vi "Periodic Tasks.vi"(8 "error in":errorcluster) -> ()   [LabVIEW 2016]
doc: "This VI runs in parallel to other tasks. It can contain as many user-defined periodic loops as you need. These can carry out PID or other sorts of timed response."
uses:
  <userlib>/836-libraries/Drive/Drive_Code/Drive_Code_Support/Drive_Code_PID_Bundle.ctl
  <vilib>/Platform/TimedLoop/XDataNode/timing_clust.ctl
  <vilib>/Platform/TimedLoop/XDataNode/nitl_modes.ctl
  <vilib>/Platform/TimedLoop/XDataNode/wakeup.ctl
  Drive Commands.ctl
  Shooting States.ctl
  <vilib>/Rock Robotics/SystemInterfaces/DIO/FPGA_DIOChannel.ctl
  Gear Command.ctl
  TurretStates.ctl
  Control 1.ctl
  TurretImu.ctl
  <vilib>/Rock Robotics/WPI/ThirdParty/CanMotor/TalonSRX/WPI_CANTalonSRX_APIFeedbackSelect.ctl
  FMS Commands.ctl
  <userlib>/836-libraries/Drive/Drive_Code/Drive_Code_Support/Sensor_Cluster.ctl
  <userlib>/836-libraries/Drive/Drive_Code/Drive_Code_Support/Camera_Cluster.ctl
  <userlib>/836-libraries/Drive/Drive_Code/Drive_Code_Support/Drive_Code_Notifier.ctl
  <userlib>/836-libraries/Drive/Drive_Code/Drive_Code_Support/Drive_Code_Command.ctl
  <userlib>/836-libraries/Drive/Drive_Code/Logging_Data.ctl
  <userlib>/836-libraries/Pneumatics/Support_Code/Pneumatics_Command.ctl
  <userlib>/836-libraries/Pneumatics/Support_Code/Pneumatics_Status.ctl
  <userlib>/836-libraries/Pneumatics/Support_Code/Pneumatics_Position.ctl
  <vilib>/Rock Robotics/WPI/Solenoid/WPI_SolenoidDevRef.ctl
  <vilib>/Rock Robotics/WPI/Solenoid/WPI_SolenoidChannel.ctl
  <vilib>/Rock Robotics/WPI/Solenoid/WPI_SolenoidValue.ctl
  <vilib>/Rock Robotics/SystemInterfaces/AI/FPGA_AIChannel.ctl
  <vilib>/Rock Robotics/WPI/DriverStation/WPI_DriverStationRobotMode2.ctl
  MatchTimeNotifications.ctl
  <vilib>/Rock Robotics/WPI/DriverStation/WPI_DriverStationAllianceInfo.ctl
  <vilib>/Analysis/coordinate.llb/Angle Units.ctl
  <vilib>/Analysis/coordinate.llb/Angle Range (Degree).ctl
  <vilib>/Rock Robotics/WPI/ThirdParty/CanMotor/TalonSRX/WPI_CANTalonSRX_APIControlMode.ctl
  <vilib>/Analysis/coordinate.llb/Wrap Angle (scalar).vi
  <vilib>/Rock Robotics/WPI/Utilities/WPI_GetSetVariantRefNum.vi
  <vilib>/addons/control/pid/pid.llb/PID Output Rate Limiter (DBL).vi
  <userlib>/836-libraries/Drive/Drive_Code/Drive_Code_Support/Drive_Loop_Turn_to_Camera.vi
  <userlib>/836-libraries/Drive/Drive_Code/Drive_Code_Support/Drive_Loop_Cheesey_Drive.vi
  <userlib>/836-libraries/Drive/Drive_Code/Drive_Code_Support/Drive_Loop_Turn.vi
  <userlib>/836-libraries/Drive/Drive_Code/Drive_Code_Support/Drive_Loop_Drive_Distance.vi
  <vilib>/addons/control/pid/pid.llb/PID (DBL).vi
  <userlib>/836-libraries/Drive/Drive_Code/Drive_Code_Support/Drive_Loop_Do_Nothing.vi
  <userlib>/836-libraries/Drive/Drive_Code/Drive_Code_Support/Drive_Loop_Follow_Camera.vi
  <userlib>/836-libraries/Drive/Drive_Code/Drive_Code_Support/Drive_Loop_Tank_Drive.vi
  <userlib>/836-libraries/Pneumatics/Support_Code/Pneumatics_Command_Set_Periodic.vi
  <vilib>/Rock Robotics/Network Tables/NT Write Number.vi
  <vilib>/platform/TimedLoop/XDataNode/XDataNode.xnode
  <vilib>/Platform/TimedLoop/XDataNode/XDNodeRunTimeDep.lvlib
  <vilib>/Analysis/NI_AAL_Angle.lvlib
  <vilib>/addons/control/pid/NI_PID_pid.lvlib
  <userlib>/836-libraries/Drive/Drive_Code/Drive_Code_Support/Drive_Loop_Approach_Camera.vi
panel:
  in  "Modulate?":bool
  out "Sensor Loop Duration? 2":i64=6
  out "Sensor Loop Late? 2":bool
  in  "Sensor Loop Period 2":i64=20
  in  "Tab Control":T1(tab)=enum."Sensors"
  in  "Reset S and H":bool
  in  "PID Reset Tolerance":dbl=1.0
  out "PID Response":cluster{dbl, "Double":dbl}(graph)={1.3854228500280215, "Double"=1.3854228500280215}
  in  "Switch Case":i32
  in  "Power 3":dbl=0.4
  in  "Angle 3":dbl=4.0
  in  "Distance":dbl=20.0
  in  "Power in":dbl=0.7
  in  "Angle in":dbl=20.0
  in  "Update PIDS":bool
  in  "Send Command":bool
  in  "PID Gains":T2={"Yaw, Driving Straight"={"proportional gain (Kc)"=0.01, "integral time (Ti, min)"=0.0, "derivative time (Td, min)"=0.0}, "Yaw, Holding Still"={"proportional gain (Kc)"=0.037, "integral time (Ti, min)"=0.01, "derivative time (Td, min)"=0.0}, "Distance, Driving Straight"={"proportional gain (Kc)"=0.035, "integral time (Ti, min)"=0.0, "derivative time (Td, min)"=0.001}, "Distance, Holding Still"={"proportional gain (Kc)"=0.0, "integral time (Ti, min)"=0.0, "derivative time (Td, min)"=0.0}}
  out "Done?":bool=TRUE
  out "Diff":dbl
  out "Motor Out":dbl(graph)
  in  "FMS Reverse Speed":dbl(knob)=-0.44952415089947806
  in  "Offset?":bool
  in  "Feeder Period":dbl
  in  "Feeder Duty Cycle":dbl
  in  "FMS Period":dbl=400.0
  in  "FMS Duty Cycle":dbl=65.0
  in  "FMS Speed":dbl(knob)=0.48612791751281736 scale=0.0..1.0
  in  "Feeder Speed":dbl(knob)=0.8400379461171551 scale=0.0..1.0
  in  "rate":dbl(knob)=501.8694638525026 scale=0.0..1000.0
  in  "TR Period":dbl=400.0
  in  "Transition Roller Duty Cycle":dbl=60.0
  in  "Trans Roller":dbl(knob)=0.6328698265378321 scale=0.0..1.0
  in  "Trans Roller Reverse Speed":dbl(knob)=-0.2732336168714805
  out "Gear Mech Duration":i64=31
  in  "Climb Blocking?":bool
  out "Shooter SM Late?":bool
  out "Shooter SM Duration":i64
  in  "Shooter SM Period":i64=40
  out "Climb Loop Late?":bool
  out "Climb Loop Duration":i64=2
  in  "Climb  Loop Period":i64=40
  out "Gear Manual Late?":bool
  out "Gear Manual Duration":i64
  in  "Gear  Manual Period":i64=40
  out "Homing Sensor Late":bool
  out "Homing Sensor Duration":i64
  in  "Drive Command Period":i64=20
  in  "Intake Period":i64=60
  in  "Intake Blocking?":bool
  in  "Gear Shift Period":i64=100
  in  "NeoPixel Period":i64=100
  in  "NeoPixel Blocking?":bool
  in  "FMS Blocking?":bool
  out "FMS Control Late?":bool
  out "FMS Control Duration":i64
  out "Intake Control Late?":bool
  out "Intake Control Duration":i64=1
  out "Drive Comand Loop Late?":bool
  out "Drive Command Loop Duration":i64=1
  out "Gear Shift Loop Late?":bool
  out "Gear Shift Loop Duration":i64
  out "NeoPixel Loop Late?":bool
  out "NeoPixel Loop Duration":i64
  out "Match Time Loop Late?":bool
  out "Match Time Loop Duration":i64=12
  in  "FMS Period":i64=10
  in  "Match Time Period":i64=100
  in  "Boiler Dist Period":i64=50
  in  "Homing Sensor Period":i64=4
  out "Boiler Dist Late?":bool
  out "Boiler Dist Duration":i64
  out "Top Late?":bool
  in  "Top Period":i64=60
  out "Top Duration":i64=13
  out "Bottom Wheel Late?":bool
  out "Bottom Wheel Duration":i64=12
  in  "Bot Period":i64=60
  out "TurretLate?":bool
  in  "Turret Period":i64=20
  out "Turret Duration":i64=2
  out "Gear Mech Late?":bool
  in  "Gear Mech Period":i64=40
  in  "Home Turret Sensor":bool
  out "Auto Target Lock":bool
  in  "Test LEDS":bool
  out "Turret State":dbl(graph)=2.0
  in  "Feed CW":dbl
  in  "FeedCCW":dbl
  out "Motor Output":dbl=-0.25
  out "Turret":cluster{"Double":dbl, "desired Angle":dbl}(graph)={"Double"=-77.76264505639548, "desired Angle"=-118.0}
  in  "Range for I":dbl=10.0
  in  "Reinitalize?":bool
  in  "Turret Max Speed":dbl(knob)=0.34982498966729664 scale=0.0..1.0
  in  "CW Bound":dbl=110.0
  in  "CCW Bound":dbl=-120.0 format="%#_13g"
  in  "Tab Control 3":T3(tab)
  in  "Min Rate":dbl=0.2
  in  "Lost Target Time?":dbl(knob)=0.5301133241962713 scale=0.0..1.0
  in  "Wait Time in Search":dbl(knob)=0.3769951386039123 scale=0.0..1.0
  in  "Period (ms)":dbl=100.0
  in  "Duty Cycle (%)":dbl=10.0
  in  "Target Range Gains":T4={"proportional gain (Kc)"=0.01, "integral time (Ti, min)"=0.006, "derivative time (Td, min)"=0.0} {"derivative time (Td, min)" format="%.4f"; "integral time (Ti, min)" format="%.8f"; "proportional gain (Kc)" format="%.8f"}
  in  "Target range":cluster{"output high":dbl, "output low":dbl}={"output high"=0.9, "output low"=-0.9}
  in  "Setpoint Tol":dbl=1.5
  in  "Search Gains":T4={"proportional gain (Kc)"=0.018, "integral time (Ti, min)"=0.003, "derivative time (Td, min)"=0.005}
  in  "Search Range":cluster{"output high":dbl, "output low":dbl}={"output high"=0.25, "output low"=-0.25}
  in  "Search Tol":dbl=7.0
  in  "Softstop":dbl=2.0
  in  "Jump to Desired Angle":T4={"proportional gain (Kc)"=0.015, "integral time (Ti, min)"=0.005, "derivative time (Td, min)"=0.6}
  in  "Jump Output":cluster{"output high":dbl, "output low":dbl}={"output high"=0.5, "output low"=-0.5}
  in  "Valid Target Time Guess":dbl(knob)=0.19161068264500253 scale=0.0..1.0
  in  "Switch outer bound delta":dbl=20.0
  in  "Stable Movemt":dbl(knob)=0.11807450406305693 scale=0.0..1.0
  in  "Guess State Time?":u32
  in  "Target Track":bool
  in  "Manual Entry":bool
  in  "Turret Desired":dbl=56.0
  in  "d":dbl=0.41666666666667 format="%#_13g"
  in  "Top Multiplier BLUE":dbl=0.977
  in  "Tab Control 2":enum32{"TBH", "PID(F)"}(tab)=enum."PID(F)"
  in  "P 2":dbl=0.04 format="%#_8g"
  in  "I 2":dbl=0.0003
  in  "D 2":dbl=2.0
  in  "F 2":dbl=0.0132
  in  "I Zone 2":dbl
  in  "Ramp Rate 2":dbl
  in  "Enc Counts 2":dbl=4096.0
  in  "Rev FB Sensor 2":bool=TRUE
  in  "Reverse Closed-Loop Output":bool
  out "State1":i32
  out "Top Response":cluster{"Top Cntrl":dbl, dbl}(graph)={"Top Cntrl"=0.0, -2616.406}
  in  "Reset1":bool
  in  "Len":i16=90
  in  "Trig":dbl=30.0
  in  "Arm":bool
  out "Tgrd":bool
  out "cnt":i16=90
  in  "Top Open":bool
  out "Top Dist":dbl
  in  "Output":dbl(knob) scale=0.0..1.0
  out "Min Top":dbl
  out "Max top":dbl
  in  "reset top":bool
  out "Top Cntrl .":dbl=-2616.406
  in  "Top Tol":dbl=25.0 format="%#_13g"
  out "RPM High":bool=TRUE
  out "RPM Low":bool
  out "1 RPM":bool
  out "5 RPM":bool
  out "2 RPM":bool
  out "8 RPM":bool
  out "7 RPM":bool
  out "6 RPM":bool
  out "4 RPM":bool
  out "3 RPM":bool
  in  "Disable Top":bool
  in  "TopFrontPanelMode?":bool
  in  "Top Cntrl":dbl(knob)=-4212.742512853087 scale=-10000.0..7000.0
  in  "Top Multiplier RED":dbl(knob)=0.9791850874811381 scale=0.0..1.0
  in  "TuneTopPID":bool
  in  "Bottom Multiplier Blue":dbl=0.977
  out "State2":i32
  out "Bot Response":cluster{"Bot Cntrl":dbl, dbl}(graph)
  in  "Reset2":bool
  in  "Len2":i16=90
  in  "Trig2":dbl=40.0
  in  "Arm2":bool
  out "Tgrd 2":bool
  out "cnt 2":i16=90
  out "Bot Dist":dbl
  in  "Ramp Rate 3":dbl
  in  "I Zone 3":dbl
  in  "F 3":dbl=0.0288
  in  "D 3":dbl=7.0
  in  "I 3":dbl=0.001
  in  "P 3":dbl=0.16
  in  "Enc Counts":dbl=4096.0
  in  "Rev FB Sensor":bool=TRUE
  out "Min Bot":dbl
  out "Max Bot":dbl
  in  "reset bot":bool
  out "Bot Cntrl .":dbl
  in  "Open?":bool
  in  "Open Loop Cntrl":dbl(knob)=0.0014346101200435335 scale=-1.0..1.0
  in  "Bot Tol":dbl=25.0 format="%#_13g"
  out "RPM High .":bool
  out "RPM Low .":bool
  out "1 RPM .":bool=TRUE
  out "5 RPM .":bool=TRUE
  out "2 RPM .":bool=TRUE
  out "8 RPM .":bool=TRUE
  out "7 RPM .":bool=TRUE
  out "6 RPM .":bool=TRUE
  out "4 RPM .":bool=TRUE
  out "3 RPM .":bool=TRUE
  in  "Disable Bottom":bool
  in  "BotFrontPanel":bool
  in  "Bot Cntrl":dbl(knob)=1732.3253418662134 scale=0.0..5700.0
  in  "Bottom Multiplier Red":dbl(knob)=0.9795602911750467 scale=0.0..1.0
  in  "TuneBotPID":bool
  in  "Max Buff Size":i32=50
  in  "Eval Period (s)":dbl=0.5
  out "Climb Speed":dbl(knob) scale=0.0..1.0
  in  "Slow Speed":dbl(knob)=0.5025106150572204 scale=0.0..1.0
  in  "Fast Thresh":dbl=90.0
  in  "Slow Thresh":dbl=20.0
  in  "Pitch Roll Switch":bool
  in  "Manual Speed":dbl(knob)=1.0 scale=0.0..1.0
  in  "Intake speed":dbl(knob)=0.7559666744644368 scale=0.0..1.0
  in  "Camera Align Stable":dbl=0.5
  out "Camera Align Done":bool=TRUE
  out "Turn To Camera":cluster{dbl, dbl}(graph)
  in  "Start Score Gear":bool
  in  "Turn To Peg Tol. (deg)":dbl=1.0
  in  "PID Segments (1-500)":dbl=60.0
  in  "Amount of Time (s)":dbl=5.0
  in  "Limit of Orientation Change":dbl=3.0
  out "PlaceGearSpline":cluster{"X":dbl, "Y":dbl}[](graph)=[{"X"=-1.3322676295501878e-15, "Y"=0.0}, {"X"=-0.005175551287835818, "Y"=0.029230486948032965}, {"X"=-0.010309669370175054, "Y"=0.05770879451037929}, {"X"=-0.015402478881982571, "Y"=0.08543795321519669}, {"X"=-0.020454104458221895, "Y"=0.1124209935906429}, {"X"=-0.025464670733856554, "Y"=0.13866094616487562}, {"X"=-0.030434302343850077, "Y"=0.16416084146605264}, {"X"=-0.03536312392316599, "Y"=0.18892371002233163}, {"X"=-0.04025126010676783, "Y"=0.21295258236187029}, {"X"=-0.045098835529619095, "Y"=0.2362504890128264}, {"X"=-0.04990597482668335, "Y"=0.25882046050335766}, {"X"=-0.0546728026329241, "Y"=0.28066552736162176}, {"X"=-0.05939944358330489, "Y"=0.3017887201157765}, {"X"=-0.06408602231278922, "Y"=0.32219306929397956}, {"X"=-0.06873266345634065, "Y"=0.3418816054243887}, {"X"=-0.07333949164892267, "Y"=0.3608573590351616}, {"X"=-0.07790663152549886, "Y"=0.379123360654456}, {"X"=-0.0824342077210327, "Y"=0.3966826408104296}, {"X"=-0.08692234487048774, "Y"=0.41353823003124013}, {"X"=-0.0913711676088275, "Y"=0.4296931588450454}, {"X"=-0.09578080057101551, "Y"=0.44515045778000295}, {"X"=-0.10015136839201531, "Y"=0.45991315736427074}, {"X"=-0.10448299570679041, "Y"=0.4739842881260064}, {"X"=-0.10877580715030434, "Y"=0.4873668805933676}, {"X"=-0.11302992735752064, "Y"=0.500063965294512}, {"X"=-0.11724548096340282, "Y"=0.5120785727575975}, {"X"=-0.12142259260291441, "Y"=0.5234137335107818}, {"X"=-0.12556138691101898, "Y"=0.5340724780822225}, {"X"=-0.12966198852268, "Y"=0.5440578370000774}, {"X"=-0.13372452207286104, "Y"=0.5533728407925042}, {"X"=-0.13774911219652555, "Y"=0.5620205199876606}, {"X"=-0.14173588352863717, "Y"=0.5700039051137045}, {"X"=-0.14568496070415934, "Y"=0.5773260266987934}, {"X"=-0.14959646835805565, "Y"=0.5839899152710851}, {"X"=-0.1534705311252896, "Y"=0.5899986013587375}, {"X"=-0.1573072736408247, "Y"=0.595355115489908}, {"X"=-0.1611068205396245, "Y"=0.6000624881927545}, {"X"=-0.16486929645665252, "Y"=0.6041237499954348}, {"X"=-0.1685948260268723, "Y"=0.6075419314261065}, {"X"=-0.17228353388524736, "Y"=0.6103200630129273}, {"X"=-0.1759355446667412, "Y"=0.6124611752840551}, {"X"=-0.1795509830063174, "Y"=0.6139682987676475}, {"X"=-0.18312997353893945, "Y"=0.6148444639918622}, {"X"=-0.1866726408995709, "Y"=0.615092701484857}, {"X"=-0.19017910972317525, "Y"=0.6147160417747896}, {"X"=-0.19364950464471603, "Y"=0.6137175153898176}, {"X"=-0.1970839502991568, "Y"=0.6121001528580988}, {"X"=-0.20048257132146108, "Y"=0.6098669847077911}, {"X"=-0.20384549234659238, "Y"=0.6070210414670519}, {"X"=-0.20717283800951425, "Y"=0.6035653536640394}, {"X"=-0.21046473294519016, "Y"=0.5995029518269108}, {"X"=-0.21372130178858373, "Y"=0.5948368664838243}, {"X"=-0.2169426691746584, "Y"=0.5895701281629372}, {"X"=-0.22012895973837776, "Y"=0.5837057673924075}, {"X"=-0.2232802981147053, "Y"=0.5772468147003926}, {"X"=-0.22639680893860456, "Y"=0.5701963006150508}, {"X"=-0.22947861684503912, "Y"=0.5625572556645392}, {"X"=-0.2325258464689724, "Y"=0.5543327103770159}, {"X"=-0.235538622445368, "Y"=0.5455256952806385}, {"X"=-0.2385170694091894, "Y"=0.5361392409035648}, {"X"=-0.2414613119954002, "Y"=0.5261763777739528}, {"X"=-0.2443714748389639, "Y"=0.5156401364199595}, {"X"=-0.24724768257484397, "Y"=0.504533547369743}, {"X"=-0.25009005983800403, "Y"=0.4928596411514612}, {"X"=-0.2528987312634075, "Y"=0.4806214482932716}, {"X"=-0.255673821486018, "Y"=0.4678219993233321}, {"X"=-0.25841545514079906, "Y"=0.45446432476980037}, {"X"=-0.26112375686271416, "Y"=0.4405514551608339}, {"X"=-0.26379885128672687, "Y"=0.42608642102459054}, {"X"=-0.2664408630478006, "Y"=0.41107225288922855}, {"X"=-0.269049916780899, "Y"=0.3955119812829047}, {"X"=-0.2716261371209856, "Y"=0.3794086367337775}, {"X"=-0.27416964870302385, "Y"=0.3627652497700043}, {"X"=-0.27668057616197733, "Y"=0.3455848509197428}, {"X"=-0.2791590441328096, "Y"=0.32787047071115094}, {"X"=-0.2816051772504842, "Y"=0.3096251396723863}, {"X"=-0.28401910014996445, "Y"=0.29085188833160647}, {"X"=-0.28640093746621414, "Y"=0.27155374721696923}, {"X"=-0.28875081383419665, "Y"=0.251733746856633}, {"X"=-0.29106885388887554, "Y"=0.23139491777875446}, {"X"=-0.29335518226521434, "Y"=0.2105402905114923}, {"X"=-0.2956099235981766, "Y"=0.18917289558300335}, {"X"=-0.2978332025227258, "Y"=0.16729576352144557}, {"X"=-0.3000251436738256, "Y"=0.1449119248549767}, {"X"=-0.30218587168643934, "Y"=0.12202441011175486}, {"X"=-0.30431551119553063, "Y"=0.09863624981993736}, {"X"=-0.306414186836063, "Y"=0.07475047450768234}, {"X"=-0.30848202324300006, "Y"=0.05037011470314714}, {"X"=-0.3105191450513051, "Y"=0.025498200934489852}, {"X"=-0.3125256768959419, "Y"=0.00013776372986783157}, {"X"=-0.3145017434118739, "Y"=-0.025708166382561206}, {"X"=-0.3164474692340646, "Y"=-0.052036558874639136}, {"X"=-0.31836297899747756, "Y"=-0.07884438321820904}, {"X"=-0.3202483973370763, "Y"=-0.10612860888511239}, {"X"=-0.3221038488878243, "Y"=-0.13388620534719187}, {"X"=-0.3239294582846852, "Y"=-0.16211414207628932}, {"X"=-0.3257253501626224, "Y"=-0.19080938854424706}, {"X"=-0.3274916491565995, "Y"=-0.21996891422290815}, {"X"=-0.32922847990158005, "Y"=-0.24958968858411407}, {"X"=-0.33093596703252753, "Y"=-0.2796686810997075}, {"X"=-0.3326142351844054, "Y"=-0.3102028612415302}, {"X"=-0.3342634089921774, "Y"=-0.3411891984814255}, {"X"=-0.33588361309080683, "Y"=-0.3726246622912342}, {"X"=-0.33747497211525734, "Y"=-0.40450622214280046}, {"X"=-0.3390376107004925, "Y"=-0.4368308475079642}, {"X"=-0.3405716534814756, "Y"=-0.4695955078585701}, {"X"=-0.34207722509317046, "Y"=-0.5027971726664584}, {"X"=-0.34355445017054037, "Y"=-0.5364328114034724}, {"X"=-0.3450034533485491, "Y"=-0.5704993935414542}, {"X"=-0.34642435926216003, "Y"=-0.604993888552246}, {"X"=-0.34781729254633664, "Y"=-0.639913265907691}, {"X"=-0.3491823778360426, "Y"=-0.6752544950796302}, {"X"=-0.35051973976624134, "Y"=-0.7110145455399067}, {"X"=-0.3518295029718964, "Y"=-0.747190386760362}, {"X"=-0.35311179208797133, "Y"=-0.7837789882128385}, {"X"=-0.35436673174942956, "Y"=-0.8207773193691789}, {"X"=-0.3555944465912348, "Y"=-0.8581823497012261}, {"X"=-0.3567950612483505, "Y"=-0.8959910486808206}, {"X"=-0.35796870035574, "Y"=-0.9342003857798058}, {"X"=-0.35911548854836717, "Y"=-0.9728073304700249}, {"X"=-0.3602355504611953, "Y"=-1.011808852223318}, {"X"=-0.361329010729188, "Y"=-1.05120192051153}, {"X"=-0.36239599398730876, "Y"=-1.0909835048065}, {"X"=-0.3634366248705212, "Y"=-1.1311505745800736}, {"X"=-0.36445102801378865, "Y"=-1.1717000993040902}, {"X"=-0.36543932805207485, "Y"=-1.2126290484503932}, {"X"=-0.3664016496203432, "Y"=-1.2539343914908254}, {"X"=-0.36733811735355737, "Y"=-1.2956130978972293}, {"X"=-0.36824885588668066, "Y"=-1.3376621371414452}, {"X"=-0.3691339898546767, "Y"=-1.380078478695317}, {"X"=-0.3699936438925091, "Y"=-1.4228590920306878}, {"X"=-0.37082794263514135, "Y"=-1.4660009466193986}, {"X"=-0.3716370107175369, "Y"=-1.5095010119332912}, {"X"=-0.3724209727746594, "Y"=-1.5533562574442086}, {"X"=-0.3731799534414723, "Y"=-1.5975636526239934}, {"X"=-0.37391407735293913, "Y"=-1.6421201669444871}, {"X"=-0.37462346914402334, "Y"=-1.6870227698775333}, {"X"=-0.3753082534496887, "Y"=-1.7322684308949718}, {"X"=-0.3759685549048985, "Y"=-1.7778541194686481}, {"X"=-0.37660449814461633, "Y"=-1.8237768050704015}, {"X"=-0.3772162078038058, "Y"=-1.8700334571720758}, {"X"=-0.37780380851743034, "Y"=-1.9166210452455135}, {"X"=-0.37836742492045355, "Y"=-1.9635365387625552}, {"X"=-0.3789071816478389, "Y"=-2.010776907195046}, {"X"=-0.37942320333454993, "Y"=-2.0583391200148253}, {"X"=-0.3799156146155501, "Y"=-2.106220146693737}, {"X"=-0.3803845401258031, "Y"=-2.154416956703623}, {"X"=-0.3808301045002724, "Y"=-2.202926519516326}, {"X"=-0.3812524323739214, "Y"=-2.251745804603687}, {"X"=-0.3816516483817139, "Y"=-2.30087178143755}, {"X"=-0.3820278771586131, "Y"=-2.350301419489756}, {"X"=-0.3823812433395826, "Y"=-2.4000316882321475}, {"X"=-0.38271187155958625, "Y"=-2.4500595571365675}, {"X"=-0.38301988645358725, "Y"=-2.5003819956748576}, {"X"=-0.38330541265654916, "Y"=-2.5509959733188605}, {"X"=-0.3835685748034356, "Y"=-2.601898459540417}, {"X"=-0.38380949752921, "Y"=-2.6530864238113727}, {"X"=-0.38402830546883615, "Y"=-2.7045568356035647}, {"X"=-0.38422512325727726, "Y"=-2.7563066643888416}, {"X"=-0.38440007552949684, "Y"=-2.80833287963904}, {"X"=-0.3845532869204587, "Y"=-2.8606324508260057}, {"X"=-0.3846848820651262, "Y"=-2.9132023474215805}, {"X"=-0.38479498559846287, "Y"=-2.966039538897604}, {"X"=-0.3848837221554322, "Y"=-3.0191409947259205}, {"X"=-0.3849512163709979, "Y"=-3.0725036843783733}, {"X"=-0.38499759288012336, "Y"=-3.126124577326804}, {"X"=-0.38502297631777205, "Y"=-3.180000643043055}, {"X"=-0.3850274913189075, "Y"=-3.2341288509989683}, {"X"=-0.3850112625184935, "Y"=-3.2885061706663827}, {"X"=-0.38497441455149317, "Y"=-3.343129571517146}, {"X"=-0.3849170720528703, "Y"=-3.397996023023098}, {"X"=-0.3848393596575885, "Y"=-3.45310249465608}, {"X"=-0.384741402000611, "Y"=-3.508445955887938}, {"X"=-0.3846233237169017, "Y"=-3.5640233761905113}, {"X"=-0.38448524944142376, "Y"=-3.6198317250356418}, {"X"=-0.38432730380914093, "Y"=-3.6758679718951726}, {"X"=-0.38414961145501664, "Y"=-3.7321290862409464}, {"X"=-0.38395229701401445, "Y"=-3.7886120375448047}, {"X"=-0.3837354851210979, "Y"=-3.8453137952785914}, {"X"=-0.38349930041123054, "Y"=-3.9022313289141453}, {"X"=-0.38324386751937584, "Y"=-3.9593616079233116}, {"X"=-0.3829693110804973, "Y"=-4.016701601777932}, {"X"=-0.3826757557295587, "Y"=-4.074248279949847}, {"X"=-0.3823633261015231, "Y"=-4.1319986119109045}, {"X"=-0.3820321468313545, "Y"=-4.189949567132939}, {"X"=-0.3816823425540162, "Y"=-4.248098115087799}, {"X"=-0.38131403790447166, "Y"=-4.306441225247323}, {"X"=-0.38092735751768453, "Y"=-4.364975867083354}, {"X"=-0.38052242602861835, "Y"=-4.423699010067736}, {"X"=-0.38009936807223665, "Y"=-4.482607623672311}, {"X"=-0.3796583082835028, "Y"=-4.5416986773689185}, {"X"=-0.3791993712973804, "Y"=-4.600969140629405}, {"X"=-0.3787226817488333, "Y"=-4.660415982925608}, {"X"=-0.37822836427282447, "Y"=-4.7200361737293735}, {"X"=-0.3777165435043178, "Y"=-4.779826682512543}, {"X"=-0.3771873440782768, "Y"=-4.8397844787469575}, {"X"=-0.3766408906296649, "Y"=-4.8999065319044615}, {"X"=-0.3760773077934456, "Y"=-4.960189811456894}, {"X"=-0.37549672020458247, "Y"=-5.0206312868761}, {"X"=-0.3748992524980391, "Y"=-5.08122792763392}, {"X"=-0.37428502930877905, "Y"=-5.141976703202198}, {"X"=-0.37365417527176553, "Y"=-5.2028745830527745}, {"X"=-0.37300681502196265, "Y"=-5.263918536657495}, {"X"=-0.3723430731943333, "Y"=-5.325105533488195}, {"X"=-0.3716630744238415, "Y"=-5.386432543016726}, {"X"=-0.3709669433454505, "Y"=-5.447896534714923}, {"X"=-0.3702548045941239, "Y"=-5.509494478054634}, {"X"=-0.3695267828048253, "Y"=-5.571223342507692}, {"X"=-0.368783002612518, "Y"=-5.6330800975459505}, {"X"=-0.3680235886521659, "Y"=-5.695061712641247}, {"X"=-0.36724866555873226, "Y"=-5.757165157265423}, {"X"=-0.36645835796718046, "Y"=-5.819387400890318}, {"X"=-0.36565279051247446, "Y"=-5.88172541298778}, {"X"=-0.36483208782957754, "Y"=-5.94417616302965}, {"X"=-0.36399637455345324, "Y"=-6.006736620487765}, {"X"=-0.363145775319065, "Y"=-6.069403754833974}, {"X"=-0.3622804147613765, "Y"=-6.132174535540118}, {"X"=-0.36140041751535124, "Y"=-6.195045932078035}, {"X"=-0.3605059082159527, "Y"=-6.25801491391957}, {"X"=-0.35959701149814455, "Y"=-6.321078450536566}, {"X"=-0.35867385199689006, "Y"=-6.3842335114008675}, {"X"=-0.35773655434715285, "Y"=-6.4474770659843115}, {"X"=-0.3567852431838966, "Y"=-6.510806083758742}, {"X"=-0.35582004314208476, "Y"=-6.574217534196006}, {"X"=-0.3548410788566807, "Y"=-6.637708386767938}, {"X"=-0.35384847496264815, "Y"=-6.701275610946384}, {"X"=-0.3528423560949506, "Y"=-6.764916176203185}, {"X"=-0.35182284688855153, "Y"=-6.828627052010189}, {"X"=-0.3507900719784143, "Y"=-6.892405207839234}, {"X"=-0.34974415599950287, "Y"=-6.956247613162157}, {"X"=-0.3486852235867804, "Y"=-7.0201512374508095}, {"X"=-0.3476133993752105, "Y"=-7.08411305017703}, {"X"=-0.3465288079997568, "Y"=-7.148130020812661}, {"X"=-0.34543157409538267, "Y"=-7.212199118829539}, {"X"=-0.3443218222970517, "Y"=-7.276317313699517}, {"X"=-0.34319967723972755, "Y"=-7.34048157489443}, {"X"=-0.3420652635583737, "Y"=-7.40468887188612}, {"X"=-0.34091870588795353, "Y"=-7.468936174146434}, {"X"=-0.33976012886343054, "Y"=-7.533220451147211}, {"X"=-0.33858965711976835, "Y"=-7.5975386723602965}, {"X"=-0.3374074152919309, "Y"=-7.661887807257524}, {"X"=-0.33621352801488097, "Y"=-7.726264825310746}, {"X"=-0.33500811992358265, "Y"=-7.790666695991799}, {"X"=-0.333791315652999, "Y"=-7.85509038877253}, {"X"=-0.3325632398380941, "Y"=-7.9195328731247745}, {"X"=-0.331324017113831, "Y"=-7.983991118520381}, {"X"=-0.33007377211517336, "Y"=-8.048462094431192}, {"X"=-0.3288126294770851, "Y"=-8.112942770329042}, {"X"=-0.32754071383452915, "Y"=-8.17743011568578}, {"X"=-0.32625814982246937, "Y"=-8.241921099973249}, {"X"=-0.32496506207586906, "Y"=-8.30641269266329}, {"X"=-0.323661575229692, "Y"=-8.370901863227738}, {"X"=-0.3223478139189018, "Y"=-8.435385581138448}, {"X"=-0.32102390277846155, "Y"=-8.499860815867253}, {"X"=-0.3196899664433352, "Y"=-8.564324536885996}, {"X"=-0.3183461295484862, "Y"=-8.628773713666524}, {"X"=-0.3169925167288777, "Y"=-8.693205315680675}, {"X"=-0.3156292526194739, "Y"=-8.757616312400293}, {"X"=-0.31425646185523765, "Y"=-8.822003673297218}, {"X"=-0.31287426907113297, "Y"=-8.886364367843301}, {"X"=-0.311482798902123, "Y"=-8.95069536551037}, {"X"=-0.31008217598317167, "Y"=-9.01499363577028}, {"X"=-0.30867252494924224, "Y"=-9.079256148094865}, {"X"=-0.3072539704352981, "Y"=-9.143479871955975}, {"X"=-0.30582663707630325, "Y"=-9.207661776825447}, {"X"=-0.3043906495072209, "Y"=-9.271798832175124}, {"X"=-0.3029461323630145, "Y"=-9.335888007476845}, {"X"=-0.30149321027864767, "Y"=-9.399926272202459}, {"X"=-0.30003200788908413, "Y"=-9.463910595823805}, {"X"=-0.2985626498292871, "Y"=-9.52783794781272}, {"X"=-0.29708526073422026, "Y"=-9.591705297641058}, {"X"=-0.2955999652388472, "Y"=-9.655509614780653}, {"X"=-0.2941068879781315, "Y"=-9.719247868703347}, {"X"=-0.2926061535870363, "Y"=-9.782917028880986}, {"X"=-0.29109788670052555, "Y"=-9.846514064785406}, {"X"=-0.2895822119535627, "Y"=-9.910035945888461}, {"X"=-0.28805925398111104, "Y"=-9.973479641661982}, {"X"=-0.28652913741813424, "Y"=-10.036842121577815}, {"X"=-0.28499198689959604, "Y"=-10.100120355107805}, {"X"=-0.28344792706045957, "Y"=-10.16331131172379}, {"X"=-0.28189708253568857, "Y"=-10.226411960897615}, {"X"=-0.2803395779602467, "Y"=-10.289419272101119}, {"X"=-0.2787755379690973, "Y"=-10.35233021480615}, {"X"=-0.27720508719720394, "Y"=-10.41514175848455}, {"X"=-0.27562835027953, "Y"=-10.477850872608153}, {"X"=-0.27404545185103946, "Y"=-10.540454526648807}, {"X"=-0.27245651654669517, "Y"=-10.602949690078358}, {"X"=-0.2708616690014613, "Y"=-10.665333332368643}, {"X"=-0.2692610338503012, "Y"=-10.7276024229915}, {"X"=-0.2676547357281783, "Y"=-10.789753931418783}, {"X"=-0.2660428992700557, "Y"=-10.851784827122327}, {"X"=-0.2644256491108978, "Y"=-10.913692079573972}, {"X"=-0.26280310988566763, "Y"=-10.975472658245566}, {"X"=-0.26117540622932855, "Y"=-11.037123532608947}, {"X"=-0.2595426627768445, "Y"=-11.09864167213596}, {"X"=-0.25790500416317885, "Y"=-11.160024046298442}, {"X"=-0.2562625550232951, "Y"=-11.221267624568247}, {"X"=-0.2546154399921567, "Y"=-11.282369376417204}, {"X"=-0.252963783704727, "Y"=-11.343326271317165}, {"X"=-0.2513077107959704, "Y"=-11.404135278739968}, {"X"=-0.24964734590084944, "Y"=-11.464793368157455}, {"X"=-0.2479828136543278, "Y"=-11.52529750904147}, {"X"=-0.2463142386913698, "Y"=-11.585644670863852}, {"X"=-0.24464174564693825, "Y"=-11.645831823096449}, {"X"=-0.24296545915599654, "Y"=-11.705855935211098}, {"X"=-0.24128550385350844, "Y"=-11.765713976679645}, {"X"=-0.23960200437443793, "Y"=-11.825402916973927}, {"X"=-0.23791508535374778, "Y"=-11.88491972556579}, {"X"=-0.23622487142640178, "Y"=-11.94426137192708}, {"X"=-0.23453148722736403, "Y"=-12.003424825529631}, {"X"=-0.23283505739159727, "Y"=-12.062407055845293}, {"X"=-0.23113570655406515, "Y"=-12.1212050323459}, {"X"=-0.22943355934973164, "Y"=-12.179815724503301}, {"X"=-0.22772874041356025, "Y"=-12.238236101789335}, {"X"=-0.22602137438051392, "Y"=-12.296463133675848}, {"X"=-0.22431158588555627, "Y"=-12.354493789634677}, {"X"=-0.22259949956365152, "Y"=-12.412325039137672}, {"X"=-0.2208852400497627, "Y"=-12.469953851656664}, {"X"=-0.21916893197885315, "Y"=-12.527377196663506}, {"X"=-0.21745069998588676, "Y"=-12.58459204363004}, {"X"=-0.21573066870582738, "Y"=-12.641595362028095}, {"X"=-0.21400896277363754, "Y"=-12.698384121329529}, {"X"=-0.21228570682428127, "Y"=-12.75495529100618}, {"X"=-0.21056102549272243, "Y"=-12.811305840529883}, {"X"=-0.20883504341392417, "Y"=-12.867432739372484}, {"X"=-0.2071078852228501, "Y"=-12.923332957005833}, {"X"=-0.20537967555446385, "Y"=-12.97900346290176}, {"X"=-0.203650539043729, "Y"=-13.034441226532115}, {"X"=-0.20192060032560866, "Y"=-13.08964321736874}, {"X"=-0.2001899840350666, "Y"=-13.144606404883472}, {"X"=-0.1984588148070667, "Y"=-13.199327758548161}, {"X"=-0.19672721727657208, "Y"=-13.25380424783464}, {"X"=-0.19499531607854595, "Y"=-13.308032842214763}, {"X"=-0.1932632358479527, "Y"=-13.362010511160365}, {"X"=-0.19153110121975558, "Y"=-13.41573422414328}, {"X"=-0.18979903682891727, "Y"=-13.469200950635372}, {"X"=-0.1880671673104025, "Y"=-13.52240766010846}, {"X"=-0.1863356172991742, "Y"=-13.575351322034404}, {"X"=-0.1846045114301957, "Y"=-13.628028905885039}, {"X"=-0.18287397433843108, "Y"=-13.680437381132203}, {"X"=-0.18114413065884355, "Y"=-13.732573717247746}, {"X"=-0.1794151050263968, "Y"=-13.78443488370351}, {"X"=-0.17768702207605375, "Y"=-13.836017849971327}, {"X"=-0.17596000644277893, "Y"=-13.887319585523052}, {"X"=-0.1742341827615353, "Y"=-13.938337059830522}, {"X"=-0.17250967566728595, "Y"=-13.98906724236558}, {"X"=-0.1707866097949952, "Y"=-14.03950710260006}, {"X"=-0.16906510977962638, "Y"=-14.089653610005817}, {"X"=-0.16734530025614305, "Y"=-14.139503734054685}, {"X"=-0.16562730585950813, "Y"=-14.189054444218513}, {"X"=-0.16391125122468575, "Y"=-14.238302709969137}, {"X"=-0.16219726098663942, "Y"=-14.287245500778404}, {"X"=-0.16048545978033246, "Y"=-14.33587978611815}, {"X"=-0.1587759722407284, "Y"=-14.384202535460224}, {"X"=-0.1570689230027912, "Y"=-14.432210718276467}, {"X"=-0.1553644367014836, "Y"=-14.479901304038721}, {"X"=-0.15366263797176946, "Y"=-14.527271262218823}, {"X"=-0.15196365144861312, "Y"=-14.57431756228862}, {"X"=-0.15026760176697715, "Y"=-14.621037173719955}, {"X"=-0.14857461356182508, "Y"=-14.66742706598467}, {"X"=-0.1468848114681206, "Y"=-14.713484208554602}, {"X"=-0.14519832012082784, "Y"=-14.759205570901601}, {"X"=-0.14351526415490917, "Y"=-14.804588122497506}, {"X"=-0.14183576820532887, "Y"=-14.849628832814162}, {"X"=-0.1401599569070511, "Y"=-14.894324671323403}, {"X"=-0.13848795489503815, "Y"=-14.938672607497079}, {"X"=-0.1368198868042538, "Y"=-14.982669610807028}, {"X"=-0.13515587726966194, "Y"=-15.026312650725098}, {"X"=-0.13349605092622652, "Y"=-15.069598696723121}, {"X"=-0.13184053240890983, "Y"=-15.112524718272955}, {"X"=-0.13018944635267604, "Y"=-15.155087684846423}, {"X"=-0.12854291739248927, "Y"=-15.197284565915384}, {"X"=-0.12690107016331262, "Y"=-15.239112330951672}, {"X"=-0.12526402930010905, "Y"=-15.280567949427132}, {"X"=-0.12363191943784245, "Y"=-15.3216483908136}, {"X"=-0.12200486521147699, "Y"=-15.362350624582929}, {"X"=-0.12038299125597518, "Y"=-15.402671620206954}, {"X"=-0.11876642220630095, "Y"=-15.442608347157519}, {"X"=-0.11715528269741823, "Y"=-15.482157774906463}, {"X"=-0.11554969736429012, "Y"=-15.521316872925636}, {"X"=-0.11394979084187998, "Y"=-15.560082610686873}, {"X"=-0.11235568776515194, "Y"=-15.59845195766202}, {"X"=-0.11076751276906933, "Y"=-15.63642188332292}, {"X"=-0.10918539048859523, "Y"=-15.67398935714141}, {"X"=-0.10760944555869341, "Y"=-15.711151348589336}, {"X"=-0.10603980261432781, "Y"=-15.747904827138544}, {"X"=-0.10447658629046132, "Y"=-15.784246762260869}, {"X"=-0.10291992122205768, "Y"=-15.820174123428162}, {"X"=-0.10136993204408083, "Y"=-15.855683880112256}, {"X"=-0.09982674339149392, "Y"=-15.890773001784996}, {"X"=-0.0982904798992604, "Y"=-15.92543845791823}, {"X"=-0.09676126620234365, "Y"=-15.959677217983792}, {"X"=-0.09523922693570781, "Y"=-15.993486251453527}, {"X"=-0.09372448673431621, "Y"=-16.02686252779928}, {"X"=-0.0922171702331315, "Y"=-16.059803016492893}, {"X"=-0.09071740206711873, "Y"=-16.092304687006205}, {"X"=-0.08922530687124056, "Y"=-16.124364508811063}, {"X"=-0.08774100928046007, "Y"=-16.155979451379302}, {"X"=-0.08626463392974146, "Y"=-16.18714648418277}, {"X"=-0.08479630545404825, "Y"=-16.217862576693314}, {"X"=-0.08333614848834417, "Y"=-16.248124698382764}, {"X"=-0.0818842876675919, "Y"=-16.27792981872297}, {"X"=-0.08044084762675562, "Y"=-16.307274907185768}, {"X"=-0.07900595300079885, "Y"=-16.33615693324301}, {"X"=-0.0775797284246849, "Y"=-16.364572866366533}, {"X"=-0.07616229853337729, "Y"=-16.392519676028186}, {"X"=-0.07475378796183998, "Y"=-16.41999433169979}, {"X"=-0.07335432134503587, "Y"=-16.446993802853214}, {"X"=-0.07196402331792846, "Y"=-16.473515058960288}, {"X"=-0.07058301851548174, "Y"=-16.499555069492853}, {"X"=-0.06921143157265922, "Y"=-16.525110803922747}, {"X"=-0.06784938712442444, "Y"=-16.550179231721824}, {"X"=-0.06649700980574047, "Y"=-16.574757322361922}, {"X"=-0.0651544242515713, "Y"=-16.598842045314882}, {"X"=-0.06382175509688041, "Y"=-16.622430370052538}, {"X"=-0.06249912697663142, "Y"=-16.64551926604675}, {"X"=-0.06118666452578733, "Y"=-16.668105702769346}, {"X"=-0.05988449237931215, "Y"=-16.69018664969218}, {"X"=-0.05859273517216894, "Y"=-16.711759076287073}, {"X"=-0.0573115175393217, "Y"=-16.732819952025892}, {"X"=-0.05604096411573394, "Y"=-16.75336624638047}, {"X"=-0.05478119953636872, "Y"=-16.773394928822643}, {"X"=-0.053532348436190064, "Y"=-16.792902968824254}, {"X"=-0.05229453545016148, "Y"=-16.811887335857158}, {"X"=-0.051067885213246504, "Y"=-16.83034499939319}, {"X"=-0.049852522360408186, "Y"=-16.84827292890419}, {"X"=-0.04864857152661052, "Y"=-16.865668093861995}, {"X"=-0.047456157346816574, "Y"=-16.88252746373846}, {"X"=-0.04627540445599081, "Y"=-16.89884800800542}, {"X"=-0.04510643748909582, "Y"=-16.914626696134714}, {"X"=-0.043949381081095605, "Y"=-16.929860497598185}, {"X"=-0.04280435986695321, "Y"=-16.94454638186769}, {"X"=-0.041671498481632645, "Y"=-16.958681318415056}, {"X"=-0.04055092156009695, "Y"=-16.972262276712133}, {"X"=-0.039442753737310626, "Y"=-16.985286226230752}, {"X"=-0.03834711964823623, "Y"=-16.997750136442765}, {"X"=-0.037264143927837765, "Y"=-17.009650976820016}, {"X"=-0.036193951211078296, "Y"=-17.020985716834343}, {"X"=-0.035136666132921816, "Y"=-17.03175132595758}, {"X"=-0.034092413328331864, "Y"=-17.041944773661587}, {"X"=-0.033061317432271475, "Y"=-17.051563029418197}, {"X"=-0.03204350307970467, "Y"=-17.060603062699254}, {"X"=-0.031039094905594967, "Y"=-17.069061842976588}, {"X"=-0.0300482175449059, "Y"=-17.076936339722064}, {"X"=-0.02907099563260051, "Y"=-17.084223522407505}, {"X"=-0.028107553803642812, "Y"=-17.090920360504768}, {"X"=-0.02715801669299584, "Y"=-17.09702382348569}, {"X"=-0.026222508935623622, "Y"=-17.102530880822094}, {"X"=-0.025301155166489675, "Y"=-17.107438501985854}, {"X"=-0.024394080020557537, "Y"=-17.111743656448795}, {"X"=-0.023501408132790225, "Y"=-17.115443313682764}, {"X"=-0.022623264138151782, "Y"=-17.11853444315959}, {"X"=-0.02175977267160573, "Y"=-17.12101401435114}, {"X"=-0.02091105836811509, "Y"=-17.122878996729238}, {"X"=-0.020077245862643898, "Y"=-17.124126359765736}, {"X"=-0.019258459790155676, "Y"=-17.124753072932457}, {"X"=-0.018454824785613454, "Y"=-17.12475610570127}, {"X"=-0.01766646548398126, "Y"=-17.124132427544005}, {"X"=-0.01689350652022211, "Y"=-17.122879007932504}, {"X"=-0.016136072529300563, "Y"=-17.120992816338603}, {"X"=-0.015394288146179118, "Y"=-17.118470822234155}, {"X"=-0.014668278005821815, "Y"=-17.115309995091}, {"X"=-0.01395816674319167, "Y"=-17.11150730438098}, {"X"=-0.013264078993252723, "Y"=-17.107059719575922}, {"X"=-0.012586139390968502, "Y"=-17.101964210147695}, {"X"=-0.011924472571302018, "Y"=-17.096217745568126}, {"X"=-0.011279203169217317, "Y"=-17.08981729530906}, {"X"=-0.01065045581967793, "Y"=-17.08275982884233}, {"X"=-0.010038355157647378, "Y"=-17.0750423156398}, {"X"=-0.009443025818088676, "Y"=-17.066661725173294}, {"X"=-0.008864592435965346, "Y"=-17.05761502691466}, {"X"=-0.00830317964624196, "Y"=-17.047899190335734}, {"X"=-0.007758912083881002, "Y"=-17.03751118490837}, {"X"=-0.007231914383846523, "Y"=-17.026447980104404}, {"X"=-0.006722311181102053, "Y"=-17.014706545395683}, {"X"=-0.0062302271106105915, "Y"=-17.00228385025403}, {"X"=-0.005755786807336192, "Y"=-16.989176864151318}, {"X"=-0.005299114906242386, "Y"=-16.975382556559367}, {"X"=-0.004860336042292169, "Y"=-16.96089789695003}, {"X"=-0.0044395748504496, "Y"=-16.945719854795133}, {"X"=-0.004036955965678205, "Y"=-16.929845399566542}, {"X"=-0.003652604022940982, "Y"=-16.913271500736084}, {"X"=-0.00328664365720199, "Y"=-16.89599512777561}, {"X"=-0.002939199503424759, "Y"=-16.878013250156947}, {"X"=-0.002610396196572278, "Y"=-16.859322837351954}, {"X"=-0.002300358371608614, "Y"=-16.839920858832468}, {"X"=-0.0020092106634972936, "Y"=-16.81980428407033}, {"X"=-0.001737077707201305, "Y"=-16.79897008253737}, {"X"=-0.0014840841376847168, "Y"=-16.777415223705454}, {"X"=-0.0012503545899110572, "Y"=-16.755136677046416}, {"X"=-0.0010360136988438553, "Y"=-16.732131412032093}, {"X"=-0.0008411860994460935, "Y"=-16.708396398134315}, {"X"=-0.0006659964266818446, "Y"=-16.683928604824953}, {"X"=-0.0005105693155140889, "Y"=-16.658725001575835}, {"X"=-0.0003750294009069016, "Y"=-16.632782557858803}, {"X"=-0.0002595013178238114, "Y"=-16.606098243145688}, {"X"=-0.00016410970122834715, "Y"=-16.578669026908354}, {"X"=-8.897918608348467e-05, "Y"=-16.550491878618633}, {"X"=-3.4234407353303444e-05, "Y"=-16.52156376774837}, {"X"=-1.3322676295501878e-15, "Y"=-16.491881663769405}]
  in  "Done?":bool
  out "Arc Length Chart":cluster{dbl, "setpoint":dbl}(graph)={41.98750750000001, "setpoint"=43.85178169819717}
  in  "Steer Range":cluster{"output high":dbl, "output low":dbl}={"output high"=1.0, "output low"=-1.0} {"output low" format="%.2f"; "output high" format="%.2f"}
  in  "PID Steer gains":T4={"proportional gain (Kc)"=7.0, "integral time (Ti, min)"=0.0, "derivative time (Td, min)"=1e-06} {"derivative time (Td, min)" format="%.3f"; "integral time (Ti, min)" format="%.4f"; "proportional gain (Kc)" format="%.3f"}
  out "steer":dbl=-1.0 format="%.2f"
  out "throttle":dbl=-0.14914193585577323 format="%.2f"
  in  "Speed Range":cluster{"output high":dbl, "output low":dbl}={"output high"=0.8, "output low"=-0.8} {"output low" format="%.2f"; "output high" format="%.2f"}
  in  "PID Speed gains":T4={"proportional gain (Kc)"=0.08, "integral time (Ti, min)"=0.0, "derivative time (Td, min)"=0.0} {"derivative time (Td, min)" format="%.3f"; "integral time (Ti, min)" format="%.3f"; "proportional gain (Kc)" format="%.3f"}
  out "Angle Chart (rad)":cluster{"Yaw Wind":dbl, "setpoint":dbl}(graph)={"Yaw Wind"=1.3285812927941276, "setpoint"=1.4723179878791584}
  in  "Power Place Gear  2":dbl=0.4
  in  "Offset APpr 2":dbl=-4.0
  in  "Invert Angle":bool
  in  "Initial dAngle":dbl=10.0
  out "Gear Delivery Graphs":cluster{"Double":dbl, "Double":dbl}(graph)={"Double"=137.66732472410789, "Double"=126.6012025}
  in  "Gear Place gains":T4={"proportional gain (Kc)"=0.01, "integral time (Ti, min)"=0.0, "derivative time (Td, min)"=0.005} {"derivative time (Td, min)" format="%.3f"; "integral time (Ti, min)" format="%.3f"; "proportional gain (Kc)" format="%.3f"}
  in  "output range":cluster{"output high":dbl, "output low":dbl}={"output high"=0.5, "output low"=-0.5} {"output low" format="%.2f"; "output high" format="%.2f"}
  in  "Offset":dbl=6.0
  out "Save Drive 2":bool
  in  "Burst":i32=75
  out "Save Drive":bool
  in  "loop period (ms) 2":u32=200
  in  "Log to USB?":bool=TRUE
  in  "TDMS Name":string
  in  "Numeric":dbl
  out "Hit Peg":bool
  out "Accel Z":dbl(graph)
  out "Accel Y":dbl(graph)
  out "Bot Dist .":dbl
  out "Top Dist .":dbl
  out "Bottom Wheel Graph":cluster{"Bot Cntrl":dbl, dbl}(graph)
  out "Top Response 2":cluster{"Top Cntrl":dbl, dbl}(graph)={"Top Cntrl"=0.0, -2972.7832571721456}
  out "Good Pri.":bool=TRUE
  out "Pitch Body 2":dbl=-0.056920261793436566
  out "Roll Body 2":dbl=0.6690482686994529
  out "Yaw Body 2":dbl=1.3854228500280215
  out "S 5":T5={"Boolean"=FALSE, "Boolean 2"=FALSE, "Boolean 3"=FALSE, "Boolean 4"=TRUE}
  out "G 5":T5={"Boolean"=TRUE, "Boolean 2"=FALSE, "Boolean 3"=FALSE, "Boolean 4"=FALSE}
  out "A 5":T5={"Boolean"=TRUE, "Boolean 2"=FALSE, "Boolean 3"=FALSE, "Boolean 4"=FALSE}
  out "M 5":T5={"Boolean"=FALSE, "Boolean 2"=FALSE, "Boolean 3"=FALSE, "Boolean 4"=TRUE}
  out "Good Pri 2":bool=TRUE
  out "Good BU 3":bool=TRUE
  out "Pitch Turret 2":dbl=-0.028041453986879628
  out "Roll Turret 2":dbl=-0.028238181631991988
  in  "ReOpen IMUs 2":bool
  out "Occupant Pri 2":u8[](array[numeric])=[160] format="%02x"
  out "Odd Pri 2":bool
  out "Odd Alt 2":bool
  out "Occupant Alt 2":u8[](array[numeric])=[160] format="%02x"
  out "S 6":T5={"Boolean"=FALSE, "Boolean 2"=FALSE, "Boolean 3"=FALSE, "Boolean 4"=TRUE}
  out "G 6":T5={"Boolean"=TRUE, "Boolean 2"=FALSE, "Boolean 3"=FALSE, "Boolean 4"=FALSE}
  out "A 6":T5={"Boolean"=TRUE, "Boolean 2"=FALSE, "Boolean 3"=FALSE, "Boolean 4"=FALSE}
  out "M 6":T5={"Boolean"=FALSE, "Boolean 2"=FALSE, "Boolean 3"=FALSE, "Boolean 4"=TRUE}
  out "S 7":T5={"Boolean"=FALSE, "Boolean 2"=FALSE, "Boolean 3"=FALSE, "Boolean 4"=TRUE}
  out "G 7":T5={"Boolean"=TRUE, "Boolean 2"=FALSE, "Boolean 3"=FALSE, "Boolean 4"=FALSE}
  out "A 7":T5={"Boolean"=TRUE, "Boolean 2"=FALSE, "Boolean 3"=FALSE, "Boolean 4"=FALSE}
  out "M 7":T5={"Boolean"=FALSE, "Boolean 2"=FALSE, "Boolean 3"=FALSE, "Boolean 4"=TRUE}
  out "Sonar 2":dbl(graph)=2.4353024850000002
  out "Right Drv Encoder 2":dbl=1456.4470125
  out "Left Drv Encoder 2":dbl=1461.0888475
  out "S 8":T5={"Boolean"=FALSE, "Boolean 2"=FALSE, "Boolean 3"=FALSE, "Boolean 4"=TRUE}
  out "G 8":T5={"Boolean"=TRUE, "Boolean 2"=FALSE, "Boolean 3"=FALSE, "Boolean 4"=FALSE}
  out "A 8":T5={"Boolean"=TRUE, "Boolean 2"=FALSE, "Boolean 3"=FALSE, "Boolean 4"=FALSE}
  out "M 8":T5={"Boolean"=FALSE, "Boolean 2"=FALSE, "Boolean 3"=FALSE, "Boolean 4"=TRUE}
  out "Yaw Turret 2":dbl=51.83726484818141
  out "Sonar Dist 2":dbl=2.4353024850000002
  in  "Sonar Gain 2":dbl=105.0
  in  "IMU Read Enable":T6={"Cal Status"=TRUE, "Orientation"=TRUE, "Gyro"=FALSE, "Accelerometer"=FALSE, "Quanterion"=FALSE, "Accel Mode"=enum."Linear", "Magnetometer"=FALSE, "Register Mode"=enum."Quaternion"}
  in  "Orient Ref (Wind)":T7 {"Pitch Ref" format="%#_13g"; "Roll Ref" format="%#_13g"; "Yaw Ref" format="%#_13g"}
  out "Good BU 2":bool=TRUE
  out "Home?":bool=TRUE
  out "Accel X":dbl(graph)
  in  "Width (sec)":dbl=0.01
  in  "y":dbl
  out "x .and. y?":bool
  in  "Tuning Mode?":bool
  in  "Load QCP":bool
  out "Out":bool
  in  "Gear Zero Down Power":dbl=-0.4
  in  "Gear Zero Down Time":dbl=1.0
  out "Encoder Pos":cluster{"setpoint":dbl, dbl}(graph)={"setpoint"=100.0, 88.32779009740001}
  in  "Intake Rev Spd":dbl(knob)=-1.0 scale=-1.0..1.0
  in  "Intake Fwd Spd":dbl(knob)=0.7095043451632626 scale=-1.0..1.0
  in  "PDP Addr":u8=1
  in  "PDP Channel":i32=9
  out "Tgrd 3":bool
  out "cnt 3":i16=40
  in  "Arm 2":bool
  in  "Trig 2":dbl=5.0
  in  "Len 2":i16=40
  in  "Reset1 2":bool
  out "Intake Motor Current":dbl(graph)
  out "State1 2":i32
  in  "reverse":bool
  in  "Thresh 1":dbl=20.0
  in  "Eval Period (sec)":dbl(knob)=0.19253649783681326 scale=0.0..1.0
  out "Stable":bool
  in  "output rate (EGU/min)":dbl(knob)=195.7494926389327 scale=0.0..500.0
  in  "reinitialize? (F)":bool
  out "Sensor Position":dbl=88.32779009740001
  in  "ZERO SENSOR":bool
  in  "Factor":dbl=310.0
  in  "Open":dbl(knob)=0.014738895236751093 scale=-1.0..1.0
  in  "Closed":bool=TRUE
  in  "Invert":bool
  in  "output range 2":cluster{"output high":dbl, "output low":dbl}={"output high"=0.45, "output low"=-0.25} {"output low" format="%.2f"; "output high" format="%.2f"}
  in  "PID gains":T4={"proportional gain (Kc)"=0.014, "integral time (Ti, min)"=0.0, "derivative time (Td, min)"=0.001} {"derivative time (Td, min)" format="%.6f"; "integral time (Ti, min)" format="%.3f"; "proportional gain (Kc)" format="%.6f"}
  in  "Catch":dbl(knob)=84.98128996789143 scale=0.0..100.0
  in  "Gear Overdone Thresh":dbl=99.0
  in  "Eval Period (sec) 2":dbl=0.1 format="%#_13g"
  in  "Absolute Encoder Factor":dbl=71.78
  in  "Absolute Encoder Shift":dbl=1.9555
  out "all currents (A)":dbl[](array[numeric])
  out "current (A)":dbl(graph)
  in  "PDP Channel 2":i32=2
  # ".01"
  # "0"
  # "i"
  # "p"
  # ".008\n.009"
  # "PID TUNING"
  # "Drive PID"
  # "Turn PID"
  # "0 Manual\n1 Turn\n2 Distance"
  # "P-Bot:\nP: 0.075?\nI: 0.001\nD: 5\nF: 0.0132"
  # "C-Bot:\nP: 0.04\nI: 0.0003\nD: 2\nF: 0.0132"
  # "P-Bot:\nP: 0.18\nI: 0.001\nD: 3\nF: 0.0288"
  # "C-Bot:\nP: 0.16\nI: 0.001\nD: 7\nF: 0.0288"
  # "NEEDS ACTUAL CONDITION"
  # "IMUs"
  # "Drive Encoders"
  # "Turret Encoders"
  # "Softstop BreakBeams"
  # "P-Bot"
  # "C-Bot (not finished)"
  # "Drive"
  # "Drive"
  # "0"
  # "Drive"
  # "Drive"
  # "2"
  # "Drive"
  # "Drive"
  # "Drive"
  # "Drive"
  # "---"
  # "4"
  # "---"
  # "---"
  # "---"
  # "6"
  # "Shooter (Bot)"
  # "---"
  # "---"
  # "Feeder"
  # "Gear Roller"
  # "8"
  # "---"
  # "Gear Roller"
  # "---"
  # "---"
  # "10"
  # "Climb"
  # "---"
  # "Turret"
  # "Shooter (Bot)"
  # "---"
  # "12"
  # "FMS"
  # "---"
  # "Shooter (Bot)"
  # "14"
  # "Shooter (Top)"
  # "Shooter (Bot)"
  # "Shooter (Top)"
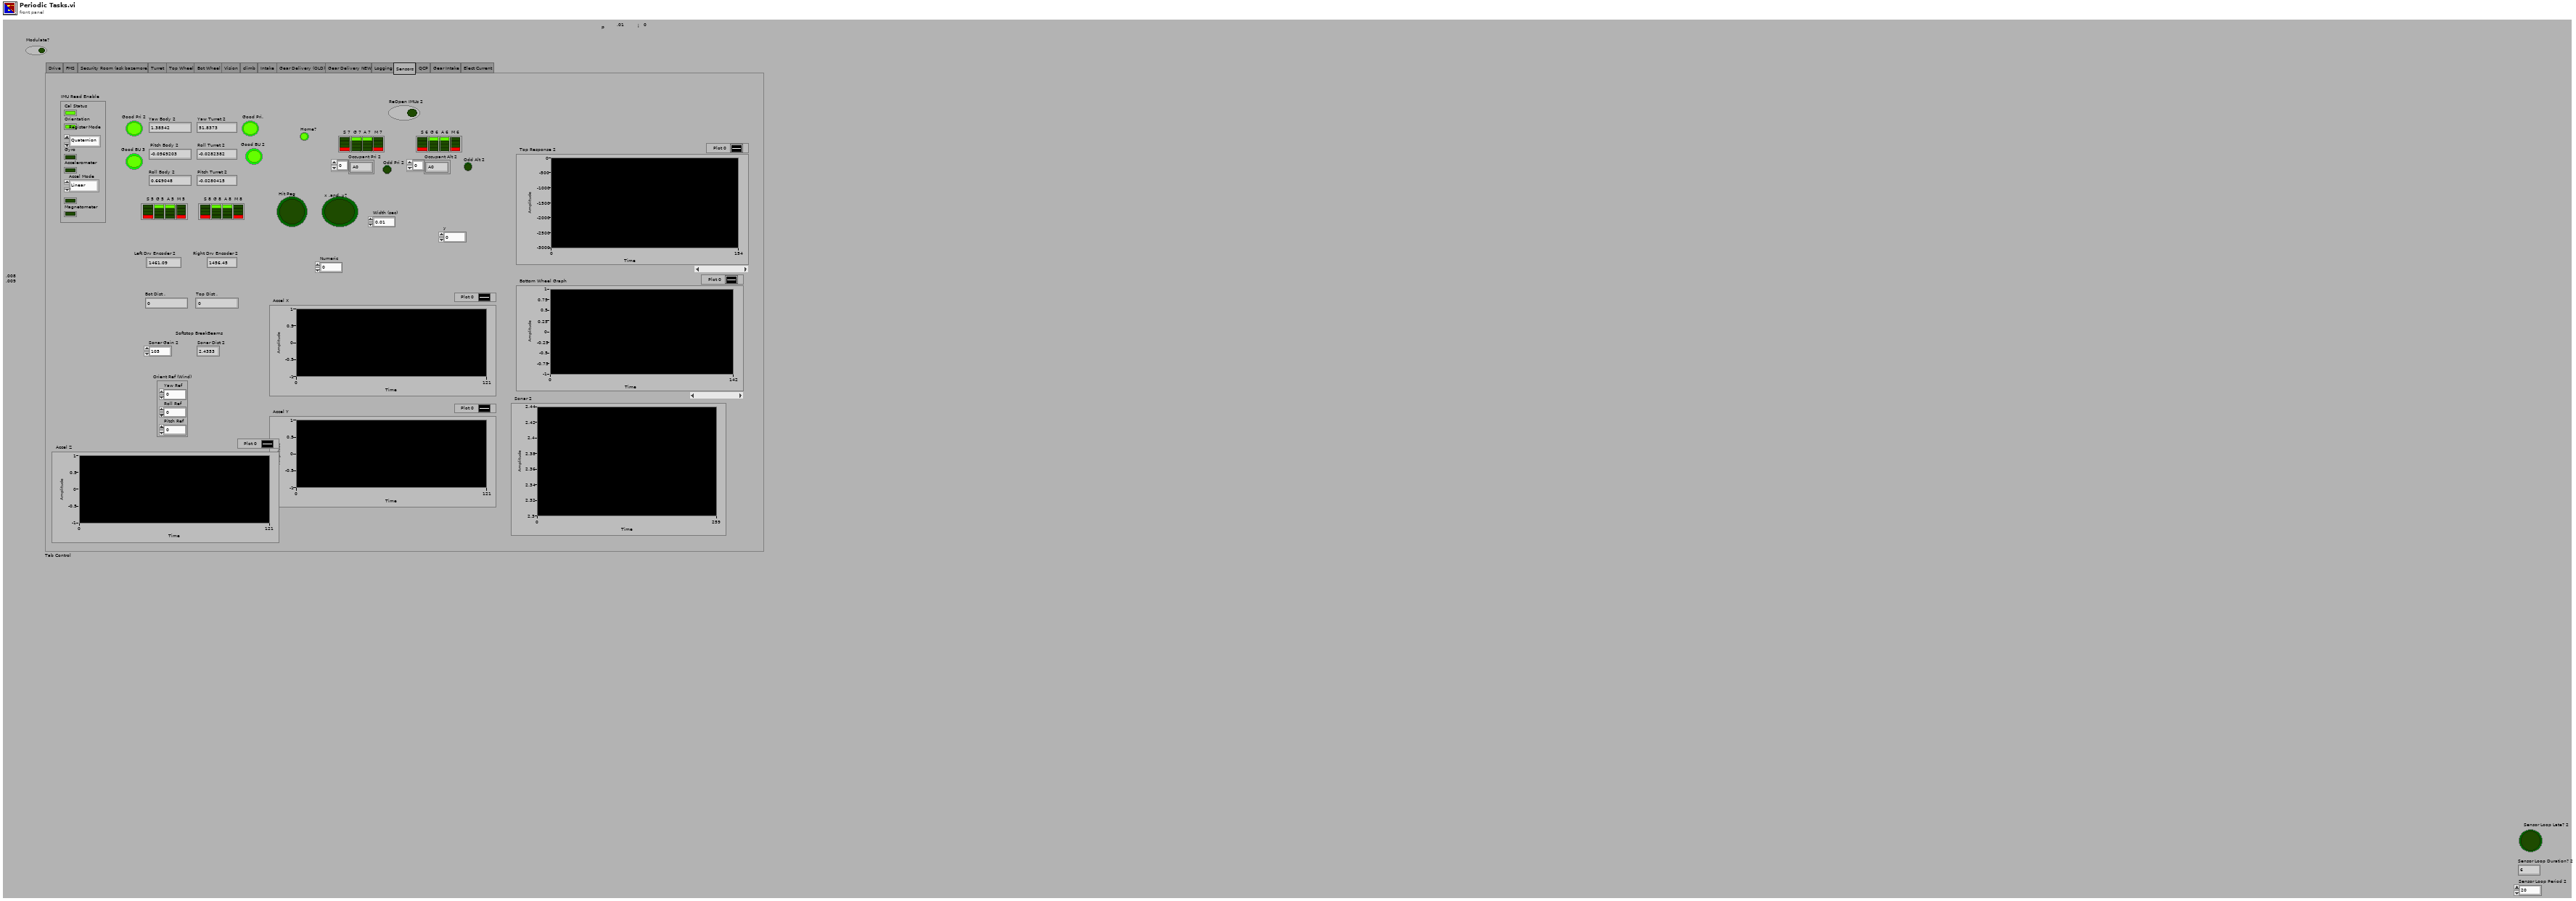
[diagram p1: front panel]
types:
  T1 = enum32{"Drive", "FMS", "Security Room (ask bazemore)", "Turret", "Top Wheel", "Bot Wheel", "Vision", "climb", "Intake", "Gear Delivery (OLD)", "Gear Delivery NEW", "Logging", "Sensors", "QCP", "Gear Intake", "Elect Current"}
  T2 = typedef "Drive_Code_PID_Bundle.ctl" = cluster{"Yaw, Driving Straight":cluster{"proportional gain (Kc)":dbl, "integral time (Ti, min)":dbl, "derivative time (Td, min)":dbl}, "Yaw, Holding Still":cluster{"proportional gain (Kc)":dbl, "integral time (Ti, min)":dbl, "derivative time (Td, min)":dbl}, "Distance, Driving Straight":cluster{"proportional gain (Kc)":dbl, "integral time (Ti, min)":dbl, "derivative time (Td, min)":dbl}, "Distance, Holding Still":cluster{"proportional gain (Kc)":dbl, "integral time (Ti, min)":dbl, "derivative time (Td, min)":dbl}}
  T3 = enum32{"Target Valid", "Search", "Guess/Desired Angle"}
  T4 = cluster{"proportional gain (Kc)":dbl, "integral time (Ti, min)":dbl, "derivative time (Td, min)":dbl}
  T5 = cluster{"Boolean":bool, "Boolean 2":bool, "Boolean 3":bool, "Boolean 4":bool}
  T6 = cluster{"Cal Status":bool, "Orientation":bool, "Gyro":bool, "Accelerometer":bool, "Quanterion":bool, "Accel Mode":enum8{"Raw Data", "Linear", "Gravity"}, "Magnetometer":bool, "Register Mode":enum8{"Euler", "Quaternion"}}
  T7 = cluster{"Yaw Ref":dbl, "Roll Ref":dbl, "Pitch Ref":dbl}
  T8 = typedef "WPI_CANTalonSRX_APIFeedbackSelect.ctl" = enum16{"Digital Quadrature Encoder", "Analog Potentiometer", "Analog Encoder", "Count on Quad-A (Rising-Edge)", "Count on Quad-A (Falling-Edge)", "CTR Magnetic Enc (Absolute)", "CTR Magnetic Enc (Relative)", "Pulse Width"}
  T9 = typedef "TurretImu.ctl" = enum16{"Pri Turret IMU", "Bu Turret IMU"}
  T10 = typedef "Control 1.ctl" = enum16{"Pri Body IMU", "Bu Body IMU"}
  T11 = typedef "TurretStates.ctl" = enum16{"Target Valid in Range", "Guess", "Search", "Desired Angle Shot", "Manual"}
  T12 = typedef "Gear Command.ctl" = enum16{"Home", "Floor Intake", "Catch", "Score"}
  T13 = typedef "FPGA_DIOChannel.ctl" = enum8{"DIO 0", "DIO 1", "DIO 2", "DIO 3", "DIO 4", "DIO 5", "DIO 6", "DIO 7", "DIO 8", "DIO 9", "DIO MXP 0", "DIO MXP 1", "DIO MXP 2", "DIO MXP 3", "DIO MXP 4", "DIO MXP 5", "DIO MXP 6", "DIO MXP 7", "DIO MXP 8", "DIO MXP 9", "DIO MXP 10", "DIO MXP 11", "DIO MXP 12", "DIO MXP 13", "DIO MXP 14", "DIO MXP 15", "SPI Port CS1", "SPI Port CS2", "SPI Port CS3", "SPI Port MISO", "SPI Port MOSI", "Invalid"}
  T14 = enum16{"open", "open or create", "create or replace", "create", "open (read-only)"}
  T15 = typedef "Shooting States.ctl" = enum16{"Wait", "Prepare for Shot", "Shoot", "Release"}
  T16 = typedef "Drive Commands.ctl" = enum16{"Manual", "Get Gear", "Score Gear", "Align Rope", "Turn To Angle", "Start Gear Score", "Place Gear", "Tank Drive", "Drive Distance"}
  T17 = typedef "Sensor_Cluster.ctl" = cluster{"Gyro Data":cluster{"Gyro RT FIFO":refnum<k33>, "Gyro Current":dbl, "Gyro Hold":dbl}, "Encoder Data":cluster{"Encoder RT FIFO":refnum<k33>, "Encoder Current":dbl, "Encoder Hold":dbl}, "Camera Data":cluster{"Camera RT FIFO":refnum<k33>, "Camera Current":T18}}
  T18 = typedef "Camera_Cluster.ctl" = cluster{" Angle":dbl, "Valid":bool}
  T19 = cluster{"Cluster":T17, "Drive Command rt fifo":refnum<k33>, "Logging Data":refnum<k33>, "PID Update":refnum<notifier>}
  T20 = typedef "WPI_RobotDriveDevRef.ctl" = cluster{"DevStatus":errorcluster, "Motors[]":T21[], "Square Inputs":bool, "Max Output":dbl}
  T21 = typedef "WPI_MotorControlDeviceRef.ctl" = cluster{"DeviceStatus":errorcluster, "Type":T22, "PWM":cluster{"PWM Channel":T23, "DeadBand":T24}, "CAN":cluster{"Device Number":u8, "SetOutput VI Ref":variant, "GetOutput VI Ref":variant, "Enable VI Ref":variant, "Disable VI Ref":variant, "Data":variant}, "Invert":bool}
  T22 = typedef "WPI_MotorControlType.ctl" = enum16{"PWM", "CAN"}
  T23 = typedef "FPGA_DIOPWMChannel.ctl" = enum8{"PWM 0", "PWM 1", "PWM 2", "PWM 3", "PWM 4", "PWM 5", "PWM 6", "PWM 7", "PWM 8", "PWM 9", "PWM MXP 0", "PWM MXP 1", "PWM MXP 2", "PWM MXP 3", "PWM MXP 4", "PWM MXP 5", "PWM MXP 6", "PWM MXP 7", "PWM MXP 8", "PWM MXP 9", "Invalid"}
  T24 = typedef "WPI_PWMDeadband.ctl" = cluster{"Name":string, "maxPositivePwm":i32, "minPositivePwm":i32, "centerPwm":i32, "maxNegativePwm":i32, "minNegativePwm":i32, "angularRange":u16}
  T25 = cluster{"Command":refnum<notifier>, "Status":refnum<queue>}
  T26 = typedef "Pneumatics_Position.ctl" = enum16{"Forward", "Reverse"}
  T27 = typedef "WPI_SolenoidDevRef.ctl" = cluster{"DevStatus":errorcluster, "Pneumatics Control Module":u8, "Forward Solenoid Channel":T28, "Reverse Solenoid Channel":T28}
  T28 = typedef "WPI_SolenoidChannel.ctl" = enum8{"Solenoid 0", "Solenoid 1", "Solenoid 2", "Solenoid 3", "Solenoid 4", "Solenoid 5", "Solenoid 6", "Solenoid 7", "Invalid"}
  T29 = cluster{"Control Notifier":refnum<notifier>, "Enum":T26, "SolenoidDevRef":T27, "Status Loop":refnum<k33>}
  T30 = typedef "XDNodeRunTimeDep.lvlib/timing_clust.ctl" = cluster{"Expected End [f-1]":u64, "Actual End [f-1]":u64, "Finished Late? [f-1]":bool, "Expected End [i-1]":u64, "Actual End [i-1]":u64, "Finished Late? [i-1]":bool, "Expected Start [i]":u64, "Actual Start [i]":u64, "Expected Start [f]":u64, "Actual Start [f]":u64, "Source Name":string, "Structure Name":string, "Period":i64, "Deadline":i64, "Offset":i64, "Start":i64, "Priority":i32, "Timeout":i32, "Mode":T31, "Wakeup Reason":T32, "Error":errorcluster, "Source Type":string, "Secondary Source Type":string, "Global End Time":u64, "Global Start Time":u64, "Frame Duration":u64, "Iteration Duration":u64, "Assigned CPU":i32, "I/O Scan Engine Mode":u32}
  T31 = typedef "XDNodeRunTimeDep.lvlib/nitl_modes.ctl" = enum32{"No Change", "Process missed periods, maintain original phase", "Discard missed periods, maintain original phase", "Process missed periods, ignore original phase", "Discard missed periods, ignore original phase"}
  T32 = typedef "XDNodeRunTimeDep.lvlib/wakeup.ctl" = enum32{"Normal", "Aborted", "Asynchronous wakeup", "Timing source error", "Timed loop error", "Timeout"}
  T33 = typedef "WPI_I2CDevRef.ctl" = cluster{"DevStatus":errorcluster, "Device Address":u8, "Handle":i32, "I2C Bus":T34}
  T34 = typedef "i2c_bus.ctl" = enum16{"I2C On-Board", "I2C MXP", "Invalid"}
  T35 = typedef "Pneumatics_Command.ctl" = enum16{"Nothing", "Forward", "Reverse", "Toggle"}
  T36 = typedef "FMS Commands.ctl" = enum16{"Shoot", "Un-Jam", "Stop"}
  T37 = typedef "WPI_DriverStationAllianceInfo.ctl" = enum16{"Red", "Blue", "Invalid"}
  T38 = typedef "MatchTimeNotifications.ctl" = enum16{"oneMinuteLeft", "thirtySecondsLeft", "tenSecondsLeft", "matchOver"}
  T39 = typedef "WPI_DriverStationRobotMode2.ctl" = enum16{"Autonomous Disabled", "Autonomous Enabled", "Teleop Disabled", "Teleop Enabled", "Disconnected", "Finish", "Test Disabled", "Test Enabled", "Emergency Stopped"}
  T40 = enum8{"setop", "setcolor", "default", "pilot", "ball", "gear", "both", "gearDeliver", "timeWarn", "targeting", "rave", "debug", "Set Power"}
  T41 = typedef "WPI_CANTalonSRX_APIControlMode.ctl" = enum8{"Percent VBus", "Speed", "Position", "Slave", "Unchanged / Invalid", "Voltage Compensation", "Current", "Motion Profile", "Motion Magic"}
  T42 = typedef "WPI_CANTalonSRX_GlobalStatus.ctl" = cluster{"Applied Throttle":dbl, "Module Enabled":bool, "CAN Error":errorcluster, "Closed Loop Error":dbl, "Forward Limit Switch Closed":bool, "Reverse Limit Switch Closed":bool, "Sensor Position":dbl, "Sensor Velocity":dbl, "Current":dbl, "Sticky Fault - Over Temp":bool, "Sticky Fault - Under Voltage":bool, "Sticky Fault - Forward Limit":bool, "Sticky Fault - Reverse Limit":bool, "Sticky Fault - Forward Soft Limit":bool, "Sticky Fault - Reverse Soft Limit":bool, "Brake is Enabled":bool, "Encoder Position":dbl, "Encoder Velocity":dbl, "Encoder Index Count":dbl, "Encoder A Pin State":bool, "Encoder B Pin State":bool, "Encoder Index Pin State":bool, "Analog In":dbl, "Analog In Velocity":dbl, "Temperature (C)":dbl, "Battery Voltage":dbl, "Control 5 Is Supported":bool, "Current Profile Slot Select":dbl, "Pos Div 8":bool, "Vel Div 4":bool, "Pulse Width Position":i32, "Pulse Width Velocity":i32, "Pulse Width Rise To Rise (us)":i32, "Pulse Width Rise To Fall (us)":i32, "Mot Prof Active Is Under Run":bool, "Mot Prof Active Has Under Run":bool, "Mot Prof Active Is Last":bool, "Mot Prof Active Velocity Only":bool, "Mot Prof Active Is Valid":bool, "Mot Prof Buffer Is Full":bool, "Mot Prof Active Profile Slot Select":i32, "Mot Prof NextID":i32, "Mot Prof Count":i32, "Mot Prof Active Velocity":dbl, "Mot Prof Active Position":dbl, "Mot Prof Output Enable":i32}
  T43 = typedef "FPGA_AIChannel.ctl" = enum8{"AI 0", "AI 1", "AI 2", "AI 3", "AI MXP 0", "AI MXP 1", "AI MXP 2", "AI MXP 3", "Invalid"}
  T44 = typedef "WPI_AnalogChannelDevRef.ctl" = cluster{"DevStatus":errorcluster, "Analog Channel":T43}
  T45 = typedef "WPI_DigitalInputDevRef.ctl" = cluster{"DevStatus":errorcluster, "DIO Channel":T13}
  T46 = typedef "Control 1" = enum16{"Home", "Floor Intake", "Catch", "Score"}
  T47 = cluster{"Search Gains":cluster{"proportional gain (Kc)":dbl, "integral time (Ti, min)":dbl, "derivative time (Td, min)":dbl}, "Search Range":cluster{"output high":dbl, "output low":dbl}}
  T48 = cluster{"Jump to Desired Angle":cluster{"proportional gain (Kc)":dbl, "integral time (Ti, min)":dbl, "derivative time (Td, min)":dbl}, "Jump Output":cluster{"output high":dbl, "output low":dbl}}
  T49 = cluster{"Target Range Gains":cluster{"proportional gain (Kc)":dbl, "integral time (Ti, min)":dbl, "derivative time (Td, min)":dbl}, "Target range":cluster{"output high":dbl, "output low":dbl}}
  T50 = cluster{"Target Range Gains":cluster{"proportional gain (Kc)":dbl, "integral time (Ti, min)":dbl, "derivative time (Td, min)":dbl}, "Target range":cluster{"output high":dbl, "output low":dbl}}[]
  T51 = typedef "NI_AAL_Angle.lvlib/Angle Range (Degree).ctl" = u16
  T52 = typedef "NI_AAL_Angle.lvlib/Angle Units.ctl" = i32
  T53 = typedef "WPI_EncoderDevRef.ctl" = cluster{"DevStatus":errorcluster, "EncoderIndex":T54, "CounterIndex":T55, "DistancePerCount":dbl, "Decoding Type":T56}
  T54 = typedef "FPGA_EncoderIdx.ctl" = enum8{"Enc 0", "Enc 1", "Enc 2", "Enc 3", "Enc 4", "Enc 5", "Enc 6", "Enc 7", "Invalid"}
  T55 = typedef "FPGA_CounterCtrSystemIndex.ctl" = enum8{"Ctr 0", "Ctr 1", "Ctr 2", "Ctr 3", "Ctr 4", "Ctr 5", "Ctr 6", "Ctr 7", "Invalid"}
  T56 = typedef "WPI_EncoderType.ctl" = enum16{"1x", "2x", "4x"}
  T57 = enum8{"ConfigMode", "AccOnly", "MagOnly", "GyroOnly", "AccMag", "AccGyro", "MagGyro", "AMG", "IMU", "Compass", "M4G", "NDOF_FMC_OFF", "NDOF"}
  T58 = cluster{"Mag":cluster{"[0]":bool, "[1]":bool, "[2]":bool, "[3]":bool}, "Acc":cluster{"[0]":bool, "[1]":bool, "[2]":bool, "[3]":bool}, "Gyro":cluster{"[0]":bool, "[1]":bool, "[2]":bool, "[3]":bool}, "Sys":cluster{"[0]":bool, "[1]":bool, "[2]":bool, "[3]":bool}, "Status":bool}
  T59 = cluster{"Yaw":dbl, "Roll":dbl, "Pitch":dbl, "Yaw Wind":dbl, "Roll Wind":dbl, "Pitch Wind":dbl}
  T60 = cluster{"[0]":bool, "[1]":bool, "[2]":bool, "[3]":bool}
  T61 = cluster{"Cluster":cluster{"[0]":bool, "[1]":bool, "[2]":bool, "[3]":bool}, "Cluster":cluster{"[0]":bool, "[1]":bool, "[2]":bool, "[3]":bool}, "Cluster":cluster{"[0]":bool, "[1]":bool, "[2]":bool, "[3]":bool}, "Cluster":cluster{"[0]":bool, "[1]":bool, "[2]":bool, "[3]":bool}}
  T62 = enum16{"Autonomous Disabled", "Autonomous Enabled", "Teleop Disabled", "Teleop Enabled", "Disconnected", "Finish", "Test Disabled", "Test Enabled", "Emergency Stopped"}
  T63 = enum16{"Calculate Path", "Drive Path", "Gear Cam Placement"}
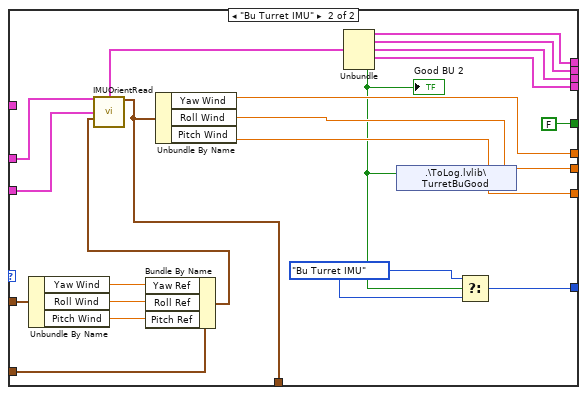
[diagram p5: hidden frame]
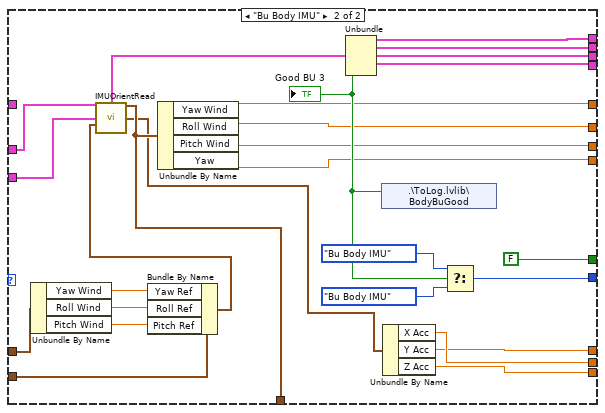
[diagram p6: hidden frame]
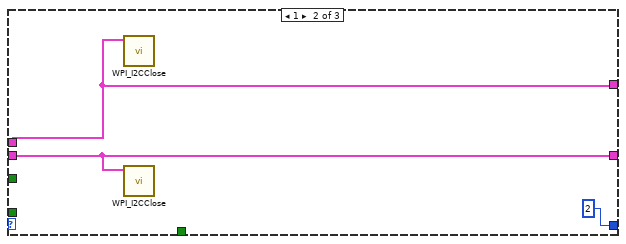
[diagram p7: hidden frame]
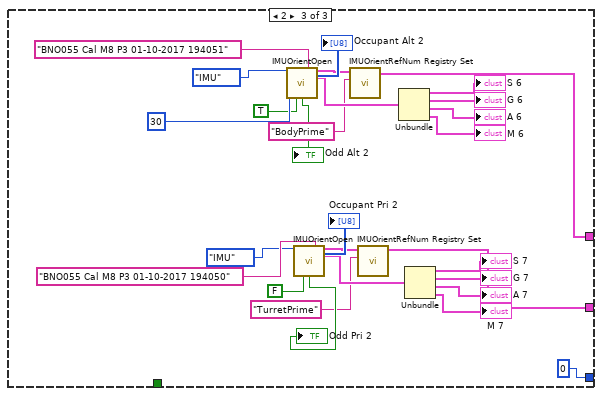
[diagram p8: hidden frame]
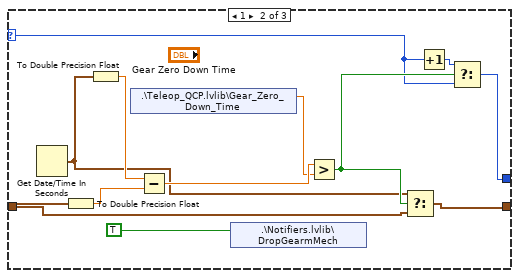
[diagram p13: hidden frame]
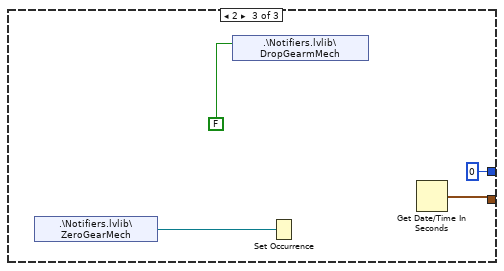
[diagram p14: hidden frame]
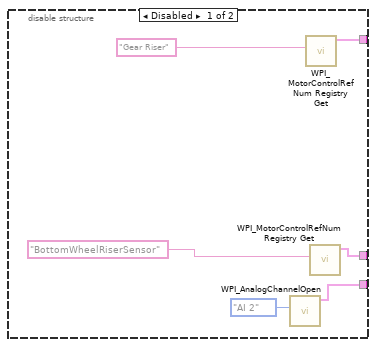
[diagram p15: hidden frame]
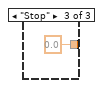
[diagram p17: hidden frame]
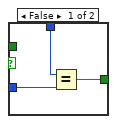
[diagram p20: hidden frame]
diagram:
  w80 = 29 ("dimension size")
  (unwired) TRUE ("Invert Throttle")
  (unwired) FALSE ("Invert Steer")
  # "RelTime\nRobotMode\nRIO Voltage\nBodyPriGood\nBodyBuGood\nTurretPriGood\nTurretBuGood\nFireButton\nShooterBotBumps\nShooterTopBumps\nTurret Bumps\nBoilerCamDist\nBoilerBearing\nBoilerValid\nGearCamDist\nGearBearing\nGearValid\nAutoState\nbody imu yaw\nturret imu yaw\nleft encoder\nright encoder\ntop shooter ctrl\ntop shooter repsonse\nbot shooter ctrl\nbot shooter response\nburst"
  # "arch length points\ntheta points\nleft encoder\nright encoder\nBody IMU Yaw Ref\nTurn Gear Setpoint"
  # "Drive FIFO Setup"
  # "Size of Drive Log"
  n1 = shared-variable ".\\ControlMode.lvlib\\Manual Mode?"() -> ()  [unwired: 1 in, 2 out]
  n2 = call <vilib>:"WPI_DriverStationStart Communication.vi"() -> ()  [unwired: 12 in]
  n3 = shared-variable ".\\Notifiers.lvlib\\Drive Command Notifier"() -> (w98:refnum<notifier>)  [unwired: 1 in, 1 out]
  n4 = shared-variable ".\\Notifiers.lvlib\\Drive Loop Cluster"() -> (w99:T19)  [unwired: 1 in, 1 out]
  n5 = call <vilib>:"WPI_RobotDriveRefNum Registry Get.vi"("refnum name"="Drive Motors") -> ("RobotDriveDevRef"=w113:T20)  [unwired: 9 in, 1 out]
  n6 = shared-variable ".\\Notifiers.lvlib\\GearShift Command DevRef"() -> (w94:T25)  [unwired: 1 in, 1 out]
  n7 = shared-variable ".\\Notifiers.lvlib\\Gear Shift Control Loop"() -> (w93:T29)  [unwired: 1 in, 1 out]
  n8 = call <userlib>:"Drive_Loop_Control_Loop.vi"("Period \n- Amount of time between iterations of the timed control loop"=i64 20 ("Period \n- Amount of time between iterations of the timed control loop"), "RobotDriveDevRef"=w113, "Control Cluster"=w99) -> ()  [unwired: 9 in]
  n9 = shared-variable ".\\Notifiers.lvlib\\FMS Command Notifier"() -> (w86:refnum<notifier>)  [unwired: 1 in, 1 out]
  n10 = shared-variable ".\\Notifiers.lvlib\\Intake Notifier"() -> (w87:refnum<notifier>)  [unwired: 1 in, 1 out]
  n11 = call <userlib>:"Pneumatic_Control_Loop.vi"("Cluster in"=w93) -> ()  [unwired: 11 in]
  n12 = disable-structure shown="Disabled" {
    frame Disabled {
      n13 = shared-variable ".\\Notifiers.lvlib\\NeoPixel Controls"() -> (w122:refnum<notifier>)  [unwired: 1 in, 1 out]
      n14 = call <vilib>:"WPI_I2CRefNum Registry Get.vi"("refnum name"="i2c") -> ("I2CDevRef"=w123:T33)  [unwired: 9 in, 1 out]
      n15 = node-c288() -> (w126:T30)  [unwired: 4 in]
      n16 = timed-loop {
        tunnel: w122 -> [w145]
        timing: w126 -> [_]
        timing-out: [_] -> w125
        tunnel: w123 -> [w143]
        shift-right: [w139] -> _
        shift-left: _ -> [w142]
        stop <- FALSE stop-if-true
        # "COMMAND TIMEMODE"
        # "NeoPixel Control Loop"
        n17 = node-c288() -> (→"NeoPixel Loop Late?":bool, →"NeoPixel Loop Duration":i64)  [unwired: 1 in]
        n18 = Select(t=-1, s="NeoPixel Blocking?", f=0 ("index")) -> (s? t:f=w129:i32)
        n19 = Wait on Notification(notifier=w145, timeout in ms (-1)=w129) -> (notification=w139:u8[], timed out?=w144:bool)  [unwired: 2 in, 2 out]
        n20 = Index Array(array=w139, index=0) -> (element=w137:u8)
        n21 = Equal?(x=w137, y=u8 0) -> (x = y?=w135:bool)
        n22 = feedback #1() -> (w140:u8[])  [unwired: 1 in]
        n23 = Select(t=w140, s=w135, f=w142) -> (s? t:f=w141:u8[])
        n24 = feedback-in #1(w141) -> ()
        n25 = case shown="False" w144 {
          tunnel: w139 -> [w149 _]
          tunnel: w143 -> [w151 _]
          frame False {
            n26 = call <vilib>:"WPI_I2CWrite.vi"("I2CDataToSend"=w149, "I2CRegister"=u8 8, "I2CDevRef"=w151) -> ()  [unwired: 7 in, 2 out]
          }
          frame True {
          }
        }
        n27 = node-c288("NeoPixel Period") -> ()  [unwired: 1 out]
      }
      n28 = node-c288(w125) -> ()  [unwired: 1 out]
    }
    frame Enabled {
    }
  }
  n29 = call <vilib>:"WPI_MotorControlRefNum Registry Get.vi"("refnum name"="BottomWheel") -> ("MotorControlDevRef"=w121:T21)  [unwired: 9 in, 1 out]
  n30 = shared-variable ".\\Notifiers.lvlib\\FMS Command Notifier"() -> (w96:refnum<notifier>)  [unwired: 1 in, 1 out]
  n31 = shared-variable ".\\Notifiers.lvlib\\NeoPixel Controls"() -> (w49:refnum<notifier>)  [unwired: 1 in, 1 out]
  n32 = node-c288() -> (w115:T30)  [unwired: 4 in]
  n33 = shared-variable ".\\OperatorController.lvlib\\Clear Bumps"() -> (w41:refnum<k4>)  [unwired: 1 in, 1 out]
  n34 = call <vilib>:"WPI_MotorControlRefNum Registry Get.vi"("refnum name"="TopWheel") -> ("MotorControlDevRef"=w44:T21)  [unwired: 9 in, 1 out]
  n35 = node-c288() -> (w90:T30)  [unwired: 4 in]
  n36 = call <vilib>:"WPI_MotorControlRefNum Registry Get.vi"("refnum name"="FMS") -> ("MotorControlDevRef"=w111:T21)  [unwired: 9 in, 1 out]
  n37 = call <vilib>:"WPI_MotorControlRefNum Registry Get.vi"("refnum name"="Feeder") -> ("MotorControlDevRef"=w110:T21)  [unwired: 9 in, 1 out]
  n38 = call <vilib>:"WPI_MotorControlRefNum Registry Get.vi"("refnum name"="Roller") -> ("MotorControlDevRef"=w5:T21)  [unwired: 9 in, 1 out]
  n39 = shared-variable ".\\Vision Variables.lvlib\\TargetTracking"(TRUE ("TargetTracking")) -> ()  [unwired: 1 in, 1 out]
  n40 = timed-loop {
    timing: w115 -> [_]
    timing-out: [_] -> w114
    tunnel: w94 -> [w163]
    stop <- FALSE stop-if-true
    # "GearShift Loop"
    n41 = node-c288() -> (→"Gear Shift Loop Late?":bool, →"Gear Shift Loop Duration":i64)  [unwired: 1 in]
    n42 = shared-variable ".\\Sensors.lvlib\\High Gear?"() -> (w160:bool)  [unwired: 1 in, 1 out]
    n43 = feedback-in #2(w160) -> ()
    n44 = feedback #2() -> (w159:bool)  [unwired: 1 in]
    n45 = Not Equal?(x=w160, y=w159) -> (x != y?=w162:bool)
    n46 = case shown="True" w162 {
      tunnel: w163 -> [_ w172]
      tunnel: w160 -> [_ w171]
      frame False {
      }
      frame True {
        n47 = Select(t=Pneumatics_Command."Forward" ("Solenoid Command"), s=w171, f=Pneumatics_Command."Reverse" ("Solenoid Command")) -> (s? t:f=w168:T35)
        n48 = call-poly <userlib>:"Pneumatics_Command_Set.vi"("Solenoid Command"=w168, "Cluster"=w172) -> ()  [unwired: 9 in, 1 out]
      }
    }
    n49 = node-c288("Gear Shift Period") -> ()  [unwired: 1 out]
  }
  n50 = node-c288() -> (w117:T30)  [unwired: 4 in]
  n51 = timed-loop {
    timing: w90 -> [_]
    timing-out: [_] -> w89
    shift-right: [w181] -> _
    shift-left: Shooting_States."Wait" -> [w188]
    tunnel: w87 -> [w187]
    tunnel: w86 -> [w186]
    stop <- _ stop-if-true
    # "Shooter State Machine"
    n52 = node-c288() -> (→"Shooter SM Duration":i64, →"Shooter SM Late?":bool)  [unwired: 1 in]
    n53 = case shown="\"Prepare for Shot\"" w188 {
      selector: w188 -> [w191 w196 w201 _]
      tunnel: [w190 w200 w201 Shooting_States."Wait"] -> w182
      tunnel: w187 -> [_ _ w205 w208]
      tunnel: w186 -> [_ _ w204 w207]
      frame "Wait", Default {
        n54 = shared-variable ".\\ControlMode.lvlib\\ShootingMode"() -> (w192:bool)  [unwired: 1 in, 1 out]
        n55 = Select(t=Shooting_States."Prepare for Shot", s=w192, f=w191) -> (s? t:f=w190:T15)
      }
      frame "Prepare for Shot" {
        n56 = shared-variable ".\\Auto Variables.lvlib\\OverrideSpinUpTime"() -> (w193:bool)  [unwired: 1 in, 1 out]
        n57 = shared-variable ".\\Sensors.lvlib\\Bottom Wheel Steady"() -> (w197:bool)  [unwired: 1 in, 1 out]
        n58 = shared-variable ".\\Sensors.lvlib\\Top Wheel Steady"() -> (w198:bool)  [unwired: 1 in, 1 out]
        n59 = Compound Arithmetic op=AND(w198, w197) -> (w195:bool)
        n60 = Or(x=w195, y=w193) -> (x .or. y?=w194:bool)
        n61 = Select(t=Shooting_States."Shoot", s=w194, f=w196) -> (s? t:f=w200:T15)
      }
      frame "Shoot" {
        n62 = Send Notification(notification=FMS_Commands."Shoot", notifier=w204) -> ()  [unwired: 1 in, 2 out]
        n63 = Send Notification(notification=FMS_Commands."Shoot", notifier=w205) -> ()  [unwired: 1 in, 2 out]
      }
      frame "Release" {
        n64 = Send Notification(notification=FMS_Commands."Stop", notifier=w208) -> ()  [unwired: 1 in, 2 out]
        n65 = Send Notification(notification=FMS_Commands."Stop", notifier=w207) -> ()  [unwired: 1 in, 2 out]
      }
    }
    n66 = shared-variable ".\\ControlMode.lvlib\\ShootingMode"() -> (w185:bool)  [unwired: 1 in, 1 out]
    n67 = feedback-in #3(w185) -> ()
    n68 = feedback #3(FALSE ("Boolean")) -> (w184:bool)
    n69 = Less?(x=w185, y=w184) -> (x < y?=w183:bool)
    n70 = Select(t=Shooting_States."Release", s=w183, f=w182) -> (s? t:f=w181:T15)
    n71 = node-c288("Shooter SM Period") -> ()  [unwired: 1 out]
  }
  n72 = shared-variable ".\\OperatorController.lvlib\\Clear Bumps"() -> (w42:refnum<k4>)  [unwired: 1 in, 1 out]
  n73 = node-c288() -> (w119:T30)  [unwired: 4 in]
  n74 = shared-variable ".\\Notifiers.lvlib\\Home!"() -> (w34:refnum<k4>)  [unwired: 1 in, 1 out]
  n75 = disable-structure shown="Disabled" {
    frame Disabled {
      n76 = shared-variable ".\\Notifiers.lvlib\\Intake Notifier"() -> (w218:refnum<notifier>)  [unwired: 1 in, 1 out]
      n77 = call <vilib>:"WPI_MotorControlRefNum Registry Get.vi"("refnum name"="Intake") -> ("MotorControlDevRef"=w219:T21)  [unwired: 9 in, 1 out]
      n78 = node-c288() -> (w221:T30)  [unwired: 4 in]
      n79 = timed-loop {
        timing: w221 -> [_]
        timing-out: [_] -> w220
        tunnel: w218 -> [w229]
        tunnel: w219 -> [w222]
        stop <- _ stop-if-true
        # "Intake Control Loop"
        n80 = node-c288() -> (→"Intake Control Late?":bool, →"Intake Control Duration":i64)  [unwired: 1 in]
        n81 = Select(t=-1, s="Intake Blocking?", f=0) -> (s? t:f=w225:i32)
        n82 = Wait on Notification(notifier=w229, timeout in ms (-1)=w225) -> (notification=w223:T36, timed out?=w224:bool)  [unwired: 2 in, 2 out]
        n83 = case shown="False" w224 {
          tunnel: w223 -> [w236 _]
          tunnel: w222 -> [w235 _]
          frame False {
            n84 = case shown="\"Un-Jam\"" w236 {
              tunnel: "Intake speed" -> [w237 w238 _]
              tunnel: [w237 w239 0.0 ("Intake speed")] -> w233
              frame "Shoot", Default {
              }
              frame "Un-Jam" {
                n85 = Negate(x=w238) -> (-x=w239:dbl)
              }
              frame "Stop" {
              }
            }
            n86 = call <vilib>:"WPI_MotorControlSetOutput.vi"("Output"=w233, "MotorControlDevRef"=w235) -> ()  [unwired: 7 in, 3 out]
          }
          frame True {
          }
        }
        n87 = node-c288("Intake Period") -> ()  [unwired: 1 out]
      }
      n88 = node-c288(w220) -> ()  [unwired: 1 out]
    }
    frame Enabled {
    }
  }
  n89 = timed-loop {
    timing: w117 -> [_]
    timing-out: [_] -> w116
    tunnel: w96 -> [w266]
    tunnel: w111 -> [w257]
    tunnel: w110 -> [w256]
    shift-right: [w254] -> _
    shift-left: _ -> [w255]
    tunnel: w5 -> [w250]
    stop <- FALSE stop-if-true
    # "FMS Control Loop"
    n90 = node-c288() -> (→"FMS Control Late?":bool, →"FMS Control Duration":i64)  [unwired: 1 in]
    n91 = shared-variable ".\\ControlMode.lvlib\\Tuning Mode?"() -> (w249:bool)  [unwired: 1 in, 1 out]
    n92 = Select(t=-1, s="FMS Blocking?", f=0) -> (s? t:f=w263:i32)
    n93 = Wait on Notification(notifier=w266, timeout in ms (-1)=w263) -> (notification=w260:T36, timed out?=w261:bool)  [unwired: 2 in, 2 out]
    n94 = feedback #4(FMS_Commands."Stop" ("Enum")) -> (w252:T36)
    n95 = case shown="True" w261 {
      tunnel: w260 -> [w272 _]
      tunnel: w257 -> [_ w298]
      tunnel: w256 -> [_ w299]
      tunnel: [w273 w291] -> w254
      tunnel: w255 -> [w273 _]
      tunnel: [w272 w296] -> w253
      tunnel: w252 -> [_ w296]
      tunnel: w250 -> [_ w293]
      tunnel: w249 -> [_ w276]
      frame False {
      }
      frame True {
        n96 = shared-variable ".\\Teleop_QCP.lvlib\\Feeder_Speed"() -> (w285:dbl)  [unwired: 1 in, 1 out]
        n97 = shared-variable ".\\Teleop_QCP.lvlib\\FMS_Transition_Fwd_Speed"() -> (w277:dbl)  [unwired: 1 in, 1 out]
        n98 = shared-variable ".\\Teleop_QCP.lvlib\\FMS_Forward_Speed"() -> (w279:dbl)  [unwired: 1 in, 1 out]
        n99 = feedback-in #5(w296) -> ()
        n100 = feedback #5() -> (w297:T36)  [unwired: 1 in]
        n101 = shared-variable ".\\Teleop_QCP.lvlib\\FMS_Duty_Cycle"() -> (w282:dbl)  [unwired: 1 in, 1 out]
        n102 = shared-variable ".\\Teleop_QCP.lvlib\\FMS_Period"() -> (w278:dbl)  [unwired: 1 in, 1 out]
        n103 = Select(t="Feeder Speed", s=w276, f=w285) -> (s? t:f=w283:dbl)
        n104 = Select(t="FMS Speed", s=w276, f=w279) -> (s? t:f=w281:dbl)
        n105 = Select(t="Trans Roller", s=w276, f=w277) -> (s? t:f=w274:dbl)
        n106 = case shown="\"Shoot\", Default" w296 {
          selector: w296 -> [w339 _ _]
          tunnel: [w323 w343 w345] -> w295
          tunnel: [w330 w342 w345] -> w294
          tunnel: w297 -> [w328 _ _]
          tunnel: w283 -> [w327 _ _]
          tunnel: w281 -> [w324 w344 _]
          tunnel: w274 -> [w319 _ _]
          tunnel: [w320 w342 w345] -> w290
          tunnel: w276 -> [w300 _ _]
          tunnel: w282 -> [w316 _ _]
          tunnel: w278 -> [w313 _ _]
          frame "Shoot", Default {
            n107 = Not Equal?(x=w339, y=w328) -> (x != y?=w340:bool)
            n108 = shared-variable ".\\Teleop_QCP.lvlib\\FMS_Transition_Duty_Cycle"() -> (w309:dbl)  [unwired: 1 in, 1 out]
            n109 = call <userlib>:"Signal_Pulse.vi"("Input"=w340) -> ("Output"=w341:bool)
            n110 = shared-variable ".\\Teleop_QCP.lvlib\\FMS_Transition_Period"() -> (w306:dbl)  [unwired: 1 in, 1 out]
            n111 = shared-variable ".\\Teleop_QCP.lvlib\\FMS_Transition_Rev_Speed"() -> (w303:dbl)  [unwired: 1 in, 1 out]
            n112 = Not(x=w341) -> (.not. x?=w338:bool)
            n113 = Select(t="FMS Duty Cycle", s=w300, f=w316) -> (s? t:f=w318:dbl)
            n114 = Select(t="FMS Period", s=w300, f=w313) -> (s? t:f=w315:dbl)
            n115 = shared-variable ".\\Teleop_QCP.lvlib\\FMS_Reverse_Speed"() -> (w310:dbl)  [unwired: 1 in, 1 out]
            n116 = call "Square Waves Generator.vi"("Duty Cycle (%)"=w318, "Period (ms)"=w315, "Enable"=TRUE) -> ("Signal"=w333:bool)
            n117 = call "Square Waves Generator.vi"("Duty Cycle (%)"="Feeder Duty Cycle", "Period (ms)"="Feeder Period", "Enable"=w338) -> ("Signal"=w335:bool)
            n118 = Select(t="Transition Roller Duty Cycle", s=w300, f=w309) -> (s? t:f=w307:dbl)
            n119 = Not(x=w335) -> (.not. x?=w336:bool)
            n120 = Select(t="TR Period", s=w300, f=w306) -> (s? t:f=w304:dbl)
            n121 = Select(t="Trans Roller Reverse Speed", s=w300, f=w303) -> (s? t:f=w301:dbl)
            n122 = Select(t=w336, s="Offset?", f=w335) -> (s? t:f=w334:bool)
            n123 = call "Square Waves Generator.vi"("Duty Cycle (%)"=w307, "Period (ms)"=w304, "Enable"=TRUE) -> ("Signal"=w321:bool)
            n124 = Select(t="FMS Reverse Speed", s=w300, f=w310) -> (s? t:f=w312:dbl)
            n125 = Select(t=w324, s=w333, f=w312) -> (s? t:f=w325:dbl)
            n126 = Select(t=w327, s=w334, f=w327) -> (s? t:f=w330:dbl)
            n127 = Select(t=w325, s="Modulate?", f=w324) -> (s? t:f=w323:dbl)
            n128 = Select(t=w319, s=w321, f=w301) -> (s? t:f=w320:dbl)
          }
          frame "Un-Jam" {
            w342 = 0.0 ("f")
            n129 = Negate(x=w344) -> (-x=w343:dbl)
          }
          frame "Stop" {
            w345 = 0.0
          }
        }
        n130 = shared-variable ".\\ControlMode.lvlib\\Tuning Mode?"() -> (w287:bool)  [unwired: 1 in, 1 out]
        n131 = shared-variable ".\\Teleop_QCP.lvlib\\FMS_Rate_Limit"() -> (w286:dbl)  [unwired: 1 in, 1 out]
        n132 = Select(t="rate", s=w287, f=w286) -> (s? t:f=w289:dbl)
        n133 = call-poly <vilib>:"PID Output Rate Limiter.vi"("output rate (EGU/min)"=w289, "initial output"=w295, "input (controller output)"=w295) -> ("output"=w291:dbl)  [unwired: 5 in, 1 out]
        n134 = Negate(x=w290) -> (-x=w292:dbl)
        n135 = call <vilib>:"WPI_MotorControlSetOutput.vi"("Output"=w291, "MotorControlDevRef"=w298) -> ()  [unwired: 7 in, 3 out]
        n136 = call <vilib>:"WPI_MotorControlSetOutput.vi"("Output"=w294, "MotorControlDevRef"=w299) -> ()  [unwired: 7 in, 3 out]
        n137 = call <vilib>:"WPI_MotorControlSetOutput.vi"("Output"=w292, "MotorControlDevRef"=w293) -> ()  [unwired: 7 in, 3 out]
      }
    }
    "Motor Out" <- w254
    n138 = feedback-in #4(w253) -> ()
    n139 = node-c288("FMS Period") -> ()  [unwired: 1 out]
  }
  n140 = timed-loop {
    timing: w119 -> [_]
    timing-out: [_] -> w118
    tunnel: w99 -> [w367]
    tunnel: w98 -> [w349]
    border: Drive_Commands."Manual" ("notification") -> [_]
    shift-right: [w359] -> _
    shift-left: _ -> [w357]
    shift-right: [w360] -> _
    shift-left: _ -> [w358]
    shift-right: [w356] -> _
    shift-left: _ -> [w354]
    shift-right: [w355] -> _
    shift-left: _ -> [w353]
    shift-right: [w352] -> _
    shift-left: _ -> [w351]
    stop <- FALSE stop-if-true
    # "4811922"
    # "Drive Command Loop"
    n141 = node-c288() -> (→"Drive Comand Loop Late?":bool, →"Drive Command Loop Duration":i64)  [unwired: 1 in]
    n142 = Wait on Notification(notifier=w349, timeout in ms (-1)=0) -> (notification=w365:T16, timed out?=w366:bool)  [unwired: 2 in, 2 out]
    n143 = feedback #6(Drive_Commands."Manual" ("notification")) -> (w362:T16)
    n144 = case shown="True" w366 {
      tunnel: w365 -> [w383 _]
      tunnel: w367 -> [w378 w458]
      tunnel: w362 -> [_ w457]
      tunnel: [w383 w457] -> w361
      tunnel: [w382 w451] -> w360
      tunnel: [w381 w450] -> w359
      tunnel: w358 -> [w374 w453]
      tunnel: w357 -> [w375 w452]
      tunnel: [w380 w445] -> w356
      tunnel: [w379 w444] -> w355
      tunnel: w354 -> [_ w449]
      tunnel: w353 -> [_ w448]
      tunnel: w349 -> [_ w446]
      tunnel: [w377 w443] -> w352
      tunnel: w351 -> [w376 w443]
      frame False {
        n145 = case shown="\"Turn To Angle\"" w383 {
          tunnel: [_ _ w386 _ w395 _] -> w382
          tunnel: [_ _ w387 _ w394 _] -> w381
          tunnel: [_ _ w389 _ w393 _] -> w380
          tunnel: [_ _ w388 _ w392 _] -> w379
          tunnel: w378 -> [_ _ _ _ _ w440]
          tunnel: [_ _ w385 _ w391 w439] -> w377
          tunnel: w376 -> [_ _ w390 _ _ _]
          tunnel: w375 -> [_ _ w387 _ _ _]
          tunnel: w374 -> [_ _ w386 _ _ _]
          frame "Manual", Default {
          }
          frame "Get Gear" {
          }
          frame "Score Gear" {
            n146 = local read "Initial dAngle"() -> (w384:dbl)
            n147 = Add(x=w384, y=w390) -> (x+y=w385:dbl)
            n148 = shared-variable ".\\Sensors.lvlib\\Right Encoder Distance"() -> (w388:dbl)  [unwired: 1 in, 1 out]
            n149 = shared-variable ".\\Sensors.lvlib\\Left Encoder"() -> (w389:dbl)  [unwired: 1 in, 1 out]
          }
          frame "Align Rope" {
          }
          frame "Turn To Angle" {
            n150 = disable-structure shown="Disabled" {
              disable-tunnel: [w425 _] -> w395
              disable-tunnel: [w424 _] -> w394
              disable-tunnel: [w423 _] -> w393
              disable-tunnel: [w422 _] -> w392
              disable-tunnel: [w408 _] -> w391
              frame Disabled {
                w399 = 1.57 ("Body IMU Yaw")
                # "posative\nnegative"
                n151 = shared-variable ".\\Vision Variables.lvlib\\GearYPoints"() -> (w401:dbl[])  [unwired: 1 in, 1 out]
                n152 = shared-variable ".\\Vision Variables.lvlib\\GearXPoints"() -> (w402:dbl[])  [unwired: 1 in, 1 out]
                n153 = shared-variable ".\\Sensors.lvlib\\Body IMU Yaw"() -> (w407:dbl)  [unwired: 1 in, 1 out]
                n154 = shared-variable ".\\Vision Variables.lvlib\\DeltaGear"() -> (w410:dbl)  [unwired: 1 in, 1 out]
                n155 = local read "Initial dAngle"() -> (w397:dbl)
                n156 = Not(x="Invert Angle") -> (.not. x?=w405:bool)
                n157 = Negate(x=w410) -> (-x=w411:dbl)
                n158 = Select(t=w411, s=w405, f=w410) -> (s? t:f=w409:dbl)
                n159 = expression code="(x/180.0)*pi" "degrees to radians"(w397) -> (w396:dbl)
                n160 = expression code="(x/180.0)*pi" "degrees to radians"(w409) -> (w403:dbl)
                n161 = Add(x=w399, y=w396) -> (x+y=w398:dbl)
                n162 = Add(x=w403, y=w398) -> (x+y=w400:dbl)
                n163 = expression code="(x/pi)*180.0" "radians to degrees"(w400) -> (w406:dbl)
                n164 = call "ArcAndTheta.vi"("Limit of Orientation Change"="Limit of Orientation Change", "Amount of Time (s)"="Amount of Time (s)", "Absolute Theta Final"=w399, "Absolute Theta initial"=w400, "Y"=w401, "X"=w402) -> ("Theta(arc length)"=w413:dbl[], "Arc Length"=w416:dbl[], "TimeStamp"=w414:dbl[], "Verify Graph"=→"PlaceGearSpline":cluster{"X":dbl, "Y":dbl}[])  [unwired: 2 in]
                n165 = Subtract(x=w407, y=w406) -> (x-y=w408:dbl)
                n166 = shared-variable ".\\Sensors.lvlib\\Right Encoder Distance"() -> (w422:dbl)  [unwired: 1 in, 1 out]
                n167 = shared-variable ".\\Sensors.lvlib\\Left Encoder"() -> (w423:dbl)  [unwired: 1 in, 1 out]
                n168 = Build Cluster Array(w414, w416) -> (w415:cluster{dbl, dbl}[])
                n169 = Build Cluster Array(w414, w413) -> (w412:cluster{dbl, dbl}[])
                n170 = Array Size(array=w414) -> (size(s)=w418:i32)
                n171 = for {
                  N: "PID Segments (1-500)" -> [w438]
                  tunnel: w418 -> [w436]
                  tunnel: w415 -> [w430]
                  tunnel: [w428] -> w425 mode=indexing
                  tunnel: [w427] -> w424 mode=indexing
                  tunnel: w412 -> [w426]
                  i -> [w434]
                  n172 = Reciprocal(x=w438) -> (1/x=w437:dbl)
                  n173 = Increment(x=w434) -> (x+1=w433:i32)
                  n174 = Multiply(x=w437, y=w436) -> (x*y=w435:dbl)
                  n175 = Round Toward -Infinity(1:w435) -> (0:w432:dbl)
                  n176 = Multiply(x=w432, y=w433) -> (x*y=w431:dbl)
                  n177 = Decrement(x=w431) -> (x-1=w429:dbl)
                  n178 = Index Array(array=w430, index=w429) -> (element=w428:cluster{dbl, dbl})
                  n179 = Index Array(array=w426, index=w429) -> (element=w427:cluster{dbl, dbl})
                }
              }
              frame Enabled {
              }
            }
          }
          frame "Start Gear Score" {
            (unwired) FALSE ("Absolute Angle? in")
            n180 = call-poly <userlib>:"Drive_Loop_Command.vi"("Power/Rate Limit"=0.7 ("Power in"), "Drive Loop Cluster"=w440) -> ()  [unwired: 10 in]
            n181 = shared-variable ".\\Sensors.lvlib\\Body IMU Yaw"() -> (w439:dbl)  [unwired: 1 in, 1 out]
          }
        }
      }
      frame True {
        n182 = shared-variable ".\\ControlMode.lvlib\\Manual Mode?"() -> (w447:bool)  [unwired: 1 in, 1 out]
        n183 = feedback #7() -> (w455:T16)
        n184 = Select(t=Drive_Commands."Manual", s=w447, f=w457) -> (s? t:f=w442:T16)
        n185 = feedback-in #7(w442) -> ()
        n186 = Not Equal?(x=w442, y=w455) -> (x != y?=w454:bool)
        n187 = case shown="\"Place Gear\"" w442 {
          tunnel: w458 -> [w479 _ w525 w550 w562 w581 w589 w654 w656]
          tunnel: w454 -> [_ _ w517 _ w561 _ w587 _ w655]
          tunnel: w453 -> [_ _ w519 _ w553 _ _ _ _]
          tunnel: w452 -> [_ _ w518 _ w552 _ _ _ _]
          tunnel: [_ _ w519 _ w553 _ _ _ _] -> w451
          tunnel: [_ _ w518 _ w552 _ _ _ _] -> w450
          tunnel: w449 -> [_ _ w521 _ _ _ _ _ _]
          tunnel: w448 -> [_ _ w520 _ _ _ _ _ _]
          tunnel: w446 -> [_ _ w511 _ w554 w583 w588 _ _]
          tunnel: w443 -> [_ _ w514 _ w551 _ _ _ _]
          tunnel: [_ _ w520 _ _ _ _ _ _] -> w445
          tunnel: [_ _ w521 _ _ _ _ _ _] -> w444
          frame "Manual", Default {
            n188 = shared-variable ".\\DriverController.lvlib\\RightStickX"() -> (w481:dbl)  [unwired: 1 in, 1 out]
            n189 = shared-variable ".\\DriverController.lvlib\\LeftStickY"() -> (w482:dbl)  [unwired: 1 in, 1 out]
            n190 = First Call?() -> (First Call?: T/F=w476:bool)
            n191 = Or(x="Update PIDS", y=w476) -> (x .or. y?=w477:bool)
            n192 = case shown="True" w477 {
              tunnel: w479 -> [_ w484]
              frame False {
              }
              frame True {
                n193 = call <userlib>:"Drive_Loop_PID_Update.vi"("PID Gains"="PID Gains", "Control Cluster"=w484) -> ()  [unwired: 10 in]
              }
            }
            n194 = case shown="2" "Switch Case" {
              tunnel: w479 -> [w488 w492 w500]
              tunnel: w482 -> [w487 _ _]
              tunnel: w481 -> [w486 _ _]
              tunnel: "Send Command" -> [_ w491 w499]
              tunnel: [0.0 ("Angle in") w490 0.0 ("Angle in")] -> w473
              frame 0, Default {
                n195 = call-poly <userlib>:"Drive_Loop_Command.vi"("Wheel"=w486, "Throttle"=w487, "Drive Loop Cluster"=w488) -> ()  [unwired: 9 in]
              }
              frame 1 {
                n196 = feedback #8() -> (w489:dbl)  [unwired: 1 in]
                n197 = case shown="True" w491 {
                  tunnel: w492 -> [_ w497]
                  tunnel: [w493 "Angle in"] -> w490
                  tunnel: w489 -> [w493 _]
                  frame False {
                  }
                  frame True {
                    n198 = call-poly <userlib>:"Drive_Loop_Command.vi"("Absolute Angle? in"=FALSE, "Angle in"="Angle in", "Power in"="Power in", "Drive Loop Cluster"=w497) -> ()  [unwired: 8 in]
                  }
                }
                n199 = feedback-in #8(w490) -> ()
              }
              frame 2 {
                n200 = case shown="True" w499 {
                  tunnel: w500 -> [_ w505]
                  frame False {
                  }
                  frame True {
                    n201 = call-poly <userlib>:"Drive_Loop_Command.vi"("Distance"="Distance", "Absolute Angle? 4"=FALSE, "Angle 3"="Angle 3", "Power 3"="Power 3", "Drive Loop Cluster"=w505) -> ()  [unwired: 7 in]
                  }
                }
              }
            }
            n202 = shared-variable ".\\Sensors.lvlib\\Body IMU Yaw"() -> (w468:dbl)  [unwired: 1 in, 1 out]
            n203 = feedback #9() -> (w463:bool)  [unwired: 1 in]
            n204 = call <userlib>:"De-Bounce_or_Delay.vi"("Eval Period (sec)"=4.0, "Signal Input"=w463) -> ("Stable"=w460:bool)  [unwired: 9 in]
            "Done?" <- w460
            n205 = Or(x="Reset S and H", y=w460) -> (x .or. y?=w462:bool)
            n206 = call <userlib>:"JK_Latch.vi"("Reset"=w462, "Set"="Send Command") -> ("Q"=w470:bool)  [unwired: 5 in]
            n207 = feedback #10() -> (w475:dbl)  [unwired: 1 in]
            n208 = Select(t=w475, s=w470, f=w468) -> (s? t:f=w474:dbl)
            n209 = feedback-in #10(w474) -> ()
            n210 = Add(x=w473, y=w474) -> (x+y=w469:dbl)
            n211 = Subtract(x=w469, y=w468) -> (x-y=w467:dbl)
            n212 = Absolute Value(x=w467) -> (abs(x)=w466:dbl)
            "Diff" <- w466
            n213 = Bundle(w469, "Double"=w468) -> (→"PID Response":cluster{dbl, "Double":dbl})  [unwired: 1 in]
            n214 = Less?(x=w466, y="PID Reset Tolerance") -> (x < y?=w464:bool)
            n215 = feedback-in #9(w464) -> ()
          }
          frame "Get Gear" {
          }
          frame "Score Gear" {
            n216 = shared-variable ".\\Sensors.lvlib\\Right Encoder Distance"() -> (w528:dbl)  [unwired: 1 in, 1 out]
            n217 = shared-variable ".\\Sensors.lvlib\\Left Encoder"() -> (w530:dbl)  [unwired: 1 in, 1 out]
            n218 = shared-variable ".\\Sensors.lvlib\\Body IMU Yaw"() -> (w516:dbl)  [unwired: 1 in, 1 out]
            n219 = Subtract(x=w516, y=w514) -> (x-y=w515:dbl)
            n220 = Subtract(x=w528, y=w520) -> (x-y=w527:dbl)
            n221 = Subtract(x=w530, y=w521) -> (x-y=w529:dbl)
            n222 = expression code="(x/180.0)*pi" "degrees to radians"(w515) -> (w542:dbl)
            n223 = Add(x=w527, y=w529) -> (x+y=w535:dbl)
            n224 = call <vilib>:"PID Setpoint Profile.vi"("reinitialize? (F)"=w517, "setpoint profile"=w519) -> ("profile complete?"=w510:bool, "setpoint"=w537:dbl)  [unwired: 4 in, 2 out]
            n225 = Divide(x=w535, y=2.0) -> (x/y=w532:dbl)
            n226 = call <vilib>:"PID Setpoint Profile.vi"("reinitialize? (F)"=w517, "setpoint profile"=w518) -> ("profile complete?"=w509:bool, "setpoint"=w541:dbl)  [unwired: 4 in, 2 out]
            n227 = call-poly <vilib>:"PID.vi"("output range"="Speed Range", "PID gains"="PID Speed gains", "process variable"=w532, "setpoint"=w537) -> ("output"=w526:dbl)  [unwired: 6 in, 1 out]
            n228 = Bundle(w532, "setpoint"=w537) -> (→"Arc Length Chart":cluster{dbl, "setpoint":dbl})  [unwired: 1 in]
            n229 = Bundle(w542, "setpoint"=w541) -> (→"Angle Chart (rad)":cluster{dbl, "setpoint":dbl})  [unwired: 1 in]
            n230 = call-poly <vilib>:"PID.vi"("reinitialize? (F)"=w517, "output range"="Steer Range", "PID gains"="PID Steer gains", "process variable"=w542, "setpoint"=w541) -> ("output"=w538:dbl)  [unwired: 5 in, 1 out]
            n231 = Negate(x=w526) -> (-x=w524:dbl)
            "throttle" <- w524
            n232 = Negate(x=w538) -> (-x=w523:dbl)
            "steer" <- w523
            n233 = And(x=w509, y=w510) -> (x .and. y?=w508:bool)
            n234 = call <userlib>:"Stable.vi"("Eval Period (sec)"=0.5, "Signal Input"=w508) -> ("Stable"=w507:bool)  [unwired: 9 in]
            n235 = Or(x="Done?", y=w507) -> (x .or. y?=w513:bool)
            n236 = case shown="True" w513 {
              tunnel: w525 -> [w545 _]
              tunnel: w524 -> [w544 _]
              tunnel: w523 -> [w543 _]
              tunnel: w511 -> [_ w547]
              frame False {
                n237 = call-poly <userlib>:"Drive_Loop_Command.vi"("Wheel"=w543, "Throttle"=w544, "Drive Loop Cluster"=w545) -> ()  [unwired: 9 in]
              }
              frame True {
                n238 = Send Notification(notification=Drive_Commands."Manual", notifier=w547) -> ()  [unwired: 1 in, 2 out]
              }
            }
          }
          frame "Align Rope" {
            n239 = shared-variable ".\\DriverController.lvlib\\RightStickX"() -> (w548:dbl)  [unwired: 1 in, 1 out]
            n240 = shared-variable ".\\DriverController.lvlib\\LeftStickY"() -> (w549:dbl)  [unwired: 1 in, 1 out]
            n241 = call-poly <userlib>:"Drive_Loop_Command.vi"("Wheel"=w548, "Throttle"=w549, "Drive Loop Cluster"=w550) -> ()  [unwired: 9 in]
          }
          frame "Turn To Angle" {
            n242 = case shown="True" w561 {
              tunnel: w562 -> [_ w573]
              tunnel: w551 -> [w567 w570]
              tunnel: [w567 w569] -> w559
              frame False {
              }
              frame True {
                n243 = shared-variable ".\\ControlMode.lvlib\\Turning Distance"() -> (w568:dbl)  [unwired: 1 in, 1 out]
                n244 = Add(x=w568, y=w570) -> (x+y=w569:dbl)
                n245 = call-poly <userlib>:"Drive_Loop_Command.vi"("Absolute Angle? in"=TRUE, "Angle in"=w568, "Power in"=0.7, "Drive Loop Cluster"=w573) -> ()  [unwired: 8 in]
              }
            }
            n246 = shared-variable ".\\Sensors.lvlib\\Body IMU Yaw"() -> (w560:dbl)  [unwired: 1 in, 1 out]
            n247 = Subtract(x=w560, y=w559) -> (x-y=w558:dbl)
            n248 = Absolute Value(x=w558) -> (abs(x)=w557:dbl)
            n249 = Less?(x=w557, y=2.0) -> (x < y?=w555:bool)
            n250 = disable-structure shown="Disabled" {
              disable-tunnel: w555 -> [w564 _]
              disable-tunnel: w554 -> [w563 _]
              frame Disabled {
                n251 = case shown="True" w564 {
                  tunnel: w563 -> [_ w566]
                  frame False {
                  }
                  frame True {
                    n252 = Send Notification(notification=Drive_Commands."Score Gear", notifier=w566) -> ()  [unwired: 1 in, 2 out]
                  }
                }
              }
              frame Enabled {
              }
            }
          }
          frame "Start Gear Score" {
            n253 = shared-variable ".\\Vision Variables.lvlib\\Gear yaw delta"() -> (w580:dbl)  [unwired: 1 in, 1 out]
            n254 = Absolute Value(x=w580) -> (abs(x)=w579:dbl)
            n255 = Less?(x=w579, y="Turn To Peg Tol. (deg)") -> (x < y?=w576:bool)
            n256 = call <userlib>:"Stable.vi"("Eval Period (sec)"="Camera Align Stable", "Signal Input"=w576) -> ("Stable"=w575:bool)  [unwired: 9 in]
            "Camera Align Done" <- w575
            n257 = case shown="True" w575 {
              tunnel: w583 -> [_ w586]
              tunnel: w581 -> [_ w584]
              frame False {
              }
              frame True {
                n258 = call-poly <userlib>:"Drive_Loop_Command.vi"("Drive Loop Cluster"=w584) -> ()  [unwired: 11 in]
                n259 = Send Notification(notification=Drive_Commands."Manual", notifier=w586) -> ()  [unwired: 1 in, 2 out]
              }
            }
            n260 = Bundle("abs(x)"=0.0, w579) -> (→"Turn To Camera":cluster{"abs(x)":dbl, dbl})  [unwired: 1 in]
          }
          frame "Place Gear" {
            n261 = disable-structure shown="Enabled" {
              disable-tunnel: w589 -> [w606 w650]
              disable-tunnel: w588 -> [w603 _]
              disable-tunnel: w587 -> [w595 w641]
              frame Disabled {
                n262 = call <userlib>:"Pulse_Stretch_&_Delay.vi"("Delay (sec)"=0.0, "In"=w595, "Width (sec)"=2.0) -> ("Out"=w594:bool)  [unwired: 2 in]
                n263 = feedback #11() -> (w601:dbl)  [unwired: 1 in]
                n264 = case shown="True" w594 {
                  tunnel: w606 -> [_ w615]
                  tunnel: [w609 w610] -> w602
                  tunnel: w601 -> [w609 _]
                  frame False {
                  }
                  frame True {
                    n265 = shared-variable ".\\Vision Variables.lvlib\\Gear Distance"() -> (w611:dbl)  [unwired: 1 in, 1 out]
                    n266 = Subtract(x=w611, y="Offset APpr 2") -> (x-y=w610:dbl)
                    n267 = call-poly <userlib>:"Drive_Loop_Command.vi"("Distance"=w610, "Absolute Angle?"=FALSE, "Power"="Power Place Gear  2", "Drive Loop Cluster"=w615) -> ()  [unwired: 8 in]
                  }
                }
                n268 = feedback-in #11(w602) -> ()
                n269 = call <userlib>:"Pulse_Stretch_&_Delay.vi"("Delay (sec)"=3.5, "In"=w595, "Width (sec)"=0.1) -> ("Out"=w598:bool)  [unwired: 2 in]
                n270 = Absolute Value(x=w602) -> (abs(x)=w605:dbl)
                n271 = shared-variable ".\\ToLog.lvlib\\BodyPriGood"() -> (w597:bool)  [unwired: 1 in, 1 out]
                n272 = Less?(x=w605, y=1.0) -> (x < y?=w591:bool)
                n273 = Not(x=w597) -> (.not. x?=w596:bool)
                n274 = Compound Arithmetic op=OR(w591, w598, w596) -> (w600:bool)
                n275 = case shown="True" w600 {
                  tunnel: w603 -> [_ w608]
                  frame False {
                  }
                  frame True {
                    n276 = Send Notification(notification=Drive_Commands."Manual", notifier=w608) -> ()  [unwired: 1 in, 2 out]
                  }
                }
              }
              frame Enabled {
                n277 = shared-variable ".\\Teleop_QCP.lvlib\\Gear_Deliver_Offset"() -> (w622:dbl)  [unwired: 1 in, 1 out]
                n278 = shared-variable ".\\Vision Variables.lvlib\\Gear Distance"() -> (w630:dbl)  [unwired: 1 in, 1 out]
                n279 = shared-variable ".\\Vision Variables.lvlib\\Gear valid"() -> (w623:bool)  [unwired: 1 in, 1 out]
                n280 = feedback-in #12(w630) -> ()
                n281 = feedback #12() -> (w629:dbl)  [unwired: 1 in]
                n282 = shared-variable ".\\Sensors.lvlib\\Left Encoder"() -> (w636:dbl)  [unwired: 1 in, 1 out]
                n283 = Equal?(x=w630, y=w629) -> (x = y?=w626:bool)
                n284 = shared-variable ".\\Teleop_QCP.lvlib\\Gear_Deliver_PID_High"() -> ()  [unwired: 1 in, 2 out]
                n285 = shared-variable ".\\Teleop_QCP.lvlib\\Gear_Deliver_PID_Low"() -> ()  [unwired: 1 in, 2 out]
                n286 = shared-variable ".\\ToLog.lvlib\\BodyPriGood"() -> (w651:bool)  [unwired: 1 in, 1 out]
                n287 = Not(x=w626) -> (.not. x?=w625:bool)
                n288 = shared-variable ".\\Teleop_QCP.lvlib\\Gear_Deliver_PID_P"() -> (w619:dbl)  [unwired: 1 in, 1 out]
                n289 = shared-variable ".\\Teleop_QCP.lvlib\\Gear_Delivery_PID_I"() -> (w618:dbl)  [unwired: 1 in, 1 out]
                n290 = shared-variable ".\\Teleop_QCP.lvlib\\Gear_Deliver_PID_D"() -> (w617:dbl)  [unwired: 1 in, 1 out]
                n291 = Subtract(x=w630, y=w622) -> (x-y=w642:dbl)
                n292 = Add(x=w642, y=w636) -> (x+y=w649:dbl)
                n293 = And(x=w625, y=w623) -> (x .and. y?=w627:bool)
                n294 = Not(x=w651) -> (.not. x?=w640:bool)
                n295 = feedback #13(w636) -> (w648:dbl)
                n296 = Select(t=w636, s=w641, f=w648) -> (s? t:f=w647:dbl)
                n297 = Select(t=w649, s=w627, f=w647) -> (s? t:f=w628:dbl)
                n298 = feedback-in #13(w628) -> ()
                n299 = Bundle By Name(cluster="Gear Place gains", "proportional gain (Kc)"=w619, "integral time (Ti, min)"=w618, "derivative time (Td, min)"=w617) -> (w620:T4)
                n300 = Subtract(x=w628, y=w636) -> (x-y=w635:dbl)
                n301 = Absolute Value(x=w635) -> (abs(x)=w624:dbl)
                n302 = call-poly <vilib>:"PID.vi"("output range"="output range", "PID gains"=w620, "process variable"=w636, "setpoint"=w628) -> ("output"=w644:dbl)  [unwired: 6 in, 1 out]
                n303 = Less?(x=w624, y=10.0) -> (x < y?=w633:bool)
                n304 = shared-variable ".\\DriverController.lvlib\\LeftStickY"() -> (w645:dbl)  [unwired: 1 in, 1 out]
                n305 = Bundle("Double"=w628, "Double"=w636) -> (→"Gear Delivery Graphs":cluster{"Double":dbl, "Double":dbl})  [unwired: 1 in]
                n306 = Negate(x=w645) -> (-x=w643:dbl)
                n307 = Max & Min(x=w644, y=w643) -> (min(x,y)=w638:dbl)  [unwired: 1 out]
                n308 = call <userlib>:"De-Bounce_or_Delay.vi"("Eval Period (sec)"=0.3, "Signal Input"=w633) -> ("Stable"=w632:bool)  [unwired: 9 in]
                n309 = shared-variable ".\\Sensors.lvlib\\Gear Distance Within Tol"(w632) -> ()  [unwired: 1 in, 1 out]
                n310 = Select(t=0.0, s=w640, f=w638) -> (s? t:f=w637:dbl)
                n311 = call-poly <userlib>:"Drive_Loop_Command.vi"("Power Level #6"=w637, "Drive Loop Cluster"=w650) -> ()  [unwired: 10 in]
              }
            }
          }
          frame "Tank Drive" {
            n312 = shared-variable ".\\Notifiers.lvlib\\Right"() -> (w652:dbl)  [unwired: 1 in, 1 out]
            n313 = shared-variable ".\\Notifiers.lvlib\\Left"() -> (w653:dbl)  [unwired: 1 in, 1 out]
            n314 = call-poly <userlib>:"Drive_Loop_Command.vi"("Right"=w652, "Left"=w653, "Drive Loop Cluster"=w654) -> ()  [unwired: 9 in]
          }
          frame "Drive Distance" {
            n315 = case shown="True" w655 {
              tunnel: w656 -> [_ w659]
              frame False {
              }
              frame True {
                n316 = shared-variable ".\\ControlMode.lvlib\\Drive Distance Dist"() -> (w661:dbl)  [unwired: 1 in, 1 out]
                n317 = call-poly <userlib>:"Drive_Loop_Command.vi"("Distance"=w661, "Absolute Angle? 4"=FALSE, "Angle 3"=0.0, "Power 3"=0.6, "Drive Loop Cluster"=w659) -> ()  [unwired: 7 in]
              }
            }
          }
        }
      }
    }
    n318 = feedback-in #6(w361) -> ()
    n319 = case shown="True" "Start Score Gear" {
      tunnel: w349 -> [_ w373]
      frame False {
      }
      frame True {
        n320 = Send Notification(notification=Drive_Commands."Turn To Angle", notifier=w373) -> ()  [unwired: 1 in, 2 out]
      }
    }
    n321 = node-c288("Drive Command Period") -> ()  [unwired: 1 out]
  }
  n322 = node-c288() -> (w51:T30)  [unwired: 4 in]
  n323 = node-c288() -> (w85:T30)  [unwired: 4 in]
  n324 = timed-loop {
    timing: w51 -> [_]
    timing-out: [_] -> w50
    tunnel: w49 -> [w703]
    stop <- FALSE stop-if-true
    # "Match Time Notifier Loop"
    n325 = node-c288() -> (→"Match Time Loop Late?":bool, →"Match Time Loop Duration":i64)  [unwired: 1 in]
    n326 = call <vilib>:"WPI_DriverStationGetRemainingMatchTime.vi"() -> ("Match Time(s)"=w682:sgl)  [unwired: 10 in, 1 out]
    n327 = call <vilib>:"WPI_DriverStationGetModeAndStatus.vi"() -> ("Robot Mode"=w705:T39)  [unwired: 10 in, 1 out]
    n328 = Less?(x=w682, y=sgl 60.0) -> (x < y?=w698:bool)
    n329 = Less?(x=w682, y=sgl 30.0) -> (x < y?=w702:bool)
    n330 = Less?(x=w682, y=sgl 1.0) -> (x < y?=w694:bool)
    n331 = Less?(x=w682, y=sgl 10.0) -> (x < y?=w684:bool)
    n332 = Equal?(x=w705, y=WPI_DriverStationRobotMode2."Teleop Enabled") -> (x = y?=w681:bool)
    n333 = call <userlib>:"Signal_Pulse.vi"("Input"=w698) -> ("Output"=w692:bool)
    n334 = call <userlib>:"Signal_Pulse.vi"("Input"=w702) -> ("Output"=w701:bool)
    n335 = call <userlib>:"Signal_Pulse.vi"("Input"=w694) -> ("Output"=w693:bool)
    n336 = call <userlib>:"Signal_Pulse.vi"("Input"=w684) -> ("Output"=w685:bool)
    n337 = shared-variable ".\\ToLog.lvlib\\Robot Mode"(w705) -> ()  [unwired: 1 in, 1 out]
    n338 = And(x=w681, y=w692) -> (x .and. y?=w691:bool)
    n339 = And(x=w681, y=w701) -> (x .and. y?=w690:bool)
    n340 = And(x=w681, y=w693) -> (x .and. y?=w680:bool)
    n341 = And(x=w681, y=w685) -> (x .and. y?=w677:bool)
    n342 = Select(t=MatchTimeNotifications."thirtySecondsLeft", s=w690, f=MatchTimeNotifications."matchOver") -> (s? t:f=w679:T38)
    n343 = Compound Arithmetic op=OR(w691, w690, w677, w680) -> (w697:bool)
    n344 = Select(t=MatchTimeNotifications."tenSecondsLeft", s=w677, f=w679) -> (s? t:f=w678:T38)
    n345 = call <vilib>:"WPI_Power Get roboRIO Input Voltage and Current.vi"() -> ("roboRIO input voltage (V)"=w668:dbl)  [unwired: 13 in, 2 out]
    n346 = call <userlib>:"Signal_Pulse.vi"("Input"=w697) -> ("Output"=w686:bool)
    n347 = call <vilib>:"WPI_DriverStationGet Alliance Info.vi"() -> ("Alliance"=w671:T37)  [unwired: 10 in, 1 out]
    n348 = shared-variable ".\\ToLog.lvlib\\roboRIO input voltage (V)"(w668) -> ()  [unwired: 1 in, 1 out]
    n349 = Select(t=MatchTimeNotifications."oneMinuteLeft", s=w691, f=w678) -> (s? t:f=w672:T38)
    n350 = case shown="True" w686 {
      tunnel: w703 -> [_ w713]
      tunnel: w672 -> [_ w714]
      frame False {
      }
      frame True {
        w711 = 0
        n351 = case shown="\"oneMinuteLeft\", Default" w714 {
          tunnel: [60 30 10 0] -> w710
          frame "oneMinuteLeft", Default {
          }
          frame "thirtySecondsLeft" {
          }
          frame "tenSecondsLeft" {
          }
          frame "matchOver" {
          }
        }
        n352 = Build Array(T40."timeWarn" ("Enum"), w710, w711, w711) -> (w709:i32[])
        n353 = Send Notification(notification=w709, notifier=w713) -> ()  [unwired: 1 in, 2 out]
      }
    }
    n354 = Equal?(x=WPI_DriverStationAllianceInfo."Blue", y=w671) -> (x = y?=w669:bool)
    n355 = shared-variable ".\\Auto Variables.lvlib\\Blue Alliance?"(w669) -> ()  [unwired: 1 in, 1 out]
    n356 = node-c288("Match Time Period") -> ()  [unwired: 1 out]
  }
  n357 = timed-loop {
    timing: w85 -> [_]
    timing-out: [_] -> w84
    i -> [w728]
    stop <- _ stop-if-true
    # "Boiler Dist Average Loop"
    n358 = node-c288() -> (→"Boiler Dist Late?":bool, →"Boiler Dist Duration":i64)  [unwired: 1 in]
    n359 = shared-variable ".\\ControlMode.lvlib\\ShootingMode"() -> (w730:bool)  [unwired: 1 in, 1 out]
    n360 = shared-variable ".\\Vision Variables.lvlib\\Boiler distance"() -> (w731:dbl)  [unwired: 1 in, 1 out]
    n361 = feedback #14() -> (w729:i32)  [unwired: 1 in]
    n362 = Select(t=w729, s=w730, f=w728) -> (s? t:f=w727:i32)
    n363 = feedback-in #14(w727) -> ()
    n364 = Subtract(x=w728, y=w727) -> (x-y=w726:i32)
    n365 = feedback #15() -> (w732:dbl[])  [unwired: 1 in]
    n366 = case shown="True" w730 {
      tunnel: w732 -> [_ w743]
      tunnel: [w738 w746] -> w735
      tunnel: [w737 w740] -> w725
      tunnel: w731 -> [w736 w739]
      tunnel: w726 -> [_ w742]
      frame False {
        w738 = 1 ("dimension size")
        n367 = Initialize Array(w736, w738) -> (w737:dbl[])
      }
      frame True {
        n368 = Quotient & Remainder(x=w742, y="Max Buff Size") -> (x-y*floor(x/y)=w745:i32)  [unwired: 1 out]
        n369 = Insert Into Array(array=w743, index=w745, new element=w739) -> (w741:dbl[])
        n370 = Delete From Array(array=w741, index="Max Buff Size") -> (array with subset deleted=w740:dbl[])  [unwired: 1 in, 1 out]
        n371 = Array Size(array=w740) -> (size(s)=w746:i32)
      }
    }
    n372 = feedback-in #15(w725) -> ()
    n373 = Add Array Elements(numeric array=w725) -> (sum=w733:dbl)
    n374 = Divide(x=w733, y=w735) -> (x/y=w734:dbl)
    n375 = shared-variable ".\\Vision Variables.lvlib\\Boiler Distance Averaged"(w734) -> ()  [unwired: 1 in, 1 out]
    n376 = node-c288("Boiler Dist Period") -> ()  [unwired: 1 out]
  }
  n377 = while {
    stop <- FALSE stop-if-true
    n378 = shared-variable ".\\Teleop_QCP.lvlib\\Turret_CCW_Bound"() -> (w753:dbl)  [unwired: 1 in, 1 out]
    n379 = shared-variable ".\\Teleop_QCP.lvlib\\Turret_CW_Bound"() -> (w754:dbl)  [unwired: 1 in, 1 out]
    n380 = shared-variable ".\\Base Parameters.lvlib\\TurretCWBound"(w754) -> ()  [unwired: 1 in, 1 out]
    n381 = shared-variable ".\\Base Parameters.lvlib\\TurretCCWBound"(w753) -> ()  [unwired: 1 in, 1 out]
    n382 = Wait (ms)(milliseconds to wait=u32 300) -> ()  [unwired: 1 out]
  }
  n383 = node-c288(w114) -> ()  [unwired: 1 out]
  n384 = node-c288(w89) -> ()  [unwired: 1 out]
  n385 = Get Date/Time In Seconds() -> (seconds since 1Jan1904=w25:timestamp)
  n386 = node-c288(w84) -> ()  [unwired: 1 out]
  n387 = node-c288(w50) -> ()  [unwired: 1 out]
  n388 = node-c288() -> (w46:T30)  [unwired: 5 in]
  n389 = timed-loop {
    timing: w46 -> [_]
    timing-out: [_] -> w45
    tunnel: w44 -> [w844]
    tunnel: w41 -> [w781]
    stop <- FALSE stop-if-true
    w808 = 0.0
    # "Top Wheel"
    n390 = node-c288() -> (→"Top Duration":i64, →"Top Late?":bool)  [unwired: 1 in]
    n391 = shared-variable ".\\Teleop_QCP.lvlib\\Top_Wheel_Enc_Counts"() -> (w763:dbl)  [unwired: 1 in, 1 out]
    n392 = shared-variable ".\\Teleop_QCP.lvlib\\Top_Wheel_Blue_Mul"() -> (w765:dbl)  [unwired: 1 in, 1 out]
    n393 = shared-variable ".\\Teleop_QCP.lvlib\\Top_Wheel_Red_Mul"() -> (w764:dbl)  [unwired: 1 in, 1 out]
    n394 = shared-variable ".\\ControlMode.lvlib\\Fixed RPM Mode"() -> (w758:bool)  [unwired: 1 in, 1 out]
    n395 = shared-variable ".\\ControlMode.lvlib\\Fixed Top RPM"() -> (w759:dbl)  [unwired: 1 in, 1 out]
    n396 = disable-structure shown="Enabled" {
      disable-tunnel: [w846 w849] -> w767
      frame Disabled {
        n397 = shared-variable ".\\Vision Variables.lvlib\\Boiler Distance Averaged"() -> (w847:dbl)  [unwired: 1 in, 1 out]
        n398 = Add(x=w847, y=1.5) -> (x+y=w846:dbl)
      }
      frame Enabled {
        n399 = shared-variable ".\\Vision Variables.lvlib\\Boiler Distance Averaged"() -> (w850:dbl)  [unwired: 1 in, 1 out]
        n400 = shared-variable ".\\Teleop_QCP.lvlib\\Vision_Boiler_Offset"() -> (w848:dbl)  [unwired: 1 in, 1 out]
        n401 = Add(x=w848, y=w850) -> (x+y=w849:dbl)
      }
    }
    n402 = shared-variable ".\\Auto Variables.lvlib\\Blue Alliance?"() -> (w757:bool)  [unwired: 1 in, 1 out]
    n403 = shared-variable ".\\Vision Variables.lvlib\\Boiler Found"() -> (w787:bool)  [unwired: 1 in, 1 out]
    n404 = shared-variable ".\\ControlMode.lvlib\\ShootingMode"() -> (w791:bool)  [unwired: 1 in, 1 out]
    n405 = Select(t=w765, s=w757, f=w764) -> (s? t:f=w782:dbl)
    n406 = Wait on Occurrence(2:w781, 3:0 ("ms timeout (-1)")) -> (0:w779:bool)  [unwired: 1 in]
    n407 = Not(x=w779) -> (.not. x?=w778:bool)
    n408 = shared-variable ".\\OperatorController.lvlib\\OpRightY"() -> (w769:dbl)  [unwired: 1 in, 1 out]
    n409 = call <userlib>:"Bump_Counter.vi"("ref"=w767, "cntrl"=w769, "quanta"=0.5, "reset"=w778) -> ("out"=w766:dbl, "Bumps"=w770:dbl)  [unwired: 1 in]
    n410 = Or(x="TopFrontPanelMode?", y=w791) -> (x .or. y?=w784:bool)
    n411 = shared-variable ".\\ToLog.lvlib\\ShooterTopBumps"(w770) -> ()  [unwired: 1 in, 1 out]
    n412 = call "ShooterLUT.vi"("Distance from Boiler"=w766) -> ("Top RPM"=w786:dbl)  [unwired: 9 in, 1 out]
    n413 = feedback #16() -> (w793:dbl)  [unwired: 1 in]
    n414 = Select(t=w786, s=w787, f=w793) -> (s? t:f=w792:dbl)
    n415 = Multiply(x=w792, y=w782) -> (x*y=w760:dbl)
    n416 = Select(t=w759, s=w758, f=w760) -> (s? t:f=w761:dbl)
    n417 = Select(t="Top Cntrl", s="TopFrontPanelMode?", f=w761) -> (s? t:f=w768:dbl)
    "Top Cntrl ." <- w768
    n418 = case shown="True" w784 {
      tunnel: w844 -> [w906 w927]
      tunnel: "Disable Top" -> [_ _]
      tunnel: w768 -> [_ w923]
      tunnel: [_ w925] -> _
      tunnel: [_ w918] -> w796
      tunnel: [_ w926] -> w795
      tunnel: "Top Open" -> [_ w919]
      tunnel: w763 -> [_ w913]
      frame False {
        n419 = call <vilib>:"WPI_CANTalonSRX_ChangeMode.vi"("Output"=0.6, "Control Mode"=WPI_CANTalonSRX_APIControlMode."Percent VBus", "CAN Talon SRX Ref"=w906) -> ()  [unwired: 7 in, 2 out]
      }
      frame True {
        n420 = call <vilib>:"WPI_CANTalonSRX_SetReference.vi"("Reverse Closed-Loop Output"="Reverse Closed-Loop Output", "Reverse Feedback Sensor"="Rev FB Sensor 2", "Feedback Reference"=WPI_CANTalonSRX_APIFeedbackSelect."Digital Quadrature Encoder", "CAN Talon SRX Ref"=w927) -> ("CAN Talon SRX Ref"=w933:T21)  [unwired: 6 in, 1 out]
        n421 = First Call?() -> (First Call?: T/F=w914:bool)
        n422 = Divide(x=w913, y=600.0) -> (x/y=w928:dbl)
        n423 = Or(x="TuneTopPID", y=w914) -> (x .or. y?=w916:bool)
        n424 = shared-variable ".\\Teleop_QCP.lvlib\\Top_Wheel_I_Zone"() -> (w912:dbl)  [unwired: 1 in, 1 out]
        n425 = shared-variable ".\\Teleop_QCP.lvlib\\Top_Wheel_PID_D"() -> (w911:dbl)  [unwired: 1 in, 1 out]
        n426 = Multiply(x=w928, y=w923) -> (x*y=w922:dbl)
        n427 = shared-variable ".\\Teleop_QCP.lvlib\\Top_Wheel_Ramp_Rate"() -> (w907:dbl)  [unwired: 1 in, 1 out]
        n428 = Negate(x=w922) -> (-x=w920:dbl)
        n429 = shared-variable ".\\Teleop_QCP.lvlib\\Top_Wheel_PID_F"() -> (w910:dbl)  [unwired: 1 in, 1 out]
        n430 = shared-variable ".\\Teleop_QCP.lvlib\\Top_Wheel_PID_P"() -> (w908:dbl)  [unwired: 1 in, 1 out]
        n431 = shared-variable ".\\Teleop_QCP.lvlib\\Top_Wheel_PID_I"() -> (w909:dbl)  [unwired: 1 in, 1 out]
        n432 = case shown="False" w916 {
          tunnel: [w936 w945] -> w935
          tunnel: w933 -> [w936 w944]
          tunnel: w908 -> [_ w943]
          tunnel: w909 -> [_ w942]
          tunnel: w911 -> [_ w941]
          tunnel: w912 -> [_ w940]
          tunnel: w907 -> [_ w939]
          tunnel: w910 -> [_ w938]
          tunnel: u8 0 ("Parameter Slot") -> [_ w937]
          frame False {
          }
          frame True {
            n433 = call <vilib>:"WPI_CANTalonSRX_SetPID.vi"("CAN Talon SRX Ref"=w944, "Parameter Slot"=w937, "P"=w943, "I"=w942, "D"=w941, "F"=w938, "I Zone"=w940, "Ramp Rate"=w939) -> ("CAN Talon SRX Ref"=w945:T21)  [unwired: 6 in, 1 out]
          }
        }
        n434 = case shown="False" w919 {
          tunnel: w935 -> [w949 w953]
          tunnel: [w948 w952] -> w934
          tunnel: w920 -> [_ w950]
          frame True {
            n435 = call <vilib>:"WPI_CANTalonSRX_ChangeMode.vi"("Output"="Output", "Control Mode"=WPI_CANTalonSRX_APIControlMode."Percent VBus", "CAN Talon SRX Ref"=w949) -> ("CAN Talon SRX Ref"=w948:T21)  [unwired: 7 in, 1 out]
          }
          frame False {
            n436 = call <vilib>:"WPI_CANTalonSRX_ChangeMode.vi"("Output"=w950, "Control Mode"=WPI_CANTalonSRX_APIControlMode."Speed", "CAN Talon SRX Ref"=w953) -> ("CAN Talon SRX Ref"=w952:T21)  [unwired: 7 in, 1 out]
          }
        }
        n437 = call <vilib>:"WPI_CANTalonSRX_GetStatus.vi"("CAN Talon SRX Ref"=w934) -> ("Talon SRX Status"=w932:T42)  [unwired: 8 in, 2 out]
        n438 = Unbundle By Name(w932) -> ("Encoder Velocity"=w924:dbl, "Applied Throttle"=w925:dbl, "Encoder Position"=w926:dbl)
        n439 = Divide(x=w924, y=w928) -> (x/y=w918:dbl)
      }
    }
    "Top Dist" <- w795
    "Top Dist ." <- w795
    n440 = feedback-in #16(w792) -> ()
    n441 = call <vilib>:"WPI_DriverStationGetModeAndStatus.vi"() -> ("Robot Mode"=w776:T39)  [unwired: 10 in, 1 out]
    n442 = feedback #17(FALSE) -> (w772:bool)
    n443 = Equal?(x=w776, y=WPI_DriverStationRobotMode2."Teleop Enabled") -> (x = y?=w773:bool)
    n444 = feedback-in #17(w773) -> ()
    n445 = Greater?(x=w773, y=w772) -> (0:w774:bool)
    n446 = case shown="True" w774 {
      frame False {
      }
      frame True {
        n447 = shared-variable ".\\ControlMode.lvlib\\Fixed RPM Mode"(FALSE ("ShootingMode")) -> ()  [unwired: 1 in, 1 out]
        n448 = shared-variable ".\\ControlMode.lvlib\\ShootingMode"(FALSE ("ShootingMode")) -> ()  [unwired: 1 in, 1 out]
      }
    }
    n449 = feedback #18(w808) -> (w816:dbl)
    n450 = Select(t=-inf, s="reset top", f=w816) -> (s? t:f=w815:dbl)
    n451 = Max & Min(x=w796, y=w815) -> (max(x,y)=w817:dbl)  [unwired: 1 out]
    "Max top" <- w817
    n452 = feedback-in #18(w817) -> ()
    n453 = shared-variable ".\\Teleop_QCP.lvlib\\Top_Wheel_RPM_Tol"() -> (w762:dbl)  [unwired: 1 in, 1 out]
    n454 = Bundle("Double"=w768, w796) -> ()  [unwired: 1 in, 1 out]
    n455 = feedback #19(w808) -> (w811:dbl)
    n456 = Select(t=inf, s="reset top", f=w811) -> (s? t:f=w813:dbl)
    n457 = Max & Min(x=w796, y=w813) -> (min(x,y)=w812:dbl)  [unwired: 1 out]
    "Min Top" <- w812
    n458 = feedback-in #19(w812) -> ()
    n459 = Add(x=w768, y=w762) -> (x+y=w820:dbl)
    n460 = Subtract(x=w768, y=w762) -> (x-y=w819:dbl)
    n461 = Subtract(x=w768, y=w796) -> (x-y=w840:dbl)
    n462 = Less Than 0?(x=w840) -> (x < 0?=→"RPM High":bool)
    n463 = Greater Than 0?(x=w840) -> (x > 0?=→"RPM Low":bool)
    n464 = Absolute Value(x=w840) -> (abs(x)=w837:dbl)
    n465 = In Range and Coerce(upper limit=w820, x=w796, lower limit=w819) -> (In Range?=w789:bool)  [unwired: 1 out]
    n466 = shared-variable ".\\ControlMode.lvlib\\ShootingMode"() -> (w790:bool)  [unwired: 1 in, 1 out]
    n467 = Less Or Equal?(x=w837, y=1.0) -> (x <= y?=→"1 RPM":bool)
    n468 = Less Or Equal?(x=w837, y=2.0) -> (x <= y?=→"2 RPM":bool)
    n469 = Less Or Equal?(x=w837, y=3.0) -> (x <= y?=→"3 RPM":bool)
    n470 = Less Or Equal?(x=w837, y=4.0) -> (x <= y?=→"4 RPM":bool)
    n471 = Less Or Equal?(x=w837, y=5.0) -> (x <= y?=→"5 RPM":bool)
    n472 = Less Or Equal?(x=w837, y=6.0) -> (x <= y?=→"6 RPM":bool)
    n473 = Less Or Equal?(x=w837, y=7.0) -> (x <= y?=→"7 RPM":bool)
    n474 = Less Or Equal?(x=w837, y=8.0) -> (x <= y?=→"8 RPM":bool)
    n475 = And(x=w789, y=w790) -> (x .and. y?=w788:bool)
    n476 = shared-variable ".\\Sensors.lvlib\\Top Wheel Steady"(w788) -> ()  [unwired: 1 in, 1 out]
    n477 = feedback #20(0) -> (w802:i32)
    "State1" <- w802
    n478 = feedback #21(w802) -> (w801:i32)
    n479 = feedback-in #21(w802) -> ()
    n480 = case shown="0, Default" w802 {
      selector: w802 -> [w859 w894 _]
      tunnel: w796 -> [w865 w885 w903]
      tunnel: [w881 w889 w902] -> w799
      tunnel: "Arm" -> [w880 _ _]
      tunnel: "Trig" -> [w861 _ _]
      tunnel: w801 -> [w860 w893 _]
      tunnel: "Len" -> [_ w891 _]
      tunnel: [w865 w885 w903] -> w806
      tunnel: "Reset1" -> [w857 _ w899]
      tunnel: [TRUE TRUE FALSE] -> w805
      frame 0, Default {
        w879 = 0
        n481 = Less?(x=w859, y=w860) -> (x < y?=w858:bool)
        n482 = Or(x=w857, y=w858) -> (x .or. y?=w856:bool)
        n483 = feedback #22(-inf) -> (w871:dbl)
        n484 = Select(t=w865, s=w856, f=w871) -> (s? t:f=w870:dbl)
        n485 = Max & Min(x=w865, y=w870) -> (max(x,y)=w877:dbl)  [unwired: 1 out]
        n486 = feedback-in #22(w877) -> ()
        n487 = feedback #23(inf) -> (w869:dbl)
        n488 = Select(t=w865, s=w856, f=w869) -> (s? t:f=w868:dbl)
        n489 = Max & Min(x=w865, y=w868) -> (min(x,y)=w876:dbl)  [unwired: 1 out]
        n490 = Add(x=w876, y=w877) -> (x+y=w875:dbl)
        n491 = Divide(x=w875, y=2.0) -> (x/y=w864:dbl)
        n492 = feedback-in #23(w876) -> ()
        n493 = Add(x=w861, y=w864) -> (x+y=w867:dbl)
        n494 = Subtract(x=w864, y=w861) -> (x-y=w866:dbl)
        n495 = In Range and Coerce(upper limit=w867, x=w865, lower limit=w866) -> (In Range?=w863:bool)  [unwired: 1 out]
        n496 = Not(x=w863) -> (.not. x?=w862:bool)
        "Tgrd" <- w862
        n497 = Select(t=1, s=w862, f=w879) -> (s? t:f=w882:i32)
        n498 = Select(t=w882, s=w880, f=w879) -> (s? t:f=w881:i32)
      }
      frame 1 {
        w896 = i16 0
        n499 = Greater?(x=w894, y=w893) -> (0:w892:bool)
        n500 = feedback #24(w896) -> (w897:i16)
        n501 = Select(t=w896, s=w892, f=w897) -> (s? t:f=w895:i16)
        n502 = Increment(x=w895) -> (x+1=w890:i16)
        "cnt" <- w890
        n503 = feedback-in #24(w890) -> ()
        n504 = Greater Or Equal?(x=w890, y=w891) -> (x >= y?=w886:bool)
        n505 = Select(t=2, s=w886, f=1) -> (s? t:f=w889:i32)
      }
      frame 2 {
        n506 = Select(t=0, s=w899, f=2) -> (s? t:f=w902:i32)
      }
    }
    n507 = feedback-in #20(w799) -> ()
    n508 = case shown="True" w805 {
      tunnel: w806 -> [_ w855]
      tunnel: w768 -> [_ w853]
      frame False {
      }
      frame True {
        n509 = Bundle(w855, "Double"=w853) -> (→"Top Response":cluster{dbl, "Double":dbl})  [unwired: 1 in]
      }
    }
    n510 = shared-variable ".\\ToLog.lvlib\\TopShooterResponse"(w806) -> ()  [unwired: 1 in, 1 out]
    n511 = shared-variable ".\\ToLog.lvlib\\TopShooterCtrl"(w768) -> ()  [unwired: 1 in, 1 out]
    n512 = node-c288("Top Period") -> ()  [unwired: 1 in, 1 out]
  }
  n513 = node-c288(w118) -> ()  [unwired: 1 out]
  n514 = while {
    shift-right: [w962] -> _
    shift-left: 0 -> [w963]
    shift-right: [w960] -> _
    shift-left: w25 -> [w961]
    stop <- FALSE stop-if-true
    # "Gear Mech Zero"
    n515 = case shown="0, Default" w963 {
      selector: w963 -> [w968 w974 _]
      tunnel: [w967 w973 0] -> w962
      tunnel: w961 -> [_ w976 _]
      tunnel: [w966 w972 w983] -> w960
      frame 0, Default {
        n516 = shared-variable ".\\DriverController.lvlib\\A"() -> (w970:bool)  [unwired: 1 in, 1 out]
        n517 = Increment(x=w968) -> (x+1=w969:i32)
        n518 = Select(t=w969, s=w970, f=w968) -> (s? t:f=w967:i32)
        n519 = Get Date/Time In Seconds() -> (seconds since 1Jan1904=w966:timestamp)
      }
      frame 1 {
        n520 = Get Date/Time In Seconds() -> (seconds since 1Jan1904=w977:timestamp)
        n521 = To Double Precision Float(number=w976) -> (double precision float=w981:dbl)
        n522 = To Double Precision Float(number=w977) -> (double precision float=w982:dbl)
        n523 = shared-variable ".\\Teleop_QCP.lvlib\\Gear_Zero_Down_Time"() -> (w971:dbl)  [unwired: 1 in, 1 out]
        n524 = Subtract(x=w982, y=w981) -> (x-y=w979:dbl)
        n525 = shared-variable ".\\Notifiers.lvlib\\DropGearmMech"(TRUE ("ZeroGearMech")) -> ()  [unwired: 1 in, 1 out]
        n526 = Greater?(x=w979, y=w971) -> (0:w978:bool)
        n527 = Select(t=w977, s=w978, f=w976) -> (s? t:f=w972:timestamp)
        n528 = Increment(x=w974) -> (x+1=w975:i32)
        n529 = Select(t=w975, s=w978, f=w974) -> (s? t:f=w973:i32)
      }
      frame 2 {
        n530 = shared-variable ".\\Notifiers.lvlib\\ZeroGearMech"() -> (w984:refnum<k4>)  [unwired: 1 in, 1 out]
        n531 = shared-variable ".\\Notifiers.lvlib\\DropGearmMech"(FALSE ("ZeroGearMech")) -> ()  [unwired: 1 in, 1 out]
        n532 = Set Occurrence(w984) -> ()
        n533 = Get Date/Time In Seconds() -> (seconds since 1Jan1904=w983:timestamp)
      }
    }
    n534 = Wait (ms)(milliseconds to wait=u32 50) -> ()  [unwired: 1 out]
  }
  n535 = node-c288(w116) -> ()  [unwired: 1 out]
  n536 = node-c288() -> (w48:T30)  [unwired: 4 in]
  n537 = timed-loop {
    timing: w48 -> [_]
    timing-out: [_] -> w47
    tunnel: w121 -> [w1072]
    tunnel: w42 -> [w1005]
    stop <- FALSE stop-if-true
    w1036 = -inf
    w1035 = inf
    # "Bottom Wheel"
    n538 = node-c288() -> (→"Bottom Wheel Duration":i64, →"Bottom Wheel Late?":bool)  [unwired: 1 in]
    n539 = disable-structure shown="Enabled" {
      disable-tunnel: [w1074 w1077] -> w998
      frame Disabled {
        n540 = shared-variable ".\\Vision Variables.lvlib\\Boiler Distance Averaged"() -> (w1075:dbl)  [unwired: 1 in, 1 out]
        n541 = Add(x=w1075, y=1.5) -> (x+y=w1074:dbl)
      }
      frame Enabled {
        n542 = shared-variable ".\\Vision Variables.lvlib\\Boiler Distance Averaged"() -> (w1078:dbl)  [unwired: 1 in, 1 out]
        n543 = shared-variable ".\\Teleop_QCP.lvlib\\Vision_Boiler_Offset"() -> (w1076:dbl)  [unwired: 1 in, 1 out]
        n544 = Add(x=w1078, y=w1076) -> (x+y=w1077:dbl)
      }
    }
    n545 = shared-variable ".\\Teleop_QCP.lvlib\\Bot_Wheel_Blue_Mul"() -> (w996:dbl)  [unwired: 1 in, 1 out]
    n546 = shared-variable ".\\OperatorController.lvlib\\OpRightY"() -> (w1006:dbl)  [unwired: 1 in, 1 out]
    n547 = shared-variable ".\\ControlMode.lvlib\\Fixed RPM Mode"() -> (w990:bool)  [unwired: 1 in, 1 out]
    n548 = shared-variable ".\\ControlMode.lvlib\\FixedBottomRPM"() -> (w987:dbl)  [unwired: 1 in, 1 out]
    n549 = shared-variable ".\\ControlMode.lvlib\\Tuning Mode?"() -> (w993:bool)  [unwired: 1 in, 1 out]
    n550 = shared-variable ".\\Vision Variables.lvlib\\Boiler Found"() -> (w1016:bool)  [unwired: 1 in, 1 out]
    n551 = Wait on Occurrence(2:w1005, 3:0 ("ms timeout (-1)")) -> (0:w1002:bool)  [unwired: 1 in]
    n552 = Negate(x=w1006) -> (-x=w1001:dbl)
    n553 = Not(x=w1002) -> (.not. x?=w1003:bool)
    n554 = Select(t="Bottom Multiplier Blue", s=w993, f=w996) -> (s? t:f=w994:dbl)
    n555 = call <userlib>:"Bump_Counter.vi"("ref"=w998, "cntrl"=w1001, "quanta"=0.5, "reset"=w1003) -> ("out"=w997:dbl, "Bumps"=w1000:dbl)  [unwired: 1 in]
    n556 = shared-variable ".\\ToLog.lvlib\\ShooterBotBumps"(w1000) -> ()  [unwired: 1 in, 1 out]
    n557 = shared-variable ".\\Auto Variables.lvlib\\Blue Alliance?"() -> (w1008:bool)  [unwired: 1 in, 1 out]
    n558 = shared-variable ".\\ControlMode.lvlib\\ShootingMode"() -> (w1015:bool)  [unwired: 1 in, 1 out]
    n559 = shared-variable ".\\Teleop_QCP.lvlib\\Bot_Wheel_Red_Mul"() -> (w992:dbl)  [unwired: 1 in, 1 out]
    n560 = call "ShooterLUT.vi"("Distance from Boiler"=w997) -> ("Bottom RPM"=w1014:dbl)  [unwired: 9 in, 1 out]
    n561 = feedback #25() -> (w1010:dbl)  [unwired: 1 in]
    n562 = Select(t=w1014, s=w1016, f=w1010) -> (s? t:f=w1020:dbl)
    n563 = feedback-in #25(w1020) -> ()
    n564 = Or(x=w1015, y="BotFrontPanel") -> (x .or. y?=w1012:bool)
    n565 = Select(t=w994, s=w1008, f=w992) -> (s? t:f=w1009:dbl)
    n566 = Multiply(x=w1010, y=w1009) -> (x*y=w989:dbl)
    n567 = Select(t=w987, s=w990, f=w989) -> (s? t:f=w988:dbl)
    n568 = Select(t="Bot Cntrl", s="BotFrontPanel", f=w988) -> (s? t:f=w999:dbl)
    n569 = case shown="True" w1012 {
      tunnel: w1072 -> [w1130 w1156]
      tunnel: w999 -> [_ w1146]
      tunnel: "Disable Bottom" -> [_ _]
      tunnel: "Open?" -> [_ w1145]
      tunnel: "Open Loop Cntrl" -> [_ w1144]
      tunnel: [_ w1151] -> _
      tunnel: [_ w1143] -> w1024
      tunnel: [_ w1146] -> w1023
      tunnel: [_ w1147] -> w1022
      frame False {
        n570 = call <vilib>:"WPI_CANTalonSRX_ChangeMode.vi"("Output"=-0.3, "Control Mode"=WPI_CANTalonSRX_APIControlMode."Percent VBus", "CAN Talon SRX Ref"=w1130) -> ()  [unwired: 7 in, 2 out]
      }
      frame True {
        n571 = shared-variable ".\\Teleop_QCP.lvlib\\Bot_Wheel_Enc_Counts"() -> (w1139:dbl)  [unwired: 1 in, 1 out]
        n572 = First Call?() -> (First Call?: T/F=w1140:bool)
        n573 = shared-variable ".\\Teleop_QCP.lvlib\\Bot_Wheel_I_Zone"() -> (w1138:dbl)  [unwired: 1 in, 1 out]
        n574 = shared-variable ".\\Teleop_QCP.lvlib\\Bot_Wheel_PID_F"() -> (w1136:dbl)  [unwired: 1 in, 1 out]
        n575 = shared-variable ".\\Teleop_QCP.lvlib\\Bot_Wheel_PID_P"() -> (w1134:dbl)  [unwired: 1 in, 1 out]
        n576 = shared-variable ".\\Teleop_QCP.lvlib\\Bot_Wheel_PID_I"() -> (w1135:dbl)  [unwired: 1 in, 1 out]
        n577 = shared-variable ".\\Teleop_QCP.lvlib\\Bot_Wheel_PID_D"() -> (w1137:dbl)  [unwired: 1 in, 1 out]
        n578 = shared-variable ".\\Teleop_QCP.lvlib\\Bot_Wheel_Ramp_Rate"() -> (w1133:dbl)  [unwired: 1 in, 1 out]
        n579 = call <vilib>:"WPI_CANTalonSRX_SetReference.vi"("Reverse Feedback Sensor"="Rev FB Sensor", "Feedback Reference"=WPI_CANTalonSRX_APIFeedbackSelect."Digital Quadrature Encoder", "CAN Talon SRX Ref"=w1156) -> ("CAN Talon SRX Ref"=w1160:T21)  [unwired: 7 in, 1 out]
        n580 = Or(x=w1140, y="TuneBotPID") -> (x .or. y?=w1142:bool)
        n581 = Divide(x=w1139, y=600.0) -> (x/y=w1154:dbl)
        n582 = case shown="False" w1142 {
          tunnel: [w1163 w1171] -> w1162
          tunnel: w1160 -> [w1163 w1170]
          tunnel: w1134 -> [_ w1169]
          tunnel: w1135 -> [_ w1168]
          tunnel: w1137 -> [_ w1167]
          tunnel: w1138 -> [_ w1166]
          tunnel: w1133 -> [_ w1165]
          tunnel: w1136 -> [_ w1164]
          frame False {
          }
          frame True {
            n583 = call <vilib>:"WPI_CANTalonSRX_SetPID.vi"("CAN Talon SRX Ref"=w1170, "P"=w1169, "I"=w1168, "D"=w1167, "F"=w1164, "I Zone"=w1166, "Ramp Rate"=w1165) -> ("CAN Talon SRX Ref"=w1171:T21)  [unwired: 7 in, 1 out]
          }
        }
        n584 = Multiply(x=w1154, y=w1146) -> (x*y=w1150:dbl)
        n585 = Negate(x=w1150) -> (-x=w1149:dbl)
        n586 = case shown="True" w1145 {
          tunnel: w1162 -> [w1175 w1179]
          tunnel: [w1174 w1178] -> w1161
          tunnel: w1149 -> [_ w1176]
          tunnel: w1144 -> [w1172 _]
          frame True {
            n587 = call <vilib>:"WPI_CANTalonSRX_ChangeMode.vi"("Output"=w1172, "Control Mode"=WPI_CANTalonSRX_APIControlMode."Percent VBus", "CAN Talon SRX Ref"=w1175) -> ("CAN Talon SRX Ref"=w1174:T21)  [unwired: 7 in, 1 out]
          }
          frame False {
            n588 = call <vilib>:"WPI_CANTalonSRX_ChangeMode.vi"("Output"=w1176, "Control Mode"=WPI_CANTalonSRX_APIControlMode."Speed", "CAN Talon SRX Ref"=w1179) -> ("CAN Talon SRX Ref"=w1178:T21)  [unwired: 7 in, 1 out]
          }
        }
        n589 = call <vilib>:"WPI_CANTalonSRX_GetStatus.vi"("CAN Talon SRX Ref"=w1161) -> ("Talon SRX Status"=w1159:T42)  [unwired: 8 in, 2 out]
        n590 = Unbundle By Name(w1159) -> ("Encoder Velocity"=w1153:dbl, "Applied Throttle"=w1151:dbl, "Encoder Position"=w1147:dbl)
        n591 = Negate(x=w1153) -> (-x=w1148:dbl)
        n592 = Divide(x=w1148, y=w1154) -> (x/y=w1152:dbl)
        n593 = Negate(x=w1152) -> (-x=w1143:dbl)
      }
    }
    "Bot Cntrl ." <- w1023
    "Bot Dist" <- w1022
    "Bot Dist ." <- w1022
    n594 = feedback #26(w1036) -> (w1042:dbl)
    n595 = Select(t=w1036, s="reset bot", f=w1042) -> (s? t:f=w1041:dbl)
    n596 = Max & Min(x=w1024, y=w1041) -> (max(x,y)=w1043:dbl)  [unwired: 1 out]
    "Max Bot" <- w1043
    n597 = feedback-in #26(w1043) -> ()
    n598 = feedback #27(w1035) -> (w1037:dbl)
    n599 = Select(t=w1035, s="reset bot", f=w1037) -> (s? t:f=w1040:dbl)
    n600 = Max & Min(x=w1024, y=w1040) -> (min(x,y)=w1038:dbl)  [unwired: 1 out]
    "Min Bot" <- w1038
    n601 = feedback-in #27(w1038) -> ()
    n602 = shared-variable ".\\Teleop_QCP.lvlib\\Bot_Wheel_RPM_Tol"() -> (w991:dbl)  [unwired: 1 in, 1 out]
    n603 = Bundle("Double"=w1023, w1024) -> ()  [unwired: 1 in, 1 out]
    n604 = Add(x=w1023, y=w991) -> (x+y=w1067:dbl)
    n605 = Subtract(x=w1023, y=w991) -> (x-y=w1068:dbl)
    n606 = Subtract(x=w1023, y=w1024) -> (x-y=w1047:dbl)
    n607 = shared-variable ".\\ControlMode.lvlib\\ShootingMode"() -> (w1019:bool)  [unwired: 1 in, 1 out]
    n608 = Less Than 0?(x=w1047) -> (x < 0?=→"RPM High .":bool)
    n609 = Greater Than 0?(x=w1047) -> (x > 0?=→"RPM Low .":bool)
    n610 = Absolute Value(x=w1047) -> (abs(x)=w1050:dbl)
    n611 = In Range and Coerce(upper limit=w1067, x=w1024, lower limit=w1068) -> (In Range?=w1018:bool)  [unwired: 1 out]
    n612 = feedback #28(0) -> (w1030:i32)
    "State2" <- w1030
    n613 = feedback #29(w1030) -> (w1029:i32)
    n614 = feedback-in #29(w1030) -> ()
    n615 = case shown="0, Default" w1030 {
      selector: w1030 -> [w1085 w1120 _]
      tunnel: w1024 -> [w1091 w1111 w1129]
      tunnel: [w1107 w1115 w1128] -> w1027
      tunnel: "Arm2" -> [w1106 _ _]
      tunnel: "Trig2" -> [w1087 _ _]
      tunnel: w1029 -> [w1086 w1119 _]
      tunnel: "Len2" -> [_ w1117 _]
      tunnel: [w1091 w1111 w1129] -> w1034
      tunnel: "Reset2" -> [w1083 _ w1125]
      tunnel: [TRUE TRUE FALSE] -> w1033
      frame 0, Default {
        w1105 = 0
        n616 = Less?(x=w1085, y=w1086) -> (x < y?=w1084:bool)
        n617 = Or(x=w1083, y=w1084) -> (x .or. y?=w1082:bool)
        n618 = feedback #30(-inf) -> (w1097:dbl)
        n619 = Select(t=w1091, s=w1082, f=w1097) -> (s? t:f=w1096:dbl)
        n620 = Max & Min(x=w1091, y=w1096) -> (max(x,y)=w1103:dbl)  [unwired: 1 out]
        n621 = feedback-in #30(w1103) -> ()
        n622 = feedback #31(inf) -> (w1095:dbl)
        n623 = Select(t=w1091, s=w1082, f=w1095) -> (s? t:f=w1094:dbl)
        n624 = Max & Min(x=w1091, y=w1094) -> (min(x,y)=w1102:dbl)  [unwired: 1 out]
        n625 = Add(x=w1102, y=w1103) -> (x+y=w1101:dbl)
        n626 = Divide(x=w1101, y=2.0) -> (x/y=w1090:dbl)
        n627 = feedback-in #31(w1102) -> ()
        n628 = Add(x=w1087, y=w1090) -> (x+y=w1093:dbl)
        n629 = Subtract(x=w1090, y=w1087) -> (x-y=w1092:dbl)
        n630 = In Range and Coerce(upper limit=w1093, x=w1091, lower limit=w1092) -> (In Range?=w1089:bool)  [unwired: 1 out]
        n631 = Not(x=w1089) -> (.not. x?=w1088:bool)
        "Tgrd 2" <- w1088
        n632 = Select(t=1, s=w1088, f=w1105) -> (s? t:f=w1108:i32)
        n633 = Select(t=w1108, s=w1106, f=w1105) -> (s? t:f=w1107:i32)
      }
      frame 1 {
        w1122 = i16 0
        n634 = Greater?(x=w1120, y=w1119) -> (0:w1118:bool)
        n635 = feedback #32(w1122) -> (w1123:i16)
        n636 = Select(t=w1122, s=w1118, f=w1123) -> (s? t:f=w1121:i16)
        n637 = Increment(x=w1121) -> (x+1=w1116:i16)
        "cnt 2" <- w1116
        n638 = feedback-in #32(w1116) -> ()
        n639 = Greater Or Equal?(x=w1116, y=w1117) -> (x >= y?=w1112:bool)
        n640 = Select(t=2, s=w1112, f=1) -> (s? t:f=w1115:i32)
      }
      frame 2 {
        n641 = Select(t=0, s=w1125, f=2) -> (s? t:f=w1128:i32)
      }
    }
    n642 = feedback-in #28(w1027) -> ()
    n643 = And(x=w1018, y=w1019) -> (x .and. y?=w1017:bool)
    n644 = Less Or Equal?(x=w1050, y=1.0) -> (x <= y?=→"1 RPM .":bool)
    n645 = Less Or Equal?(x=w1050, y=2.0) -> (x <= y?=→"2 RPM .":bool)
    n646 = Less Or Equal?(x=w1050, y=3.0) -> (x <= y?=→"3 RPM .":bool)
    n647 = Less Or Equal?(x=w1050, y=4.0) -> (x <= y?=→"4 RPM .":bool)
    n648 = Less Or Equal?(x=w1050, y=5.0) -> (x <= y?=→"5 RPM .":bool)
    n649 = Less Or Equal?(x=w1050, y=6.0) -> (x <= y?=→"6 RPM .":bool)
    n650 = Less Or Equal?(x=w1050, y=7.0) -> (x <= y?=→"7 RPM .":bool)
    n651 = Less Or Equal?(x=w1050, y=8.0) -> (x <= y?=→"8 RPM .":bool)
    n652 = shared-variable ".\\Sensors.lvlib\\Bottom Wheel Steady"(w1017) -> ()  [unwired: 1 in, 1 out]
    n653 = shared-variable ".\\ToLog.lvlib\\BotShooterResponse"(w1034) -> ()  [unwired: 1 in, 1 out]
    n654 = case shown="True" w1033 {
      tunnel: w1034 -> [_ w1081]
      tunnel: w1023 -> [_ w1080]
      frame False {
      }
      frame True {
        n655 = Bundle(w1081, "Double"=w1080) -> (→"Bot Response":cluster{dbl, "Double":dbl})  [unwired: 1 in]
      }
    }
    n656 = shared-variable ".\\ToLog.lvlib\\BotShooterCtrl"(w1023) -> ()  [unwired: 1 in, 1 out]
    n657 = node-c288("Bot Period") -> ()  [unwired: 1 in, 1 out]
  }
  n658 = node-c288(i64 20 ("Period")) -> (w40:T30)  [unwired: 3 in]
  n659 = disable-structure shown="Enabled" {
    disable-tunnel: [w1190 w1194] -> w57
    disable-tunnel: [w1188 w1194] -> w2
    disable-tunnel: [w1186 w1192] -> w4
    frame Disabled {
      n660 = call <vilib>:"WPI_AnalogChannelOpen.vi"("Analog Channel"=FPGA_AIChannel."AI 2") -> ("AIDeviceRef"=w1186:T44)  [unwired: 9 in, 1 out]
      n661 = call <vilib>:"WPI_MotorControlRefNum Registry Get.vi"("refnum name"="Gear Riser") -> ("MotorControlDevRef"=w1190:T21)  [unwired: 9 in, 1 out]
      n662 = call <vilib>:"WPI_MotorControlRefNum Registry Get.vi"("refnum name"="BottomWheelRiserSensor") -> ("MotorControlDevRef"=w1188:T21)  [unwired: 9 in, 1 out]
    }
    frame Enabled {
      n663 = call <vilib>:"WPI_MotorControlRefNum Registry Get.vi"("refnum name"="GearRiser") -> ("MotorControlDevRef"=w1194:T21)  [unwired: 9 in, 1 out]
      n664 = call <vilib>:"WPI_AnalogChannelOpen.vi"("Analog Channel"=FPGA_AIChannel."AI 2") -> ("AIDeviceRef"=w1192:T44)  [unwired: 9 in, 1 out]
    }
  }
  n665 = shared-variable ".\\Notifiers.lvlib\\Home!"() -> (w62:refnum<k4>)  [unwired: 1 in, 1 out]
  n666 = call <vilib>:"WPI_MotorControlRefNum Registry Get.vi"("refnum name"="Intake") -> ("MotorControlDevRef"=w58:T21)  [unwired: 9 in, 1 out]
  n667 = call <vilib>:"WPI_CANTalonSRX_SetReference.vi"("Feedback Reference"=WPI_CANTalonSRX_APIFeedbackSelect."CTR Magnetic Enc (Absolute)", "CAN Talon SRX Ref"=w2) -> ("CAN Talon SRX Ref"=w3:T21)  [unwired: 8 in, 1 out]
  n668 = node-c288() -> (w61:T30)  [unwired: 4 in]
  n669 = shared-variable ".\\Notifiers.lvlib\\GearReceive Control DevRef"() -> (w92:T29)  [unwired: 1 in, 1 out]
  n670 = call <vilib>:"WPI_DigitalInputOpen.vi"("DIO Channel"=FPGA_DIOChannel."DIO 0") -> ("DigitalInputDevRef"=w63:T45)  [unwired: 9 in, 1 out]
  n671 = timed-loop {
    timing: w61 -> [_]
    timing-out: [_] -> w60
    tunnel: w58 -> [w1271]
    tunnel: w57 -> [w1231]
    tunnel: w3 -> [w1196]
    tunnel: w4 -> [w1209]
    stop <- FALSE stop-if-true
    n672 = node-c288() -> (→"Gear Mech Late?":bool, →"Gear Mech Duration":i64)  [unwired: 1 in]
    n673 = shared-variable ".\\Notifiers.lvlib\\ZeroGearMech"() -> (w1225:refnum<k4>)  [unwired: 1 in, 1 out]
    n674 = disable-structure shown="Disabled" {
      disable-tunnel: w1209 -> [w1279 _]
      frame Disabled {
        n675 = call <vilib>:"WPI_AnalogChannelGetVoltage.vi"("AIDeviceRef"=w1279) -> ("Voltage"=w1276:dbl)  [unwired: 8 in, 2 out]
        n676 = Subtract(x=w1276, y="Absolute Encoder Shift") -> (x-y=w1275:dbl)
        n677 = Multiply(x=w1275, y="Absolute Encoder Factor") -> ()  [unwired: 1 out]
      }
      frame Enabled {
      }
    }
    n678 = shared-variable ".\\ControlMode.lvlib\\Gear Intake Speed"() -> (w1238:dbl)  [unwired: 1 in, 1 out]
    n679 = First Call?() -> (First Call?: T/F=w1233:bool)
    n680 = Wait on Occurrence(1:FALSE ("ignore previous (T)"), 2:w1225, 3:0 ("ms timeout (-1)")) -> (0:w1223:bool)
    n681 = feedback-in #33(w1233) -> ()
    n682 = feedback #33() -> (w1232:bool)  [unwired: 1 in]
    n683 = call <vilib>:"WPI_CANTalonSRX_GetStatus.vi"("CAN Talon SRX Ref"=w1196) -> ("Talon SRX Status"=w1252:T42)  [unwired: 8 in, 2 out]
    n684 = shared-variable ".\\DriverController.lvlib\\RB"() -> ()  [unwired: 1 in, 2 out]
    n685 = Not(x=w1223) -> (.not. x?=w1222:bool)
    n686 = Unbundle By Name(w1252) -> ("Sensor Position"=w1251:dbl)
    n687 = feedback-in #34(w1238) -> ()
    n688 = feedback #34(0.0 ("Double")) -> (w1240:dbl)
    n689 = Compound Arithmetic op=OR(w1232, "ZERO SENSOR", w1222) -> (w1218:bool)
    n690 = call <userlib>:"Pulse_Stretch_&_Delay.vi"("In"=w1218, "Width (sec)"=1.0) -> ("Out"=→"Out":bool)  [unwired: 3 in]
    n691 = Less?(x=w1238, y=w1240) -> (x < y?=w1239:bool)
    n692 = shared-variable ".\\Teleop_QCP.lvlib\\Gear_Stall_Rate_Limit"() -> (w1201:dbl)  [unwired: 1 in, 1 out]
    n693 = shared-variable ".\\Teleop_QCP.lvlib\\Gear_Intake_PDP_Channel"() -> (w1207:dbl)  [unwired: 1 in, 1 out]
    n694 = shared-variable ".\\Teleop_QCP.lvlib\\Gear_Intake_PDP_Adr"() -> (w1208:dbl)  [unwired: 1 in, 1 out]
    n695 = Select(t=0.0, s=w1222, f=0.3 ("New Sensor Position")) -> (s? t:f=w1219:dbl)
    n696 = shared-variable ".\\Teleop_QCP.lvlib\\Gear_Stall_Thresh"() -> (w1200:dbl)  [unwired: 1 in, 1 out]
    n697 = Multiply(x=w1251, y="Factor") -> (x*y=w1198:dbl)
    "Sensor Position" <- w1198
    n698 = shared-variable ".\\Teleop_QCP.lvlib\\Gear_Stall_Eval"() -> (w1202:dbl)  [unwired: 1 in, 1 out]
    n699 = case shown="True" w1218 {
      tunnel: w1196 -> [_ w1286]
      tunnel: w1219 -> [_ w1285]
      frame False {
      }
      frame True {
        n700 = call <vilib>:"WPI_CANTalonSRX_SetSensorPosition.vi"("New Sensor Position"=w1285, "CAN Talon SRX Ref"=w1286) -> ()  [unwired: 8 in, 2 out]
      }
    }
    n701 = call <vilib>:"WPI_Power Get PDP Currents.vi"("Power Distribution Panel (0)"=w1208, "PDP Channel"=w1207) -> ("current (A)"=w1260:dbl)  [unwired: 11 in, 2 out]
    n702 = shared-variable ".\\Teleop_QCP.lvlib\\Gear_Mech_PID_P"() -> ()  [unwired: 1 in, 2 out]
    n703 = shared-variable ".\\Teleop_QCP.lvlib\\Gear_Mech_PID_I"() -> ()  [unwired: 1 in, 2 out]
    n704 = shared-variable ".\\Teleop_QCP.lvlib\\Gear_Mech_PID_D"() -> ()  [unwired: 1 in, 2 out]
    n705 = call-poly <vilib>:"PID Output Rate Limiter.vi"("reinitialize? (F)"="reinitialize? (F)", "output rate (EGU/min)"=w1201, "initial output"=0.0 ("f"), "input (controller output)"=w1238) -> ("output"=w1256:dbl)  [unwired: 4 in, 1 out]
    n706 = Greater?(x=w1260, y=w1200) -> (0:w1259:bool)
    n707 = call <userlib>:"Stable.vi"("Eval Period (sec)"=w1202, "Signal Input"=w1259) -> ("Stable"=w1236:bool)  [unwired: 9 in]
    "Stable" <- w1236
    n708 = call <userlib>:"JK_Latch.vi"("Reset"=w1239, "Set"=w1236) -> ("Q"=w1253:bool)  [unwired: 5 in]
    n709 = shared-variable ".\\Sensors.lvlib\\Riser setpoint"() -> (w1243:dbl)  [unwired: 1 in, 1 out]
    n710 = Bundle("Double"=w1243, w1198) -> (→"Encoder Pos":cluster{"Double":dbl, dbl})  [unwired: 1 in]
    n711 = Greater?(x=w1198, y="Gear Overdone Thresh") -> (0:w1213:bool)
    n712 = shared-variable ".\\Teleop_QCP.lvlib\\Gear_Mech_PID_Low"() -> (w1203:dbl)  [unwired: 1 in, 1 out]
    n713 = shared-variable ".\\Teleop_QCP.lvlib\\Gear_Mech_PID_High"() -> (w1204:dbl)  [unwired: 1 in, 1 out]
    n714 = Select(t=0.0, s=w1253, f=w1256) -> (s? t:f=w1255:dbl)
    n715 = call <userlib>:"Pulse_Stretch_&_Delay.vi"("In"=w1236, "Width (sec)"=0.2 ("Delay (sec)")) -> ("Out"=w1235:bool)  [unwired: 3 in]
    n716 = call <userlib>:"Stable.vi"("Eval Period (sec)"="Eval Period (sec) 2", "Signal Input"=w1213) -> ("Stable"=w1210:bool)  [unwired: 9 in]
    n717 = call <userlib>:"Pulse_Stretch_&_Delay.vi"("Delay (sec)"=0.0, "In"=w1213, "Width (sec)"="Eval Period (sec) 2") -> ()  [unwired: 2 in, 1 out]
    n718 = call <vilib>:"WPI_MotorControlSetOutput.vi"("Output"=w1255, "MotorControlDevRef"=w1271) -> ()  [unwired: 7 in, 3 out]
    n719 = shared-variable ".\\Sensors.lvlib\\Gear Intake Stalled"(w1235) -> ()  [unwired: 1 in, 1 out]
    n720 = shared-variable ".\\Sensors.lvlib\\Gear Overdoned"(w1210) -> ()  [unwired: 1 in, 1 out]
    n721 = Bundle(cluster="output range 2", "output high"=w1204, "output low"=w1203) -> (w1205:cluster{"output high":dbl, "output low":dbl})
    n722 = call-poly <vilib>:"PID.vi"("output range"=w1205, "PID gains"="PID gains", "process variable"=w1198, "setpoint"=w1243) -> ("output"=w1245:dbl)  [unwired: 6 in, 1 out]
    n723 = Negate(x=w1245) -> (-x=w1244:dbl)
    n724 = Select(t=w1244, s="Invert", f=w1245) -> (s? t:f=w1248:dbl)
    n725 = shared-variable ".\\Notifiers.lvlib\\DropGearmMech"() -> (w1228:bool)  [unwired: 1 in, 1 out]
    n726 = Select(t=w1248, s="Closed", f="Open") -> (s? t:f=w1227:dbl)
    n727 = shared-variable ".\\Teleop_QCP.lvlib\\Gear_Zero_Down_Power"() -> (w1199:dbl)  [unwired: 1 in, 1 out]
    n728 = Select(t=w1199, s=w1228, f=w1227) -> (s? t:f=w1226:dbl)
    n729 = feedback #35(0) -> (w1265:i32)
    "State1 2" <- w1265
    n730 = feedback #36(w1265) -> (w1266:i32)
    n731 = feedback-in #36(w1265) -> ()
    n732 = case shown="1" w1265 {
      selector: w1265 -> [w1291 w1326 _]
      tunnel: w1260 -> [w1297 w1317 w1335]
      tunnel: [w1313 w1321 w1334] -> w1268
      tunnel: "Arm 2" -> [w1312 _ _]
      tunnel: "Trig 2" -> [w1293 _ _]
      tunnel: w1266 -> [w1292 w1325 _]
      tunnel: "Len 2" -> [_ w1323 _]
      tunnel: [w1297 w1317 w1335] -> w1261
      tunnel: "Reset1 2" -> [w1289 _ w1331]
      tunnel: [TRUE TRUE FALSE] -> w1262
      frame 0, Default {
        w1311 = 0
        n733 = Less?(x=w1291, y=w1292) -> (x < y?=w1290:bool)
        n734 = Or(x=w1289, y=w1290) -> (x .or. y?=w1288:bool)
        n735 = feedback #37(-inf) -> (w1303:dbl)
        n736 = Select(t=w1297, s=w1288, f=w1303) -> (s? t:f=w1302:dbl)
        n737 = Max & Min(x=w1297, y=w1302) -> (max(x,y)=w1309:dbl)  [unwired: 1 out]
        n738 = feedback-in #37(w1309) -> ()
        n739 = feedback #38(inf) -> (w1301:dbl)
        n740 = Select(t=w1297, s=w1288, f=w1301) -> (s? t:f=w1300:dbl)
        n741 = Max & Min(x=w1297, y=w1300) -> (min(x,y)=w1308:dbl)  [unwired: 1 out]
        n742 = Add(x=w1308, y=w1309) -> (x+y=w1307:dbl)
        n743 = Divide(x=w1307, y=2.0) -> (x/y=w1296:dbl)
        n744 = feedback-in #38(w1308) -> ()
        n745 = Add(x=w1293, y=w1296) -> (x+y=w1299:dbl)
        n746 = Subtract(x=w1296, y=w1293) -> (x-y=w1298:dbl)
        n747 = In Range and Coerce(upper limit=w1299, x=w1297, lower limit=w1298) -> (In Range?=w1295:bool)  [unwired: 1 out]
        n748 = Not(x=w1295) -> (.not. x?=w1294:bool)
        "Tgrd 3" <- w1294
        n749 = Select(t=1, s=w1294, f=w1311) -> (s? t:f=w1314:i32)
        n750 = Select(t=w1314, s=w1312, f=w1311) -> (s? t:f=w1313:i32)
      }
      frame 1 {
        w1328 = i16 0
        n751 = Greater?(x=w1326, y=w1325) -> (0:w1324:bool)
        n752 = feedback #39(w1328) -> (w1329:i16)
        n753 = Select(t=w1328, s=w1324, f=w1329) -> (s? t:f=w1327:i16)
        n754 = Increment(x=w1327) -> (x+1=w1322:i16)
        "cnt 3" <- w1322
        n755 = feedback-in #39(w1322) -> ()
        n756 = Greater Or Equal?(x=w1322, y=w1323) -> (x >= y?=w1318:bool)
        n757 = Select(t=2, s=w1318, f=1) -> (s? t:f=w1321:i32)
      }
      frame 2 {
        n758 = Select(t=0, s=w1331, f=2) -> (s? t:f=w1334:i32)
      }
    }
    n759 = feedback-in #35(w1268) -> ()
    n760 = disable-structure shown="Enabled" {
      disable-tunnel: w1231 -> [w1282 w1283]
      disable-tunnel: WPI_CANTalonSRX_APIControlMode."Percent VBus" ("Control Mode") -> [w1281 _]
      disable-tunnel: w1226 -> [w1280 w1284]
      frame Enabled {
        n761 = call <vilib>:"WPI_CANTalonSRX_ChangeMode.vi"("Output"=w1280, "Control Mode"=w1281, "CAN Talon SRX Ref"=w1282) -> ()  [unwired: 7 in, 2 out]
      }
      frame Disabled {
        n762 = call <vilib>:"WPI_MotorControlSetOutput.vi"("Output"=w1284, "MotorControlDevRef"=w1283) -> ()  [unwired: 7 in, 3 out]
      }
    }
    n763 = case shown="True" w1262 {
      tunnel: w1261 -> [_ w1287]
      frame False {
      }
      frame True {
        "Intake Motor Current" <- w1287
      }
    }
    n764 = node-c288("Gear Mech Period") -> ()  [unwired: 1 out]
  }
  n765 = call <userlib>:"Pneumatic_Control_Loop.vi"("Cluster in"=w92) -> ()  [unwired: 11 in]
  n766 = shared-variable ".\\Notifiers.lvlib\\Gear Receiver Command DevRef"() -> (w52:T25)  [unwired: 1 in, 1 out]
  n767 = node-c288() -> (w66:T30)  [unwired: 4 in]
  n768 = timed-loop {
    timing: w66 -> [_]
    timing-out: [_] -> w65
    tunnel: w63 -> [w1352]
    tunnel: w62 -> [w1347]
    stop <- _ stop-if-true
    # "Homing Sensor"
    n769 = node-c288() -> (→"Homing Sensor Late":bool, →"Homing Sensor Duration":i64)  [unwired: 1 in]
    n770 = call <vilib>:"WPI_DigitalInputGetValue.vi"("DigitalInputDevRef"=w1352) -> ("Value"=w1350:bool)  [unwired: 8 in, 2 out]
    "Home?" <- w1350
    n771 = feedback-in #40(w1350) -> ()
    n772 = feedback #40(TRUE ("Value")) -> (w1349:bool)
    n773 = Less?(x=w1350, y=w1349) -> (x < y?=w1348:bool)
    n774 = Or(x="Home Turret Sensor", y=w1348) -> (x .or. y?=w1343:bool)
    n775 = case shown="True" w1343 {
      tunnel: w1347 -> [_ w1353]
      frame False {
      }
      frame True {
        n776 = Set Occurrence(w1353) -> ()
      }
    }
    n777 = node-c288("Homing Sensor Period") -> ()  [unwired: 1 out]
  }
  n778 = node-c288(i64 50 ("Period")) -> (w29:T30)  [unwired: 3 in]
  n779 = timed-loop {
    timing: w29 -> [_]
    timing-out: [_] -> w28
    stop <- _ stop-if-true
    n780 = node-c288() -> ()  [unwired: 1 in, 1 out]
    n781 = call <vilib>:"WPI_Power Get PDP Currents.vi"("Power Distribution Panel (0)"=u8 1, "PDP Channel"="PDP Channel 2") -> ("current (A)"=→"current (A)":dbl, "all currents (A)"=→"all currents (A)":dbl[])  [unwired: 11 in, 1 out]
    n782 = node-c288() -> ()  [unwired: 1 in, 1 out]
  }
  n783 = node-c288(i64 20 ("Period")) -> (w55:T30)  [unwired: 3 in]
  n784 = timed-loop {
    shift-right: [w1373] -> _
    shift-left: Gear_Command."Home" -> [w1368]
    timing: w55 -> [_]
    timing-out: [_] -> w54
    tunnel: w52 -> [w1370]
    stop <- FALSE stop-if-true
    n785 = node-c288() -> ()  [unwired: 1 in, 1 out]
    n786 = feedback-in #41(w1368) -> ()
    n787 = feedback #41(w1368) -> (w1369:T46)
    n788 = Not Equal?(x=w1368, y=w1369) -> (x != y?=w1367:bool)
    n789 = shared-variable ".\\Teleop_QCP.lvlib\\Gear_Intake_Fwd_Speed"() -> (w1366:dbl)  [unwired: 1 in, 1 out]
    n790 = case shown="\"Score\"" w1368 {
      selector: w1368 -> [w1383 w1401 w1411 w1422]
      tunnel: [w1381 w1400 w1413 w1421] -> w1373
      tunnel: [w1377 w1390 w1402 w1418] -> w1372
      tunnel: [0.0 ("Riser setpoint") w1391 w1405 w1419] -> w1371
      tunnel: w1366 -> [_ w1391 w1405 _]
      tunnel: w1370 -> [w1379 _ w1404 _]
      tunnel: w1367 -> [w1378 _ w1403 _]
      frame "Home", Default {
        (unwired) 100.0 ("Riser setpoint")
        n791 = case shown="True" w1378 {
          tunnel: w1379 -> [_ w1388]
          frame False {
          }
          frame True {
            n792 = call-poly <userlib>:"Pneumatics_Command_Set.vi"("Solenoid Command"=Pneumatics_Command."Reverse", "Cluster"=w1388) -> ()  [unwired: 9 in, 1 out]
          }
        }
        n793 = shared-variable ".\\Notifiers.lvlib\\Gear Command Notifier"() -> (w1387:refnum<notifier>)  [unwired: 1 in, 1 out]
        n794 = Wait on Notification(notifier=w1387, timeout in ms (-1)=0) -> (notifier out=w1380:refnum<notifier>, notification=w1382:T46, timed out?=w1384:bool)  [unwired: 2 in, 1 out]
        n795 = Cancel Notification(0:w1380) -> ()  [unwired: 1 in, 3 out]
        n796 = Select(t=w1383, s=w1384, f=w1382) -> (s? t:f=w1381:T46)
        n797 = shared-variable ".\\Teleop_QCP.lvlib\\Gear_Home_Pos"() -> (w1377:dbl)  [unwired: 1 in, 1 out]
      }
      frame "Floor Intake" {
        (unwired) 0.0 ("Riser setpoint")
        n798 = shared-variable ".\\Notifiers.lvlib\\Gear Command Notifier"() -> (w1398:refnum<notifier>)  [unwired: 1 in, 1 out]
        n799 = shared-variable ".\\Sensors.lvlib\\Gear Intake Stalled"() -> (w1395:bool)  [unwired: 1 in, 1 out]
        n800 = Wait on Notification(notifier=w1398, timeout in ms (-1)=0) -> (notifier out=w1392:refnum<notifier>, timed out?=w1397:bool)  [unwired: 2 in, 2 out]
        n801 = Cancel Notification(0:w1392) -> ()  [unwired: 1 in, 3 out]
        n802 = Not(x=w1397) -> (.not. x?=w1396:bool)
        n803 = Or(x=w1396, y=w1395) -> (x .or. y?=w1394:bool)
        n804 = shared-variable ".\\Teleop_QCP.lvlib\\Gear_Intake_Pos"() -> (w1390:dbl)  [unwired: 1 in, 1 out]
        n805 = Select(t=Gear_Command."Home", s=w1394, f=w1401) -> (s? t:f=w1400:T46)
      }
      frame "Catch" {
        n806 = shared-variable ".\\Sensors.lvlib\\Gear Intake Stalled"() -> (w1407:bool)  [unwired: 1 in, 1 out]
        n807 = case shown="True" w1403 {
          tunnel: w1404 -> [_ w1417]
          frame False {
          }
          frame True {
            n808 = call-poly <userlib>:"Pneumatics_Command_Set.vi"("Solenoid Command"=Pneumatics_Command."Forward", "Cluster"=w1417) -> ()  [unwired: 9 in, 1 out]
          }
        }
        n809 = shared-variable ".\\Notifiers.lvlib\\Gear Command Notifier"() -> (w1415:refnum<notifier>)  [unwired: 1 in, 1 out]
        n810 = Wait on Notification(notifier=w1415, timeout in ms (-1)=0) -> (notifier out=w1412:refnum<notifier>, timed out?=w1409:bool)  [unwired: 2 in, 2 out]
        n811 = Not(x=w1409) -> (.not. x?=w1408:bool)
        n812 = Or(x=w1407, y=w1408) -> (x .or. y?=w1406:bool)
        n813 = shared-variable ".\\Teleop_QCP.lvlib\\Gear_Catch_Pos"() -> (w1402:dbl)  [unwired: 1 in, 1 out]
        n814 = Select(t=Gear_Command."Home", s=w1406, f=w1411) -> (s? t:f=w1413:T46)
        n815 = Cancel Notification(0:w1412) -> ()  [unwired: 1 in, 3 out]
      }
      frame "Score" {
        (unwired) 35.0 ("Riser setpoint")
        n816 = shared-variable ".\\Notifiers.lvlib\\Gear Command Notifier"() -> (w1426:refnum<notifier>)  [unwired: 1 in, 1 out]
        n817 = shared-variable ".\\Teleop_QCP.lvlib\\Gear_Intake_Rev_Speed"() -> (w1419:dbl)  [unwired: 1 in, 1 out]
        n818 = Wait on Notification(notifier=w1426, timeout in ms (-1)=0) -> (notifier out=w1420:refnum<notifier>, notification=w1423:T46, timed out?=w1424:bool)  [unwired: 2 in, 1 out]
        n819 = Cancel Notification(0:w1420) -> ()  [unwired: 1 in, 3 out]
        n820 = shared-variable ".\\Teleop_QCP.lvlib\\Gear_Score_Pos"() -> (w1418:dbl)  [unwired: 1 in, 1 out]
        n821 = Select(t=w1422, s=w1424, f=w1423) -> (s? t:f=w1421:T46)
      }
    }
    n822 = shared-variable ".\\ControlMode.lvlib\\Gear Intake Speed"(w1371) -> ()  [unwired: 1 in, 1 out]
    n823 = shared-variable ".\\Sensors.lvlib\\Riser setpoint"(w1372) -> ()  [unwired: 1 in, 1 out]
    n824 = node-c288() -> ()  [unwired: 1 in, 1 out]
  }
  n825 = shared-variable ".\\Notifiers.lvlib\\Drive Command Notifier"() -> (w97:refnum<notifier>)  [unwired: 1 in, 1 out]
  n826 = node-c288(w65) -> ()  [unwired: 1 out]
  n827 = node-c288(w45) -> ()  [unwired: 1 out]
  n828 = node-c288(w28) -> ()  [unwired: 1 out]
  n829 = node-c288(w47) -> ()  [unwired: 1 out]
  n830 = shared-variable ".\\Notifiers.lvlib\\Drive Command Notifier"() -> (w32:refnum<notifier>)  [unwired: 1 in, 1 out]
  n831 = call <vilib>:"WPI_MotorControlRefNum Registry Get.vi"("refnum name"="Climb") -> ("MotorControlDevRef"=w101:T21)  [unwired: 9 in, 1 out]
  n832 = node-c288(w54) -> ()  [unwired: 1 out]
  n833 = node-c288(w60) -> ()  [unwired: 1 out]
  n834 = node-c288(i64 40 ("Period")) -> (w104:T30)  [unwired: 3 in]
  n835 = shared-variable ".\\Notifiers.lvlib\\NeoPixel Controls"() -> (w36:refnum<notifier>)  [unwired: 1 in, 1 out]
  n836 = while {
    stop <- FALSE stop-if-true
    n837 = Wait (ms)(milliseconds to wait=u32 200) -> ()  [unwired: 1 out]
    n838 = feedback-in #42("Load QCP") -> ()
    n839 = feedback #42() -> (w1435:bool)  [unwired: 1 in]
    n840 = Greater?(x="Load QCP", y=w1435) -> (0:w1434:bool)
    n841 = First Call?() -> (First Call?: T/F=w1431:bool)
    n842 = Or(x=w1434, y=w1431) -> (x .or. y?=w1432:bool)
    n843 = call <vilib>:"WPI_UtilitiesFRC ReadUserButton.vi"() -> ("User Button"=w1428:bool)  [unwired: 10 in, 1 out]
    n844 = shared-variable ".\\ControlMode.lvlib\\Tuning Mode?"("Tuning Mode?") -> ()  [unwired: 1 in, 1 out]
    n845 = feedback #43() -> (w1429:bool)  [unwired: 1 in]
    n846 = feedback-in #43(w1428) -> ()
    n847 = Greater?(x=w1428, y=w1429) -> (0:w1427:bool)
    n848 = Or(x=w1432, y=w1427) -> (x .or. y?=w1430:bool)
    n849 = case shown="True" w1430 {
      frame False {
      }
      frame True {
        n850 = call "QCP_Load.vi"() -> ()  [unwired: 12 in]
      }
    }
  }
  n851 = node-c288(i64 60 ("Period")) -> (w107:T30)  [unwired: 3 in]
  n852 = timed-loop {
    timing: w104 -> [_]
    timing-out: [_] -> w103
    tunnel: w97 -> [w1445]
    tunnel: w101 -> [w1444]
    stop <- _ stop-if-true
    # "Climb"
    n853 = node-c288() -> (→"Climb Loop Late?":bool, →"Climb Loop Duration":i64)  [unwired: 1 in]
    n854 = case shown="True" TRUE {
      tunnel: w1445 -> [w1456 w1490]
      tunnel: w1444 -> [w1453 w1487]
      tunnel: "Climb Blocking?" -> [_ w1486]
      frame False {
        # "enable climb"
        n855 = Wait on Notification(notifier=w1456, timeout in ms (-1)=0) -> (notification=w1454:T16, timed out?=w1455:bool)  [unwired: 2 in, 2 out]
        n856 = feedback #44() -> (w1448:dbl)  [unwired: 1 in]
        n857 = feedback #45() -> (w1449:bool)  [unwired: 1 in]
        n858 = case shown="False" w1455 {
          tunnel: w1454 -> [_ w1482]
          tunnel: [w1462 w1478] -> w1447
          tunnel: [w1461 w1480] -> w1450
          tunnel: w1449 -> [w1461 _]
          tunnel: w1448 -> [_ w1477]
          frame False {
            # "initally climb the rope at full speed, when we detect that the robot\nis swinging up, slow down, once the robot has fully swung, begin\nclimbin at full speed again"
            n859 = shared-variable ".\\Sensors.lvlib\\Body IMU Pitch"() -> (w1475:dbl)  [unwired: 1 in, 1 out]
            n860 = shared-variable ".\\Sensors.lvlib\\Body IMU Roll"() -> (w1476:dbl)  [unwired: 1 in, 1 out]
            n861 = Select(t=w1476, s="Pitch Roll Switch", f=w1475) -> (s? t:f=w1469:dbl)
            n862 = Greater?(x=w1469, y="Fast Thresh") -> (0:w1466:bool)
            n863 = Greater?(x=w1469, y="Slow Thresh") -> (0:w1465:bool)
            n864 = call <userlib>:"Stable.vi"("Eval Period (sec)"="Eval Period (s)", "Signal Input"=w1465) -> ("Stable"=w1464:bool)  [unwired: 9 in]
            n865 = call <userlib>:"Stable.vi"("Eval Period (sec)"="Eval Period (s)", "Signal Input"=w1466) -> ("Stable"=w1463:bool)  [unwired: 9 in]
            n866 = call <userlib>:"JK_Latch.vi"("Reset"=w1463, "Set"=w1464) -> ("Q"=w1473:bool)  [unwired: 5 in]
            n867 = Select(t="Slow Speed", s=w1473, f=1.0) -> (s? t:f=w1460:dbl)
            n868 = Select(t=w1460, s=w1461, f=0.0) -> (s? t:f=w1462:dbl)
          }
          frame True {
            # "only enable climb if the \ndriver sends the notification\notherwise disable it and\nstop the climb motor"
            n869 = Equal?(x=w1482, y=Drive_Commands."Align Rope") -> (x = y?=w1480:bool)
            n870 = Select(t=w1477, s=w1480, f=0.0) -> (s? t:f=w1478:dbl)
          }
        }
        "Climb Speed" <- w1447
        n871 = feedback-in #44(w1447) -> ()
        n872 = feedback-in #45(w1450) -> ()
        n873 = feedback-in #46(w1447) -> ()
        n874 = feedback #46() -> (w1452:dbl)  [unwired: 1 in]
        n875 = Not Equal?(x=w1452, y=w1447) -> (x != y?=w1451:bool)
        n876 = case shown="True" w1451 {
          tunnel: w1453 -> [_ w1458]
          tunnel: w1447 -> [_ w1457]
          frame False {
          }
          frame True {
            n877 = call <vilib>:"WPI_MotorControlSetOutput.vi"("Output"=w1457, "MotorControlDevRef"=w1458) -> ()  [unwired: 7 in, 3 out]
          }
        }
      }
      frame True {
        n878 = Select(t=-1, s=w1486, f=0) -> (s? t:f=w1483:i32)
        n879 = Wait on Notification(notifier=w1490, timeout in ms (-1)=w1483) -> (notification=w1488:T16, timed out?=w1489:bool)  [unwired: 2 in, 2 out]
        n880 = case shown="False" w1489 {
          tunnel: w1488 -> [w1493 _]
          tunnel: w1487 -> [w1492 _]
          frame False {
            n881 = case shown="\"Align Rope\"" w1493 {
              tunnel: [0.0 ("Max Speed") 0.0 ("Max Speed") 0.0 ("Max Speed") "Manual Speed"] -> w1491
              frame "Manual", Default {
              }
              frame "Get Gear" {
              }
              frame "Score Gear" {
              }
              frame "Align Rope" {
              }
            }
            n882 = call <vilib>:"WPI_MotorControlSetOutput.vi"("Output"=w1491, "MotorControlDevRef"=w1492) -> ()  [unwired: 7 in, 3 out]
          }
          frame True {
          }
        }
      }
    }
    n883 = node-c288("Climb  Loop Period") -> ()  [unwired: 1 out]
  }
  n884 = timed-loop {
    timing: w107 -> [_]
    timing-out: [_] -> w106
    tunnel: w97 -> [w1507]
    stop <- _ stop-if-true
    # "Gear Recieve Manual Mode"
    n885 = node-c288() -> (→"Gear Manual Late?":bool, →"Gear Manual Duration":i64)  [unwired: 1 in]
    n886 = shared-variable ".\\ControlMode.lvlib\\Manual Mode?"() -> (w1508:bool)  [unwired: 1 in, 1 out]
    n887 = case shown="True" w1508 {
      tunnel: w1507 -> [w1512 w1521]
      frame True {
        n888 = Wait on Notification(notifier=w1512, timeout in ms (-1)=0) -> (notification=w1509:T16, timed out?=w1510:bool)  [unwired: 2 in, 2 out]
        n889 = case shown="False" w1510 {
          tunnel: w1509 -> [w1514 _]
          frame False {
            n890 = Equal?(x=w1514, y=Drive_Commands."Get Gear") -> (x = y?=w1516:bool)
            n891 = Select(t=Pneumatics_Command."Toggle" ("Solenoid Command"), s=w1516, f=Pneumatics_Command."Nothing" ("Solenoid Command")) -> ()  [unwired: 1 out]
          }
          frame True {
          }
        }
      }
      frame False {
        n892 = Wait on Notification(notifier=w1521, timeout in ms (-1)=0) -> (notification=w1518:T16, timed out?=w1519:bool)  [unwired: 2 in, 2 out]
        n893 = case shown="False" w1519 {
          tunnel: w1518 -> [w1524 _]
          frame False {
            n894 = Equal?(x=w1524, y=Drive_Commands."Get Gear") -> (x = y?=w1526:bool)
            n895 = Select(t=Pneumatics_Command."Toggle" ("Solenoid Command"), s=w1526, f=Pneumatics_Command."Nothing" ("Solenoid Command")) -> (s? t:f=w1522:T35)
            n896 = call-poly <userlib>:"Pneumatics_Command_Set.vi"("Solenoid Command"=w1522) -> ()  [unwired: 10 in, 1 out]
          }
          frame True {
          }
        }
      }
    }
    n897 = node-c288("Gear  Manual Period") -> ()  [unwired: 1 out]
  }
  n898 = while {
    tunnel: [w1546] -> w71
    tunnel: "Log to USB?" -> [w1535]
    tunnel: "TDMS Name" -> [w1534]
    i -> [w1550]
    stop <- w1547 continue-if-true
    n899 = Current VI's Path() -> (path=w1545:path)
    n900 = Strip Path(path=w1545) -> (stripped path=w1539:path)  [unwired: 1 out]
    n901 = String To Path(string="~/") -> (path=w1543:path)
    n902 = Select(t=w1543, s=w1535, f=w1539) -> (s? t:f=w1544:path)
    n903 = Get Date/Time In Seconds() -> (seconds since 1Jan1904=w1552:timestamp)
    n904 = case shown="True" w1535 {
      selector: w1535 -> [w1558 _]
      tunnel: w1544 -> [w1557 w1563]
      tunnel: [w1557 w1560] -> w1541
      tunnel: [w1558 w1559] -> w1538
      frame False {
      }
      frame True {
        n905 = Build Path(base path=w1563, name or relative path="LogFiles") -> (appended path=w1562:path)
        n906 = call <vilib>:"Check if File or Folder Exists.vi"("path"=w1562) -> ("file or folder exists?"=w1566:bool, "dup path"=w1565:path)  [unwired: 8 in, 1 out]
        n907 = case shown="False" w1566 {
          tunnel: [w1568 w1569] -> w1561
          tunnel: w1565 -> [w1567 w1569]
          frame False {
            n908 = Create Folder(path (use dialog)=w1567) -> (created path=w1568:path)  [unwired: 2 in, 2 out]
          }
          frame True {
          }
        }
        n909 = call <vilib>:"Check if File or Folder Exists.vi"("path"=w1561) -> ("file or folder exists?"=w1559:bool, "dup path"=w1560:path)  [unwired: 8 in, 1 out]
      }
    }
    n910 = Format Date/Time String(time format string (%c)="%m-%#d-%Y %H%M", seconds (now)=w1552, UTC format=FALSE) -> (date/time string=w1555:string)
    n911 = Number To Hexadecimal String(1:i16 4 ("width (-)"), 2:w1550) -> (0:w1548:string)
    n912 = Concatenate Strings(w1534, w1555, w1548, ".tdms" ("string")) -> (w1556:string)
    n913 = Wait (ms)(milliseconds to wait=u32 1 ("millisecond multiple")) -> ()  [unwired: 1 out]
    n914 = case shown="False" w1538 {
      tunnel: w1539 -> [w1574 w1579]
      tunnel: [w1570 w1579] -> w1537
      frame False {
        n915 = Build Path(base path=w1574, name or relative path="LogFiles") -> (appended path=w1571:path)
        n916 = call <vilib>:"Check if File or Folder Exists.vi"("path"=w1571) -> ("file or folder exists?"=w1572:bool, "dup path"=w1573:path)  [unwired: 8 in, 1 out]
        n917 = case shown="False" w1572 {
          tunnel: [w1577 w1578] -> w1570
          tunnel: w1573 -> [w1576 w1578]
          frame False {
            n918 = Create Folder(path (use dialog)=w1576) -> (created path=w1577:path)  [unwired: 2 in, 2 out]
          }
          frame True {
          }
        }
      }
      frame True {
      }
    }
    n919 = Select(t=w1541, s=w1538, f=w1537) -> (s? t:f=w1540:path)
    n920 = Build Path(base path=w1540, name or relative path=w1556) -> (appended path=w1546:path)
    n921 = call <vilib>:"Check if File or Folder Exists.vi"("path"=w1546) -> ("file or folder exists?"=w1547:bool)  [unwired: 8 in, 2 out]
  }
  n922 = call <vilib>:"WPI_MotorControlRefNum Registry Get.vi"("refnum name"="Turret") -> ("MotorControlDevRef"=w30:T21)  [unwired: 9 in, 1 out]
  n923 = timed-loop {
    timing: w40 -> [_]
    timing-out: [_] -> w39
    shift-right: [w1643] -> _
    shift-left: TurretStates."Search" -> [w1640]
    tunnel: w36 -> [w1673]
    tunnel: -90.0 -> [w1659]
    tunnel: w34 -> [w1657]
    border: 0.0 -> [_]
    tunnel: w32 -> [w1618]
    tunnel: w30 -> [w1615]
    stop <- FALSE stop-if-true
    w1592 = 45.0 ("y")
    w1666 = 0
    # "Turret Control"
    n924 = node-c288() -> (→"TurretLate?":bool, →"Turret Duration":i64)  [unwired: 1 in]
    n925 = shared-variable ".\\Sensors.lvlib\\Turret IMU Yaw Wind"() -> (w1683:dbl)  [unwired: 1 in, 1 out]
    n926 = shared-variable ".\\Sensors.lvlib\\Body IMU Yaw"() -> (w1682:dbl)  [unwired: 1 in, 1 out]
    n927 = Wait on Occurrence(1:FALSE ("ignore previous (T)"), 2:w1657, 3:0 ("ms timeout (-1)")) -> (0:w1655:bool)
    n928 = Not(x=w1655) -> (.not. x?=w1586:bool)
    n929 = shared-variable ".\\Vision Variables.lvlib\\TargetLock"() -> (→"Auto Target Lock":bool)  [unwired: 1 in, 1 out]
    n930 = Subtract(x=w1682, y=w1683) -> (x-y=w1658:dbl)
    n931 = Add(x=w1658, y=w1659) -> (x+y=w1646:dbl)
    n932 = Negate(x=w1646) -> (-x=w1648:dbl)
    n933 = feedback #47() -> (w1647:dbl)
    n934 = Select(t=w1648, s=w1586, f=w1647) -> (s? t:f=w1645:dbl)
    n935 = feedback-in #47(w1645) -> ()
    n936 = Add(x=w1645, y=w1646) -> (x+y=w1626:dbl)
    n937 = feedback #48() -> (w1675:u32)  [unwired: 1 in]
    n938 = Bundle("Search Gains"="Search Gains", "Search Range"="Search Range") -> (w1605:T47)  [unwired: 1 in]
    n939 = Bundle("Jump to Desired Angle"="Jump to Desired Angle", "Jump Output"="Jump Output") -> (w1604:T48)  [unwired: 1 in]
    n940 = Bundle("Target Range Gains"="Target Range Gains", "Target range"="Target range") -> (w1603:T49)  [unwired: 1 in]
    n941 = Build Array(w1605, w1604, w1603) -> (w1602:T50)
    n942 = feedback #49() -> (w1679:dbl)  [unwired: 1 in]
    n943 = case shown="\"Search\"" w1640 {
      selector: w1640 -> [w1749 w1802 w1823 _]
      tunnel: w1626 -> [w1745 w1799 _ _]
      tunnel: [w1729 w1776 w1825 TurretStates."Target Valid in Range"] -> w1624
      tunnel: [w1733 w1796 w1822 w1827] -> w1639
      tunnel: w1679 -> [_ w1778 _ _]
      tunnel: [w1732 w1778 0.0 ("Double") 0.0 ("Double")] -> w1674
      tunnel: [w1743 w1770 u32 0 ("millisecond timer value") u32 0 ("millisecond timer value")] -> w1676
      tunnel: w1675 -> [w1742 w1770 _ _]
      tunnel: [w1725 w1762 w1809 w1831] -> w1616
      tunnel: w1602 -> [w1724 w1764 w1810 w1832]
      frame "Target Valid in Range", Default {
        # "Part of Guess F"
        n944 = shared-variable ".\\Vision Variables.lvlib\\Boiler Yaw delta"() -> (w1753:dbl)  [unwired: 1 in, 1 out]
        n945 = shared-variable ".\\Base Parameters.lvlib\\TurretCCWBound"() -> (w1728:dbl)  [unwired: 1 in, 1 out]
        n946 = shared-variable ".\\Base Parameters.lvlib\\TurretCWBound"() -> (w1727:dbl)  [unwired: 1 in, 1 out]
        n947 = shared-variable ".\\Vision Variables.lvlib\\Boiler Found"() -> (w1750:bool)  [unwired: 1 in, 1 out]
        n948 = Tick Count (ms)() -> (millisecond timer value=w1743:u32)
        n949 = disable-structure shown="Disabled" {
          disable-tunnel: [w1756 _] -> w1744
          frame Disabled {
            n950 = Greater?(x=0.0, y="Min Rate") -> (0:w1756:bool)
          }
          frame Enabled {
          }
        }
        n951 = Subtract(x=w1743, y=w1742) -> (x-y=w1741:u32)
        n952 = Add(x=w1745, y=w1753) -> (x+y=w1752:dbl)
        n953 = feedback-in #50(w1753) -> ()
        n954 = feedback #50() -> (w1754:dbl)  [unwired: 1 in]
        n955 = Equal?(x=w1753, y=w1754) -> (x = y?=w1736:bool)
        n956 = Less?(x=w1741, y=u32 50) -> (x < y?=w1739:bool)
        n957 = Not(x=w1750) -> (.not. x?=w1731:bool)
        n958 = feedback #51() -> (w1751:dbl)  [unwired: 1 in]
        n959 = Or(x=w1731, y=w1736) -> (x .or. y?=w1735:bool)
        n960 = Select(t=w1751, s=w1735, f=w1752) -> (s? t:f=w1733:dbl)
        n961 = feedback-in #51(w1733) -> ()
        n962 = Greater?(x=w1733, y=w1727) -> (0:w1747:bool)
        n963 = Less?(x=w1733, y=w1728) -> (x < y?=w1746:bool)
        n964 = Compound Arithmetic op=OR(w1731, w1747, w1746, w1744) -> (w1738:bool)
        n965 = shared-variable ".\\Teleop_QCP.lvlib\\Turret_Valid_Lost_Time"() -> (w1723:dbl)  [unwired: 1 in, 1 out]
        n966 = And(x=w1739, y=w1738) -> (x .and. y?=w1737:bool)
        n967 = shared-variable ".\\Sensors.lvlib\\Body IMU Yaw"() -> (w1734:dbl)  [unwired: 1 in, 1 out]
        n968 = call <userlib>:"De-Bounce_or_Delay.vi"("Eval Period (sec)"=w1723, "Signal Input"=w1737) -> ("Stable"=w1730:bool)  [unwired: 9 in]
        n969 = Index Array(array=w1724, index=2) -> (element=w1725:T49)
        n970 = Add(x=w1734, y=w1733) -> (x+y=w1732:dbl)
        n971 = Select(t=TurretStates."Search", s=w1730, f=w1749) -> (s? t:f=w1729:T11)
      }
      frame "Guess" {
        w1794 = T51 1 items=["none", "-180 to 180 (-pi to pi)", "0 to 360 (0 to 2pi)"] ("angle range")
        w1795 = T52 2 items=["radian in, radian out", "radian in, degree out", "degree in, degree out", "degree in, radian out"] ("angle units")
        n972 = shared-variable ".\\Teleop_QCP.lvlib\\Turret_Guess_State_Time"() -> (w1760:dbl)  [unwired: 1 in, 1 out]
        n973 = shared-variable ".\\Base Parameters.lvlib\\TurretCCWBound"() -> (w1767:dbl)  [unwired: 1 in, 1 out]
        n974 = shared-variable ".\\Base Parameters.lvlib\\TurretCWBound"() -> (w1766:dbl)  [unwired: 1 in, 1 out]
        n975 = shared-variable ".\\Teleop_QCP.lvlib\\Turret_Guess_Switch_Outer_Delta"() -> (w1759:dbl)  [unwired: 1 in, 1 out]
        n976 = shared-variable ".\\Sensors.lvlib\\Body IMU Yaw"() -> (w1789:dbl)  [unwired: 1 in, 1 out]
        n977 = shared-variable ".\\Teleop_QCP.lvlib\\Turret_Guess_Stable_Movement"() -> (w1761:dbl)  [unwired: 1 in, 1 out]
        n978 = Tick Count (ms)() -> (millisecond timer value=w1771:u32)
        n979 = Subtract(x=w1771, y=w1770) -> (x-y=w1769:u32)
        n980 = Greater?(x=w1769, y=w1760) -> (0:w1768:bool)
        n981 = feedback-in #52(w1789) -> ()
        n982 = feedback #52() -> (w1790:dbl)  [unwired: 1 in]
        n983 = Subtract(x=w1789, y=w1790) -> (x-y=w1783:dbl)
        n984 = Subtract(x=w1767, y=w1759) -> (x-y=w1801:dbl)
        n985 = Add(x=w1766, y=w1759) -> (x+y=w1800:dbl)
        n986 = Subtract(x=w1789, y=w1778) -> (x-y=w1793:dbl)
        n987 = call-poly <vilib>:"Wrap Angle.vi"("angle units"=w1795, "angle range"=w1794, "angle in"=w1793) -> ("angle out"=w1792:dbl)  [unwired: 7 in, 1 out]
        n988 = Less Than 0?(x=w1783) -> (x < 0?=w1786:bool)
        n989 = Less?(x=w1792, y=w1801) -> (x < y?=w1787:bool)
        n990 = Greater?(x=w1792, y=w1800) -> (0:w1791:bool)
        n991 = Greater Than 0?(x=w1783) -> (x > 0?=w1788:bool)
        n992 = shared-variable ".\\Sensors.lvlib\\TurretInTolerance"() -> (w1765:bool)  [unwired: 1 in, 1 out]
        n993 = And(x=w1791, y=w1788) -> (x .and. y?=w1780:bool)
        n994 = shared-variable ".\\Vision Variables.lvlib\\Boiler Found"() -> (w1775:bool)  [unwired: 1 in, 1 out]
        n995 = And(x=w1787, y=w1786) -> (x .and. y?=w1782:bool)
        n996 = shared-variable ".\\Teleop_QCP.lvlib\\Turret_Guess_Valid_Time"() -> (w1758:dbl)  [unwired: 1 in, 1 out]
        n997 = In Range and Coerce(upper limit=w1766, x=w1792, lower limit=w1767) -> (In Range?=w1772:bool)  [unwired: 1 out]
        n998 = call <userlib>:"Stable.vi"("Eval Period (sec)"=w1761, "Signal Input"=w1780) -> ("Stable"=w1779:bool)  [unwired: 9 in]
        n999 = call <userlib>:"Stable.vi"("Eval Period (sec)"=w1761, "Signal Input"=w1782) -> ("Stable"=w1781:bool)  [unwired: 9 in]
        n1000 = call <userlib>:"JK_Latch.vi"("Reset"=w1765, "Set"=w1779) -> ("Q"=w1785:bool)  [unwired: 5 in]
        n1001 = call <userlib>:"JK_Latch.vi"("Reset"=w1765, "Set"=w1781) -> ("Q"=w1784:bool)  [unwired: 5 in]
        n1002 = call <userlib>:"Stable.vi"("Eval Period (sec)"=w1758, "Signal Input"=w1775) -> ("Stable"=w1774:bool)  [unwired: 9 in]
        n1003 = Select(t=w1767, s=w1785, f=w1799) -> (s? t:f=w1798:dbl)
        n1004 = Select(t=TurretStates."Search", s=w1768, f=w1802) -> (s? t:f=w1777:T11)
        n1005 = Select(t=w1766, s=w1784, f=w1798) -> (s? t:f=w1797:dbl)
        n1006 = Index Array(array=w1764, index=1) -> (element=w1762:T49)
        n1007 = And(x=w1774, y=w1772) -> (x .and. y?=w1773:bool)
        n1008 = Select(t=TurretStates."Target Valid in Range", s=w1773, f=w1777) -> (s? t:f=w1776:T11)
        n1009 = Select(t=w1792, s=w1772, f=w1797) -> (s? t:f=w1796:dbl)
      }
      frame "Search" {
        n1010 = shared-variable ".\\Teleop_QCP.lvlib\\Turret_Search_Softstop"() -> (w1808:dbl)  [unwired: 1 in, 1 out]
        n1011 = shared-variable ".\\Teleop_QCP.lvlib\\Turret_Valid_Wait_In_Search"() -> (w1807:dbl)  [unwired: 1 in, 1 out]
        n1012 = shared-variable ".\\Vision Variables.lvlib\\Boiler Found"() -> (w1818:bool)  [unwired: 1 in, 1 out]
        n1013 = shared-variable ".\\Base Parameters.lvlib\\TurretCWBound"() -> (w1812:dbl)  [unwired: 1 in, 1 out]
        n1014 = shared-variable ".\\Base Parameters.lvlib\\TurretCCWBound"() -> (w1813:dbl)  [unwired: 1 in, 1 out]
        n1015 = call <userlib>:"Stable.vi"("Eval Period (sec)"=0.2, "Signal Input"=w1818) -> ("Stable"=w1817:bool)  [unwired: 9 in]
        n1016 = Subtract(x=w1812, y=w1808) -> (x-y=w1805:dbl)
        n1017 = Add(x=w1813, y=w1808) -> (x+y=w1806:dbl)
        n1018 = shared-variable ".\\Sensors.lvlib\\TurretInTolerance"() -> (w1811:bool)  [unwired: 1 in, 1 out]
        n1019 = Select(t=TurretStates."Target Valid in Range", s=w1817, f=w1823) -> (s? t:f=w1825:T11)
        n1020 = call <userlib>:"Stable.vi"("Eval Period (sec)"=w1807, "Signal Input"=w1811) -> ("Stable"=w1814:bool)  [unwired: 9 in]
        n1021 = call <userlib>:"Latch.vi"("Edge"=TRUE ("Edge:  When lit the output is \"True\" for this control"), "In"=w1814) -> ("Out"=w1819:bool)
        n1022 = Select(t=w1806, s=w1819, f=w1805) -> (s? t:f=w1822:dbl)
        n1023 = Index Array(array=w1810) -> (element=w1809:T49)  [unwired: 1 in]
      }
      frame "Desired Angle Shot" {
        n1024 = shared-variable ".\\Teleop_QCP.lvlib\\Turret_Desired"() -> (w1826:dbl)  [unwired: 1 in, 1 out]
        n1025 = shared-variable ".\\Vision Variables.lvlib\\TurretDesiredAngle"() -> (w1828:dbl)  [unwired: 1 in, 1 out]
        n1026 = Index Array(array=w1832, index=1) -> (element=w1831:T49)
        n1027 = Select(t=w1826, s="Manual Entry", f=w1828) -> (s? t:f=w1827:dbl)
      }
    }
    "Turret State" <- w1624
    n1028 = feedback-in #48(w1676) -> ()
    n1029 = feedback-in #49(w1674) -> ()
    n1030 = shared-variable ".\\ControlMode.lvlib\\ShootingMode"() -> (w1633:bool)  [unwired: 1 in, 1 out]
    n1031 = shared-variable ".\\Vision Variables.lvlib\\Boiler Found"() -> (w1600:bool)  [unwired: 1 in, 1 out]
    n1032 = shared-variable ".\\OperatorController.lvlib\\Turret Speed"() -> (w1634:dbl)  [unwired: 1 in, 1 out]
    n1033 = shared-variable ".\\Vision Variables.lvlib\\Boiler distance"() -> (w1635:dbl)  [unwired: 1 in, 1 out]
    n1034 = Not(x=w1600) -> (.not. x?=w1601:bool)
    n1035 = shared-variable ".\\Teleop_QCP.lvlib\\Turret_Search_Tol"() -> (w1582:dbl)  [unwired: 1 in, 1 out]
    n1036 = feedback #53() -> (w1632:bool)  [unwired: 1 in]
    n1037 = feedback-in #53(w1633) -> ()
    n1038 = Less?(x=w1633, y=w1632) -> (x < y?=w1599:bool)
    n1039 = shared-variable ".\\Teleop_QCP.lvlib\\Turret_Valid_Setpoint_Tol"() -> (w1581:dbl)  [unwired: 1 in, 1 out]
    n1040 = Or(x=w1599, y=w1601) -> (x .or. y?=w1598:bool)
    n1041 = Negate(x=w1634) -> (-x=w1597:dbl)
    n1042 = call "Bump Turret Az.vi"("reset"=w1598, "D"=w1635, "d"="d", "D-Pad"=w1597) -> ("offset"=w1637:dbl)  [unwired: 7 in]
    n1043 = shared-variable ".\\Teleop_QCP.lvlib\\Turret_Range_For_I"() -> (w1583:dbl)  [unwired: 1 in, 1 out]
    n1044 = shared-variable ".\\ToLog.lvlib\\TurretBump"(w1637) -> ()  [unwired: 1 in, 1 out]
    n1045 = Add(x=w1637, y=w1639) -> (x+y=w1638:dbl)
    n1046 = Bundle(w1626, w1638) -> (→"Turret":cluster{dbl, dbl})  [unwired: 1 in]
    n1047 = Subtract(x=w1638, y=w1626) -> (x-y=w1680:dbl)
    n1048 = Equal?(x=w1624, y=TurretStates."Search") -> (x = y?=w1628:bool)
    n1049 = Select(t=w1582, s=w1628, f=w1581) -> (s? t:f=w1630:dbl)
    n1050 = Equal?(x=TurretStates."Target Valid in Range", y=w1624) -> (x = y?=w1663:bool)
    n1051 = Absolute Value(x=w1680) -> (abs(x)=w1650:dbl)
    n1052 = Greater?(x=w1650, y=w1583) -> (0:w1641:bool)
    n1053 = Less?(x=w1650, y=w1630) -> (x < y?=w1631:bool)
    n1054 = And(x=w1663, y=w1631) -> (x .and. y?=w1662:bool)
    n1055 = shared-variable ".\\Sensors.lvlib\\Body IMU Roll"() -> (w1590:dbl)  [unwired: 1 in, 1 out]
    n1056 = Wait on Notification(notifier=w1618, timeout in ms (-1)=0) -> (notification=w1621:T16, timed out?=w1622:bool)  [unwired: 2 in, 2 out]
    n1057 = shared-variable ".\\Sensors.lvlib\\DeltaSetpointProcessTurret"(w1650) -> ()  [unwired: 1 in, 1 out]
    n1058 = Compound Arithmetic op=OR(w1631, "Reinitalize?", w1641) -> (w1627:bool)
    n1059 = shared-variable ".\\Sensors.lvlib\\TurretInTolerance"(w1631) -> ()  [unwired: 1 in, 1 out]
    n1060 = call "Square Waves Generator.vi"("Duty Cycle (%)"="Duty Cycle (%)", "Period (ms)"="Period (ms)", "Enable"=TRUE) -> ("Signal"=w1668:bool)
    n1061 = Or(x="Test LEDS", y=w1662) -> (x .or. y?=w1661:bool)
    n1062 = shared-variable ".\\Vision Variables.lvlib\\Boiler Target Lock"(w1661) -> ()  [unwired: 1 in, 1 out]
    n1063 = shared-variable ".\\Teleop_QCP.lvlib\\Turret_Feed_CCW"() -> (w1585:dbl)  [unwired: 1 in, 1 out]
    n1064 = shared-variable ".\\OperatorController.lvlib\\Manual Turret?"() -> (w1625:bool)  [unwired: 1 in, 1 out]
    n1065 = feedback #54() -> (w1619:bool)  [unwired: 1 in]
    n1066 = case shown="True" w1622 {
      tunnel: w1621 -> [w1687 _]
      tunnel: Drive_Commands."Align Rope" ("notification") -> [w1686 _]
      tunnel: [w1685 w1688] -> w1596
      tunnel: w1619 -> [_ w1688]
      frame False {
        n1067 = Equal?(x=w1686, y=w1687) -> (x = y?=w1685:bool)
      }
      frame True {
      }
    }
    n1068 = feedback-in #54(w1596) -> ()
    n1069 = shared-variable ".\\Sensors.lvlib\\Body IMU Pitch"() -> (w1591:dbl)  [unwired: 1 in, 1 out]
    n1070 = shared-variable ".\\OperatorController.lvlib\\Turret Speed"() -> (w1651:dbl)  [unwired: 1 in, 1 out]
    n1071 = shared-variable ".\\Teleop_QCP.lvlib\\Turret_Max_Speed"() -> (w1580:dbl)  [unwired: 1 in, 1 out]
    n1072 = Absolute Value(x=w1590) -> (abs(x)=w1587:dbl)
    n1073 = Absolute Value(x=w1591) -> (abs(x)=w1588:dbl)
    n1074 = Greater?(x=w1588, y=w1592) -> (0:w1594:bool)
    n1075 = Greater?(x=w1587, y=w1592) -> (0:w1593:bool)
    n1076 = feedback #55(w1666) -> (w1665:i32)
    n1077 = shared-variable ".\\Vision Variables.lvlib\\TargetTracking"() -> (w1614:bool)  [unwired: 1 in, 1 out]
    n1078 = Or(x=w1594, y=w1593) -> (x .or. y?=w1595:bool)
    n1079 = Or(x=w1595, y=w1596) -> (x .or. y?=w1589:bool)
    n1080 = Multiply(x=w1651, y=w1580) -> (x*y=w1617:dbl)
    n1081 = feedback #56(w1666) -> (w1667:i32)
    n1082 = case shown="2" w1667 {
      selector: w1667 -> [w1690 w1698 w1713]
      tunnel: w1673 -> [_ w1705 w1720]
      tunnel: [w1692 w1694 w1709] -> w1672
      tunnel: w1668 -> [_ w1702 w1717]
      tunnel: w1665 -> [_ w1700 w1715]
      tunnel: w1661 -> [w1689 w1697 w1712]
      frame 0, Default {
        n1083 = Increment(x=w1690) -> (x+1=w1691:i32)
        n1084 = Select(t=w1691, s=w1689, f=w1690) -> (s? t:f=w1692:i32)
      }
      frame 1 {
        w1695 = 0
        n1085 = Not Equal?(x=w1700, y=w1698) -> (x != y?=w1699:bool)
        n1086 = Increment(x=w1698) -> (x+1=w1701:i32)
        n1087 = Not(x=w1697) -> (.not. x?=w1693:bool)
        n1088 = Build Array(T40."gear" ("Enum"), w1695, w1695, w1695) -> (w1703:i32[])
        n1089 = Select(t=w1701, s=w1702, f=w1698) -> (s? t:f=w1696:i32)
        n1090 = case shown="True" w1699 {
          tunnel: w1705 -> [_ w1707]
          tunnel: w1703 -> [_ w1706]
          frame False {
          }
          frame True {
            n1091 = Send Notification(notification=w1706, notifier=w1707) -> ()  [unwired: 1 in, 2 out]
          }
        }
        n1092 = Select(t=w1695, s=w1693, f=w1696) -> (s? t:f=w1694:i32)
      }
      frame 2 {
        w1710 = 0
        n1093 = Not Equal?(x=w1715, y=w1713) -> (x != y?=w1714:bool)
        n1094 = Decrement(x=w1713) -> (x-1=w1716:i32)
        n1095 = Not(x=w1712) -> (.not. x?=w1708:bool)
        n1096 = Build Array(T40."ball" ("Enum"), w1710, w1710, w1710) -> (w1718:i32[])
        n1097 = Select(t=w1716, s=w1717, f=w1713) -> (s? t:f=w1711:i32)
        n1098 = case shown="True" w1714 {
          tunnel: w1720 -> [_ w1722]
          tunnel: w1718 -> [_ w1721]
          frame False {
          }
          frame True {
            n1099 = Send Notification(notification=w1721, notifier=w1722) -> ()  [unwired: 1 in, 2 out]
          }
        }
        n1100 = Select(t=w1710, s=w1708, f=w1711) -> (s? t:f=w1709:i32)
      }
    }
    n1101 = feedback-in #55(w1667) -> ()
    n1102 = feedback-in #56(w1672) -> ()
    n1103 = shared-variable ".\\Teleop_QCP.lvlib\\Turret_Feed_CW"() -> (w1584:dbl)  [unwired: 1 in, 1 out]
    n1104 = call "Turret-firstVI.vi"("MotorControlDevRef"=w1615, "Current angle"=w1626, "desired Angle"=w1638, "PID Values"=w1616, "Manual"=w1625, "Feed CCW"=w1585, "Output"=w1617, "Feed CW"=w1584, "reinitialize? (F)"=w1627, "Climbing?"=w1589) -> ("Motor Output"=→"Motor Output":dbl)  [unwired: 9 in]
    n1105 = Or(x=w1614, y="Target Track") -> (x .or. y?=w1613:bool)
    n1106 = Select(t=w1624, s=w1613, f=TurretStates."Desired Angle Shot" ("x")) -> (s? t:f=w1643:T11)
    n1107 = node-c288("Turret Period") -> ()  [unwired: 1 out]
  }
  n1108 = node-c288(w39) -> ()  [unwired: 1 out]
  n1109 = node-c288(w106) -> ()  [unwired: 1 out]
  n1110 = node-c288(w103) -> ()  [unwired: 1 out]
  n1111 = shared-variable ".\\Notifiers.lvlib\\Drive Loop Cluster"() -> (w15:T19)  [unwired: 1 in, 1 out]
  n1112 = disable-structure shown="Disabled" {
    disable-tunnel: [w1842 _] -> w10
    frame Disabled {
      n1113 = call <userlib>:"IMUOrientRefNum Registry Get.vi"("refnum name"="BU TurretPrime") -> ("I2CDevRef out"=w1842:T33)  [unwired: 9 in, 1 out]
    }
    frame Enabled {
    }
  }
  n1114 = disable-structure shown="Disabled" {
    disable-tunnel: [w1844 _] -> w11
    frame Disabled {
      n1115 = call <userlib>:"IMUOrientRefNum Registry Get.vi"("refnum name"="BU BodyPrime") -> ("I2CDevRef out"=w1844:T33)  [unwired: 9 in, 1 out]
    }
    frame Enabled {
    }
  }
  n1116 = disable-structure shown="Disabled" {
    disable-tunnel: [w1847 _] -> w18
    frame Disabled {
      n1117 = call <vilib>:"WPI_AnalogChannelRefNum Registry Get.vi"("refnum name"="Sonar") -> ("AIDeviceRef"=w1847:T44)  [unwired: 9 in, 1 out]
    }
    frame Enabled {
    }
  }
  n1118 = TDMS Open(6:TRUE ("disable buffering? (T)"), 7:enum16{"1.0", "2.0"}."2.0" ("file format version (2.0)"), 10:T14."open or create" ("operation (0:open)"), 11:w71) -> (3:w69:refnum<k34>)  [unwired: 3 in, 1 out]
  n1119 = Initialize Array(0.0, w80) -> (w76:dbl[])
  n1120 = To Unsigned Long Integer(number=w80) -> (unsigned 32bit integer=w79:u32)
  n1121 = call <userlib>:"IMUOrientRefNum Registry Get.vi"("refnum name"="TurretPrime") -> ("I2CDevRef out"=w19:T33)  [unwired: 9 in, 1 out]
  n1122 = call <vilib>:"WPI_EncoderRefNum Registry Get.vi"("refnum name"="RightDriveEncoder") -> ("EncoderDevRef"=w22:T53)  [unwired: 9 in, 1 out]
  n1123 = call <vilib>:"WPI_EncoderRefNum Registry Get.vi"("refnum name"="LeftDriveEncoder") -> ("EncoderDevRef"=w21:T53)  [unwired: 9 in, 1 out]
  n1124 = call <userlib>:"IMUOrientRefNum Registry Get.vi"("refnum name"="BodyPrime") -> ("I2CDevRef out"=w20:T33)  [unwired: 9 in, 1 out]
  n1125 = RT FIFO Create(0:"Drive FIFO" ("name (unnamed)"), 1:w76, 4:u32 100 ("size (10)"), 6:w79) -> (8:w77:refnum<k33>)  [unwired: 4 in, 2 out]
  n1126 = node-c288() -> (w24:T30)  [unwired: 4 in]
  n1127 = timed-loop {
    tunnel: w22 -> [w1917]
    tunnel: w21 -> [w1916]
    timing: w24 -> [_]
    timing-out: [_] -> w23
    tunnel: w18 -> [w1914]
    tunnel: w15 -> [w1911]
    shift-right: [w1896] -> _
    shift-left: w20 -> [w1897]
    shift-right: [w1895] -> _
    shift-left: w19 -> [w1898]
    shift-right: [w1891] -> _
    shift-left: Control_1."Pri Body IMU" -> [w1892]
    tunnel: w11 -> [w1884]
    shift-right: [w1872] -> _
    shift-left: _ -> [w1874]
    tunnel: "Orient Ref (Wind)" -> [w1873]
    shift-right: [w1868] -> _
    shift-left: TurretImu."Pri Turret IMU" -> [w1869]
    tunnel: "IMU Read Enable" -> [w1867]
    tunnel: w10 -> [w1866]
    tunnel: "IMU Read Enable" -> [w1865]
    tunnel: "Orient Ref (Wind)" -> [w1864]
    shift-right: [w1863] -> _
    shift-left: _ -> [w1862]
    stop <- FALSE stop-if-true
    # "Sesnor Loop"
    n1128 = node-c288() -> (→"Sensor Loop Late? 2":bool, →"Sensor Loop Duration? 2":i64)  [unwired: 1 in]
    n1129 = case shown="\"Pri Body IMU\", Default" w1892 {
      tunnel: w1897 -> [w1984 _]
      tunnel: [w1979 w2008] -> w1891
      tunnel: [w1978 w2004] -> w1890
      tunnel: [w1977 w2003] -> w1889
      tunnel: [w1976 w2002] -> w1888
      tunnel: [w1975 w2001] -> w1887
      tunnel: [w1971 w2007] -> w1871
      tunnel: [w1974 w2006] -> w1886
      tunnel: [w1973 w2005] -> w1885
      tunnel: w1884 -> [_ w2000]
      tunnel: [w1972 FALSE ("Status")] -> w1880
      tunnel: [w1970 w1998] -> w1875
      tunnel: w1874 -> [_ w1997]
      tunnel: w1873 -> [_ w1992]
      tunnel: [w1969 w1993] -> w1872
      tunnel: w1867 -> [w1968 w1990]
      tunnel: [w1966 w1988] -> w1858
      tunnel: [w1965 w1987] -> w1861
      tunnel: [w1964 w1986] -> w1859
      frame "Pri Body IMU", Default {
        (unwired) Control_1."Bu Body IMU"
        n1130 = First Call?() -> (First Call?: T/F=w1982:bool)
        n1131 = feedback #57() -> (w1983:bool)  [unwired: 1 in]
        n1132 = feedback-in #57(w1982) -> ()
        n1133 = call <userlib>:"IMUOrientRead.vi"("I2CDevRef"=w1984, "Orient Reset (Wind)"=w1983, "Read Enable"=w1968) -> ("Cal Status"=w1985:T58, "Orient Y/R/P"=w1969:T59, "Acc X,Y,Z"=w1967:cluster{"X Acc":dbl, "Y Acc":dbl, "Z Acc":dbl})  [unwired: 6 in, 4 out]
        n1134 = Unbundle By Name(w1969) -> ("Yaw Wind"=w1971:dbl, "Roll Wind"=w1974:dbl, "Pitch Wind"=w1973:dbl, "Yaw"=w1970:dbl)
        n1135 = Unbundle By Name(w1967) -> ("X Acc"=w1966:dbl, "Y Acc"=w1965:dbl, "Z Acc"=w1964:dbl)
        n1136 = Unbundle(w1985) -> ("Mag"=w1978:T60, "Acc"=w1977:T60, "Gyro"=w1976:T60, "Sys"=w1975:T60, "Status"=w1972:bool)
        "Good Pri 2" <- w1972
        n1137 = shared-variable ".\\ToLog.lvlib\\BodyPriGood"(w1972) -> ()  [unwired: 1 in, 1 out]
        n1138 = Select(t=Control_1."Pri Body IMU", s=w1972, f=Control_1."Pri Body IMU") -> (s? t:f=w1979:T10)
      }
      frame "Bu Body IMU" {
        n1139 = Unbundle By Name(w1997) -> ("Yaw Wind"=w1996:dbl, "Roll Wind"=w1995:dbl, "Pitch Wind"=w1994:dbl)
        n1140 = Bundle By Name(cluster=w1992, "Yaw Ref"=w1996, "Roll Ref"=w1995, "Pitch Ref"=w1994) -> (w1991:T7)
        n1141 = call <userlib>:"IMUOrientRead.vi"("I2CDevRef"=w2000, "Read Enable"=w1990, "Orient Ref (Wind)"=w1991) -> ("Cal Status"=w2012:T58, "Orient Y/R/P"=w1993:T59, "Acc X,Y,Z"=w1989:cluster{"X Acc":dbl, "Y Acc":dbl, "Z Acc":dbl})  [unwired: 6 in, 4 out]
        n1142 = Unbundle By Name(w1993) -> ("Yaw Wind"=w2007:dbl, "Roll Wind"=w2006:dbl, "Pitch Wind"=w2005:dbl, "Yaw"=w1998:dbl)
        n1143 = Unbundle(w2012) -> ("Mag"=w2004:T60, "Acc"=w2003:T60, "Gyro"=w2002:T60, "Sys"=w2001:T60, "Status"=w2011:bool)
        "Good BU 3" <- w2011
        n1144 = shared-variable ".\\ToLog.lvlib\\BodyBuGood"(w2011) -> ()  [unwired: 1 in, 1 out]
        n1145 = Unbundle By Name(w1989) -> ("X Acc"=w1988:dbl, "Y Acc"=w1987:dbl, "Z Acc"=w1986:dbl)
        n1146 = Select(t=Control_1."Bu Body IMU", s=w2011, f=Control_1."Bu Body IMU") -> (s? t:f=w2008:T10)
      }
    }
    "M 5" <- w1887
    "A 5" <- w1888
    "G 5" <- w1889
    "S 5" <- w1890
    "Yaw Body 2" <- w1871
    "Roll Body 2" <- w1886
    "Pitch Body 2" <- w1885
    "Accel X" <- w1858
    "Accel Z" <- w1859
    "Accel Y" <- w1861
    n1147 = case shown="\"Pri Turret IMU\", Default" w1869 {
      tunnel: [w1942 w1952] -> w1908
      tunnel: [w1941 w1953] -> w1907
      tunnel: [w1940 w1954] -> w1906
      tunnel: [w1939 w1955] -> w1905
      tunnel: w1898 -> [w1937 _]
      tunnel: [w1936 w1956] -> w1894
      tunnel: [w1935 w1950] -> w1893
      tunnel: [w1931 FALSE ("Status")] -> w1879
      tunnel: [w1932 w1957] -> w1876
      tunnel: [w1930 w1951] -> w1868
      tunnel: w1866 -> [_ w1949]
      tunnel: w1865 -> [w1929 w1947]
      tunnel: w1864 -> [_ w1948]
      tunnel: [w1928 w1946] -> w1863
      tunnel: w1862 -> [_ w1945]
      frame "Pri Turret IMU", Default {
        w1927 = TurretImu."Pri Turret IMU"
        n1148 = First Call?() -> (First Call?: T/F=w1934:bool)
        n1149 = feedback #58() -> (w1933:bool)  [unwired: 1 in]
        n1150 = feedback-in #58(w1934) -> ()
        n1151 = call <userlib>:"IMUOrientRead.vi"("I2CDevRef"=w1937, "Orient Reset (Wind)"=w1933, "Read Enable"=w1929) -> ("Cal Status"=w1938:T58, "Orient Y/R/P"=w1928:T59)  [unwired: 6 in, 5 out]
        n1152 = Unbundle By Name(w1928) -> ("Yaw Wind"=w1932:dbl, "Roll Wind"=w1936:dbl, "Pitch Wind"=w1935:dbl)
        n1153 = Unbundle(w1938) -> ("Mag"=w1939:T60, "Acc"=w1940:T60, "Gyro"=w1941:T60, "Sys"=w1942:T60, "Status"=w1931:bool)
        "Good Pri." <- w1931
        n1154 = shared-variable ".\\ToLog.lvlib\\TurretPriGood"(w1931) -> ()  [unwired: 1 in, 1 out]
        n1155 = Select(t=w1927, s=w1931, f=w1927) -> (s? t:f=w1930:T9)
      }
      frame "Bu Turret IMU" {
        w1944 = TurretImu."Bu Turret IMU"
        n1156 = Unbundle By Name(w1945) -> ("Yaw Wind"=w1962:dbl, "Roll Wind"=w1961:dbl, "Pitch Wind"=w1960:dbl)
        n1157 = Bundle By Name(cluster=w1948, "Yaw Ref"=w1962, "Roll Ref"=w1961, "Pitch Ref"=w1960) -> (w1959:T7)
        n1158 = call <userlib>:"IMUOrientRead.vi"("I2CDevRef"=w1949, "Read Enable"=w1947, "Orient Ref (Wind)"=w1959) -> ("Cal Status"=w1963:T58, "Orient Y/R/P"=w1946:T59)  [unwired: 6 in, 5 out]
        n1159 = Unbundle By Name(w1946) -> ("Yaw Wind"=w1957:dbl, "Roll Wind"=w1956:dbl, "Pitch Wind"=w1950:dbl)
        n1160 = Unbundle(w1963) -> ("Mag"=w1955:T60, "Acc"=w1954:T60, "Gyro"=w1953:T60, "Sys"=w1952:T60, "Status"=w1943:bool)
        "Good BU 2" <- w1943
        n1161 = shared-variable ".\\ToLog.lvlib\\TurretBuGood"(w1943) -> ()  [unwired: 1 in, 1 out]
        n1162 = Select(t=w1944, s=w1943, f=w1944) -> (s? t:f=w1951:T9)
      }
    }
    "Yaw Turret 2" <- w1876
    "M 8" <- w1908
    "A 8" <- w1907
    "G 8" <- w1906
    "S 8" <- w1905
    "Roll Turret 2" <- w1894
    "Pitch Turret 2" <- w1893
    n1163 = disable-structure shown="Disabled" {
      disable-tunnel: w1914 -> [w1926 _]
      frame Disabled {
        n1164 = call <vilib>:"WPI_AnalogChannelGetVoltage.vi"("AIDeviceRef"=w1926) -> ("Voltage"=w1925:dbl)  [unwired: 8 in, 2 out]
        n1165 = Get Date/Time In Seconds() -> (seconds since 1Jan1904=w1922:timestamp)
        n1166 = To Double Precision Float(number=w1922) -> (double precision float=w1921:dbl)
        n1167 = Multiply(x="Sonar Gain 2", y=w1925) -> (x*y=w1923:dbl)
        n1168 = call <userlib>:"Rate_Selective_Filter.vi"("hi limit"=70.0, "lo limit"=0.0, "Time"=w1921, "Distance"=w1923) -> ("Filtered"=w1918:dbl)  [unwired: 3 in, 2 out]
        "Sonar Dist 2" <- w1918
        "Sonar 2" <- w1918
        n1169 = shared-variable ".\\Sensors.lvlib\\Sonar Distance"(w1918) -> ()  [unwired: 1 in, 1 out]
      }
      frame Enabled {
      }
    }
    n1170 = call <vilib>:"WPI_EncoderGet.vi"("EncoderDevRef"=w1917) -> ("Distance"=w1904:dbl, "Rate"=w1909:dbl)  [unwired: 5 in, 4 out]
    n1171 = call <vilib>:"WPI_EncoderGet.vi"("EncoderDevRef"=w1916) -> ("Distance"=w1903:dbl, "Rate"=w1852:dbl)  [unwired: 5 in, 4 out]
    n1172 = Negate(x=w1903) -> (-x=w1883:dbl)
    "Left Drv Encoder 2" <- w1883
    n1173 = Negate(x=w1904) -> (-x=w1882:dbl)
    "Right Drv Encoder 2" <- w1882
    n1174 = shared-variable ".\\Sensors.lvlib\\Right Encoder Rate"(w1909) -> ()  [unwired: 1 in, 1 out]
    n1175 = shared-variable ".\\Sensors.lvlib\\Left Encoder Rate"(w1852) -> ()  [unwired: 1 in, 1 out]
    n1176 = Less?(x=w1852, y="y") -> (x < y?=w1849:bool)
    n1177 = call <userlib>:"Drive_Loop_Gyro_Angle.vi"("Yaw Wind"=w1871, "Drive Loop Cluster"=w1911) -> ()  [unwired: 10 in]
    n1178 = call <userlib>:"Drive_Loop_Encoder_Count.vi"("Distance"=w1883, "Drive Loop Cluster"=w1911) -> ()  [unwired: 10 in]
    n1179 = shared-variable ".\\Sensors.lvlib\\Right Encoder Distance"(w1882) -> ()  [unwired: 1 in, 1 out]
    n1180 = shared-variable ".\\Sensors.lvlib\\Left Encoder"(w1883) -> ()  [unwired: 1 in, 1 out]
    n1181 = Absolute Value(x=w1859) -> (abs(x)=w1856:dbl)
    n1182 = shared-variable ".\\Sensors.lvlib\\Turret IMU Pitch"(w1893) -> ()  [unwired: 1 in, 1 out]
    n1183 = shared-variable ".\\Sensors.lvlib\\Turret IMU Roll"(w1894) -> ()  [unwired: 1 in, 1 out]
    n1184 = shared-variable ".\\Sensors.lvlib\\Turret IMU Yaw Wind"(w1876) -> ()  [unwired: 1 in, 1 out]
    n1185 = Absolute Value(x=w1858) -> (abs(x)=w1855:dbl)
    n1186 = call-poly <vilib>:"NT Write Value.vi"("Numeric"=w1871, "Name"="Body Yaw") -> ()  [unwired: 9 in, 1 out]
    n1187 = Add(x=w1856, y=w1855) -> (x+y=w1857:dbl)
    n1188 = Greater?(x=w1857, y="Numeric") -> (0:w1854:bool)
    n1189 = shared-variable ".\\Sensors.lvlib\\Body IMU Yaw"(w1871) -> ()  [unwired: 1 in, 1 out]
    n1190 = shared-variable ".\\Sensors.lvlib\\Body IMU Roll"(w1886) -> ()  [unwired: 1 in, 1 out]
    n1191 = shared-variable ".\\Sensors.lvlib\\Body IMU Pitch"(w1885) -> ()  [unwired: 1 in, 1 out]
    n1192 = shared-variable ".\\Sensors.lvlib\\BodyYawAbs"(w1875) -> ()  [unwired: 1 in, 1 out]
    n1193 = call <userlib>:"Pulse_Stretch_&_Delay.vi"("In"=w1854, "Width (sec)"="Width (sec)") -> ("Out"=w1850:bool)  [unwired: 3 in]
    "Hit Peg" <- w1850
    n1194 = And(x=w1849, y=w1850) -> (x .and. y?=→"x .and. y?":bool)
    n1195 = Not(x=w1880) -> (.not. x?=w1878:bool)
    n1196 = call-poly <vilib>:"NT Write Value.vi"("Numeric"=w1876, "Name"="Turret Yaw") -> ()  [unwired: 9 in, 1 out]
    n1197 = Not(x=w1879) -> (.not. x?=w1877:bool)
    n1198 = feedback #59(0) -> (w1899:i32)
    n1199 = case shown="0, Default" w1899 {
      tunnel: "ReOpen IMUs 2" -> [w2017 _ _]
      tunnel: [w2026 2 ("t") 0 ("t")] -> w1900
      tunnel: w1897 -> [w2024 w2028 _]
      tunnel: w1898 -> [w2023 w2029 _]
      tunnel: [w2024 w2028 w2031] -> w1896
      tunnel: [w2023 w2029 w2032] -> w1895
      tunnel: w1878 -> [w2022 _ _]
      tunnel: w1877 -> [w2021 _ _]
      frame 0, Default {
        n1200 = shared-variable ".\\OperatorController.lvlib\\Manual Turret?"() -> (w2019:bool)  [unwired: 1 in, 1 out]
        n1201 = Compound Arithmetic op=OR(w2022, w2021) -> (w2020:bool)
        n1202 = feedback-in #60(w2019) -> ()
        n1203 = feedback #60(FALSE ("Boolean")) -> (w2018:bool)
        n1204 = Greater?(x=w2019, y=w2018) -> (0:w2015:bool)
        n1205 = And(x=w2015, y=w2020) -> (x .and. y?=w2013:bool)
        n1206 = Or(x=w2013, y=w2017) -> (x .or. y?=w2014:bool)
        n1207 = Select(t=1, s=w2014, f=0) -> (s? t:f=w2026:i32)
      }
      frame 1 {
        n1208 = call <vilib>:"WPI_I2CClose.vi"("I2CDevRef"=w2028) -> ()  [unwired: 10 in, 1 out]
        n1209 = call <vilib>:"WPI_I2CClose.vi"("I2CDevRef"=w2029) -> ()  [unwired: 10 in, 1 out]
      }
      frame 2 {
        n1210 = call <userlib>:"IMUOrientOpen.vi"("Op Mode"=T57."IMU", "Stored Cal File"="BNO055 Cal M8 P3 01-10-2017 194051", "Status delay"=30, "Alt Adr?"=TRUE) -> ("Occupant"=→"Occupant Alt 2":u8[], "I2CDevRef"=w2049:T33, "Cal Status @ Open"=w2053:T61, "Odd"=→"Odd Alt 2":bool)  [unwired: 6 in, 2 out]
        n1211 = call <userlib>:"IMUOrientOpen.vi"("Op Mode"=T57."IMU", "Stored Cal File"="BNO055 Cal M8 P3 01-10-2017 194050", "Alt Adr?"=FALSE) -> ("Occupant"=→"Occupant Pri 2":u8[], "I2CDevRef"=w2036:T33, "Cal Status @ Open"=w2039:T61, "Odd"=→"Odd Pri 2":bool)  [unwired: 7 in, 2 out]
        n1212 = call <userlib>:"IMUOrientRefNum Registry Set.vi"("refnum name"="BodyPrime", "I2CDevRef in"=w2049) -> ("I2CDevRef out"=w2031:T33)  [unwired: 8 in, 1 out]
        n1213 = call <userlib>:"IMUOrientRefNum Registry Set.vi"("refnum name"="TurretPrime", "I2CDevRef in"=w2036) -> ("I2CDevRef out"=w2032:T33)  [unwired: 8 in, 1 out]
        n1214 = Unbundle(w2053) -> ("Cluster"=→"S 6":T60, "Cluster"=→"G 6":T60, "Cluster"=→"A 6":T60, "Cluster"=→"M 6":T60)
        n1215 = Unbundle(w2039) -> ("Cluster"=→"S 7":T60, "Cluster"=→"G 7":T60, "Cluster"=→"A 7":T60, "Cluster"=→"M 7":T60)
      }
    }
    n1216 = feedback-in #59(w1900) -> ()
    n1217 = node-c288("Sensor Loop Period 2") -> ()  [unwired: 1 out]
  }
  n1218 = while "Drive Logging Loop" {
    tunnel: w77 -> [w2071]
    tunnel: w76 -> [w2070]
    tunnel: w69 -> [w2065]
    stop <- FALSE stop-if-true
    n1219 = local read "Save Drive"() -> (w2068:bool)
    n1220 = local read "Burst"() -> (w2066:i32)
    n1221 = call "Drive Data Logger.vi"("Save"=w2068, "Array"=w2070, "Burst"=w2066, "rt fifo"=w2071, "TDMS Refnum"=w2065) -> ()  [unwired: 7 in]
    n1222 = Wait (ms)(milliseconds to wait="loop period (ms) 2") -> ()  [unwired: 1 out]
  }
  n1223 = Get Date/Time In Seconds() -> (seconds since 1Jan1904=w68:timestamp)
  n1224 = To Double Precision Float(number=w68) -> (double precision float=w67:dbl)
  n1225 = while {
    tunnel: w77 -> [w2077]
    tunnel: w76 -> [w2076]
    tunnel: w67 -> [w2075]
    stop <- FALSE stop-if-true
    n1226 = Wait (ms)(milliseconds to wait=u32 40) -> ()  [unwired: 1 out]
    n1227 = case shown="True" TRUE {
      tunnel: w2076 -> [_ w2119]
      tunnel: w2075 -> [_ w2118]
      tunnel: w2077 -> [_ w2117]
      frame False {
      }
      frame True {
        (unwired) 1 ("index")
        (unwired) 0 ("index")
        n1228 = shared-variable ".\\ToLog.lvlib\\Distance (lateral) 1"() -> (w2080:dbl)  [unwired: 1 in, 1 out]
        n1229 = shared-variable ".\\ToLog.lvlib\\BotShooterCtrl"() -> (w2082:dbl)  [unwired: 1 in, 1 out]
        n1230 = shared-variable ".\\ToLog.lvlib\\Distance (lateral) 2"() -> (w2079:dbl)  [unwired: 1 in, 1 out]
        n1231 = shared-variable ".\\ToLog.lvlib\\BotShooterResponse"() -> (w2081:dbl)  [unwired: 1 in, 1 out]
        n1232 = shared-variable ".\\ToLog.lvlib\\TopShooterResponse"() -> (w2083:dbl)  [unwired: 1 in, 1 out]
        n1233 = shared-variable ".\\ToLog.lvlib\\roboRIO input voltage (V)"() -> (w2111:dbl)  [unwired: 1 in, 1 out]
        n1234 = shared-variable ".\\Vision Variables.lvlib\\Gear yaw delta"() -> (w2092:dbl)  [unwired: 1 in, 1 out]
        n1235 = shared-variable ".\\Sensors.lvlib\\Left Encoder"() -> (w2086:dbl)  [unwired: 1 in, 1 out]
        n1236 = shared-variable ".\\ToLog.lvlib\\TopShooterCtrl"() -> (w2084:dbl)  [unwired: 1 in, 1 out]
        n1237 = shared-variable ".\\Sensors.lvlib\\Right Encoder Distance"() -> (w2085:dbl)  [unwired: 1 in, 1 out]
        n1238 = shared-variable ".\\Vision Variables.lvlib\\Gear valid"() -> (w2091:bool)  [unwired: 1 in, 1 out]
        n1239 = shared-variable ".\\ToLog.lvlib\\Robot Mode"() -> (w2112:T62)  [unwired: 1 in, 1 out]
        n1240 = Get Date/Time In Seconds() -> (seconds since 1Jan1904=w2122:timestamp)
        n1241 = shared-variable ".\\Sensors.lvlib\\Turret IMU Yaw Wind"() -> (w2087:dbl)  [unwired: 1 in, 1 out]
        n1242 = shared-variable ".\\Vision Variables.lvlib\\Gear Distance"() -> (w2093:dbl)  [unwired: 1 in, 1 out]
        n1243 = shared-variable ".\\ToLog.lvlib\\TurretBuGood"() -> (w2107:bool)  [unwired: 1 in, 1 out]
        n1244 = shared-variable ".\\Sensors.lvlib\\Body IMU Yaw"() -> (w2088:dbl)  [unwired: 1 in, 1 out]
        n1245 = shared-variable ".\\ControlMode.lvlib\\ShootingMode"() -> (w2102:bool)  [unwired: 1 in, 1 out]
        n1246 = shared-variable ".\\ToLog.lvlib\\BodyBuGood"() -> (w2109:bool)  [unwired: 1 in, 1 out]
        n1247 = shared-variable ".\\ToLog.lvlib\\TurretPriGood"() -> (w2108:bool)  [unwired: 1 in, 1 out]
        n1248 = shared-variable ".\\ToLog.lvlib\\BodyPriGood"() -> (w2110:bool)  [unwired: 1 in, 1 out]
        n1249 = shared-variable ".\\ToLog.lvlib\\TurretBump"() -> (w2098:dbl)  [unwired: 1 in, 1 out]
        n1250 = shared-variable ".\\Vision Variables.lvlib\\Boiler Yaw delta"() -> (w2096:dbl)  [unwired: 1 in, 1 out]
        n1251 = shared-variable ".\\ToLog.lvlib\\ShooterTopBumps"() -> (w2099:dbl)  [unwired: 1 in, 1 out]
        n1252 = shared-variable ".\\Vision Variables.lvlib\\Boiler Found"() -> (w2095:bool)  [unwired: 1 in, 1 out]
        n1253 = shared-variable ".\\ToLog.lvlib\\ShooterBotBumps"() -> (w2100:dbl)  [unwired: 1 in, 1 out]
        n1254 = shared-variable ".\\Vision Variables.lvlib\\Boiler Distance Averaged"() -> (w2097:dbl)  [unwired: 1 in, 1 out]
        n1255 = shared-variable ".\\ToLog.lvlib\\Auto State"() -> (w2089:T63)  [unwired: 1 in, 1 out]
        n1256 = To Double Precision Float(number=w2122) -> (double precision float=w2123:dbl)
        n1257 = Subtract(x=w2123, y=w2118) -> (x-y=w2115:dbl)
        n1258 = Boolean To (0,1)(Boolean=w2091) -> (0, 1=w2090:i16)
        n1259 = Boolean To (0,1)(Boolean=w2109) -> (0, 1=w2105:i16)
        n1260 = Boolean To (0,1)(Boolean=w2108) -> (0, 1=w2104:i16)
        n1261 = Boolean To (0,1)(Boolean=w2107) -> (0, 1=w2103:i16)
        n1262 = Boolean To (0,1)(Boolean=w2102) -> (0, 1=w2101:i16)
        n1263 = Boolean To (0,1)(Boolean=w2110) -> (0, 1=w2106:i16)
        n1264 = Boolean To (0,1)(Boolean=w2095) -> (0, 1=w2094:i16)
        n1265 = feedback #61(u32 0 ("# elements")) -> (w2078:u32)
        n1266 = Replace Array Subset(array=w2119, new element #1=w2115, new element #2=w2112, new element #3=w2111, new element #4=w2106, new element #5=w2105, new element #6=w2104, new element #7=w2103, new element #8=w2101, new element #9=w2100, new element #10=w2099, new element #11=w2098, new element #12=w2097, new element #13=w2096, new element #14=w2094, new element #15=w2093, new element #16=w2092, new element #17=w2090, new element #18=w2089, new element #19=w2088, new element #20=w2087, new element #21=w2086, new element #22=w2085, new element #23=w2084, new element #24=w2083, new element #25=w2082, new element #26=w2081, new element #27=w2080, new element #28=w2079, new element #29=w2078) -> (w2120:dbl[])  [unwired: 29 in]
        n1267 = RT FIFO Write(0:w2117, 1:w2120) -> (7:w2116:u32)  [unwired: 3 in, 3 out]
        n1268 = Greater?(x=w2116, y="Burst") -> (0:→"Save Drive 2" →"Save Drive":bool)
        n1269 = feedback-in #61(w2116) -> ()
      }
    }
  }
  n1270 = node-c288(w23) -> ()  [unwired: 1 out]
